vi "输出数据解析.vi"(0 "主板引用":refnum<vi>, 1 "从板引用":refnum<vi>, 2 "板选择":enum16{"主板", "从板"}(ring), 3 "二维码信息":refnum<vi>, 5 "错误代码":i32, 7 "命令序号":u8, 9 "输入数组":u8[](array[numeric]), 11 "命令":u8 format="%x", 12 "进度引用":refnum<vi>, 13 "从板个数":refnum<vi>, 14 "从板二维码信息":refnum<vi>) -> (4 "从板数":u8, 10 "序号":u8, 15 "状态":bool)   [LabVIEW 2013]
panel:
  in  "从板个数 2":dbl=1.0
  out "子字符串之前":string
  out "从板信息":T1
  out "主板数据 2":T2
  out "充电控制参数":bool
  out "二级故障1 2":bool
  out "一级故障1 6":bool
  out "一级故障1 5":bool
  out "二级故障1":bool
  out "一级故障5":bool
  out "一级故障1 4":bool
  out "一级故障1 3":bool
  out "一级故障1 2":bool
  out "一级故障1":bool
  in  "Ctl引用句柄":refnum<vi>
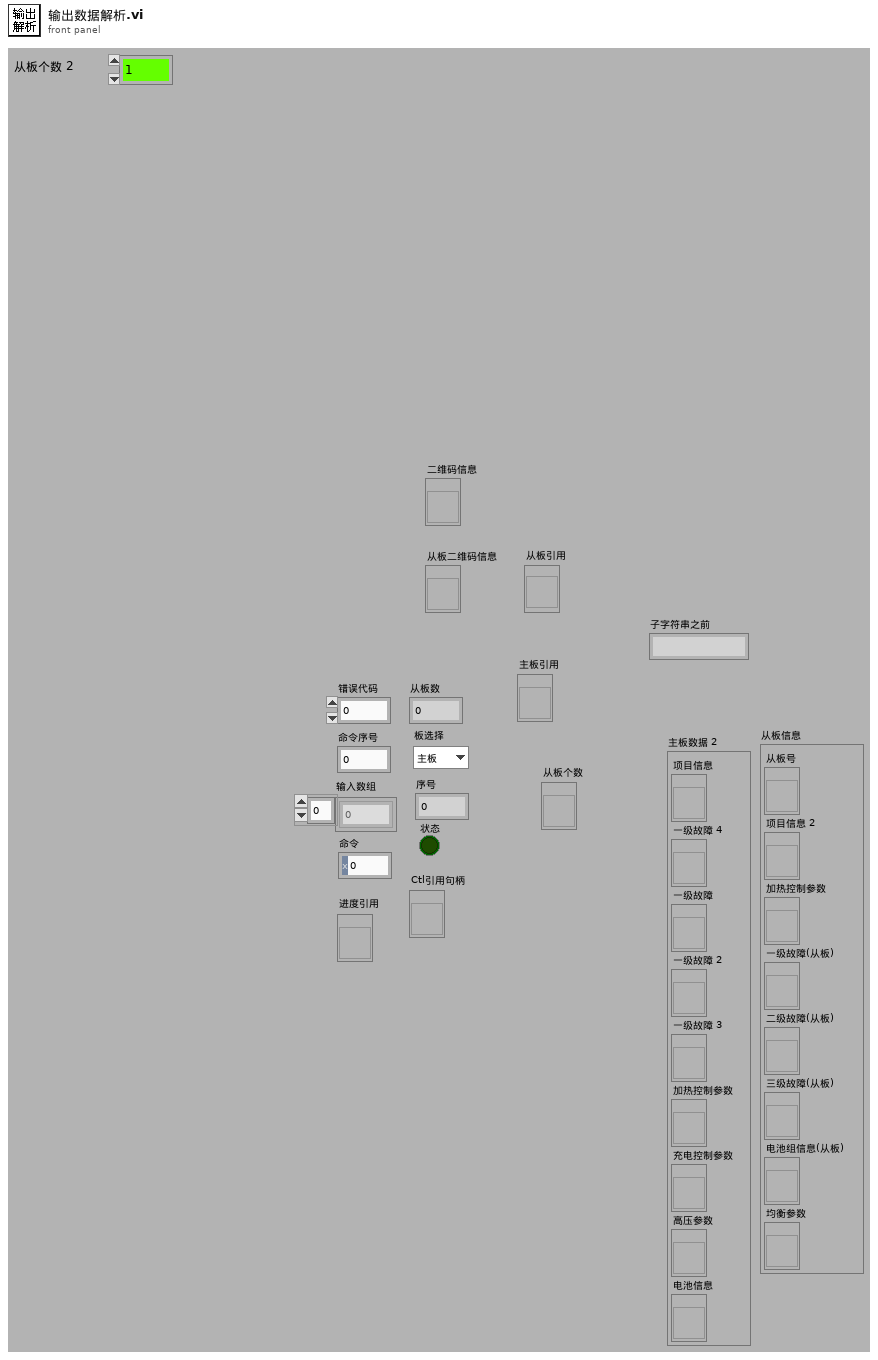
[diagram p1: front panel]
types:
  T1 = cluster{"从板号":refnum<vi>, "项目信息 2":refnum<vi>, "加热控制参数":refnum<vi>, "一级故障(从板)":refnum<vi>, "二级故障(从板)":refnum<vi>, "三级故障(从板)":refnum<vi>, "电池组信息(从板)":refnum<vi>, "均衡参数":refnum<vi>}
  T2 = cluster{"项目信息":refnum<vi>, "一级故障 4":refnum<vi>, "一级故障":refnum<vi>, "一级故障 2":refnum<vi>, "一级故障 3":refnum<vi>, "加热控制参数":refnum<vi>, "充电控制参数":refnum<vi>, "高压参数":refnum<vi>, "电池信息":refnum<vi>}
  T3 = cluster{"电池额定容量":dbl, "使用者":dbl, "电池实际容量":dbl, "车牌号":string, "配置文件版本":string, "SOH":dbl, "SOC":dbl, "产品编号":string, "系统时钟":string}
  T4 = cluster{"电池额定容量(A)":dbl, "使用者":dbl, "电池实际容量(A)":dbl, "车架(牌)号":string, "配置文件版本":string, "SOH(%)":dbl, "SOC(%)":dbl, "产品编号":string, "系统时钟":string}
  T5 = cluster{"总电压过高":dbl, "整组电压不均衡":dbl, "SOC过高":dbl, "单体电压过高":dbl, "总电压过低":dbl, "温度过高":dbl, "温度过低":dbl, "单组电压不均衡":dbl, "整组温度不均衡":dbl, "单组温度不均衡":dbl, "单体电压过低":dbl, "充电电流过高":dbl, "放电电流过高":dbl, "SOC过低":dbl, "内阻过大":dbl, "极柱温度过高":dbl, "SOH过低":dbl}
  T6 = cluster{"风机开启温度":dbl, "风机关闭温度":dbl, "加热开启温度":dbl, "加热关闭温度":dbl, "风机开启温差":dbl, "风机关闭温差":dbl, "加热关闭温差":dbl}
  T7 = cluster{"最大允许单体电压":dbl, "最大允许总电压":dbl, "最小允许单体电压":dbl, "最大允许充电电流":dbl, "最小允许充电电流":dbl, "最大允许充电温度":dbl, "最小允许充电温度":dbl, "电流步长":dbl}
  T8 = cluster{"充电能量阀值":dbl, "放电能量阀值":dbl, "电流增益":dbl, "平均电流":dbl, "电压增益":dbl, "平均电压":dbl}
  T9 = cluster{"电池串联":dbl, "电池并联":dbl, "累计放电总安时":dbl, "电池包额定容量":dbl, "电池包额定能量":dbl, "电池包额定总电压":dbl, "累计充电总安时":dbl, "电池充满次数":dbl, "电池放空次数":dbl, "电池充电次数":dbl, "电池生产日期":string, "电池厂家":string, "电池类型":string, "电池包组号":string, "电池包产权标识":string, "电池应用车型":string, "实际容量":dbl}
  T10 = cluster{"电压过高":dbl, "电压过低":dbl, "温度过高":dbl, "温度过低":dbl, "电压不均衡(V)":dbl, "温度不均衡":dbl, "SOC过低":dbl}
  T11 = cluster{"串联数":dbl, "并联数":dbl, "电池厂家":dbl, "电池类型":dbl, "额定能量":dbl, "额定容量":dbl, "实际容量":dbl, "额定总压":dbl, "产权标识":dbl, "应用车型":dbl, "电池包组号":dbl, "SOC":dbl, "充电总安时":dbl, "放电总这时":dbl, "放空次数":dbl, "充满次数":dbl, "充电次数":dbl, "车牌号":string, "生产日期":string, "最大允许单体电压":dbl, "最大允许总电压":dbl, "最大允许温度":dbl, "最小允许温度":dbl, "最大允许充电电流":dbl, "最小允许充电电流":dbl, "最小允许单体电压":dbl, "电流步长":dbl, "电池包序号":dbl}
  T12 = cluster{"充电结束电压(90%)":sgl, "充电结束电压(91%)":sgl, "充电结束电压(92%)":sgl, "充电结束电压(93%)":sgl, "充电结束电压(94%)":sgl, "均衡计算-电压高阀值1级":sgl, "均衡计算-电压高阀值2级":sgl, "均衡计算-电压低阀值1级":sgl, "均衡计算-电压低阀值2级":sgl, "均衡计算-最低电压阀值":sgl, "均衡停止-最低电压阀值":sgl, "均衡计算-电压极差阀值":sgl, "充电结束电压(95%)":sgl, "充电结束电压(96%)":sgl, "充电结束电压(97%)":sgl, "充电结束电压(98%)":sgl, "充电结束电压(99%)":sgl, "充电结束电压(100%)":sgl}
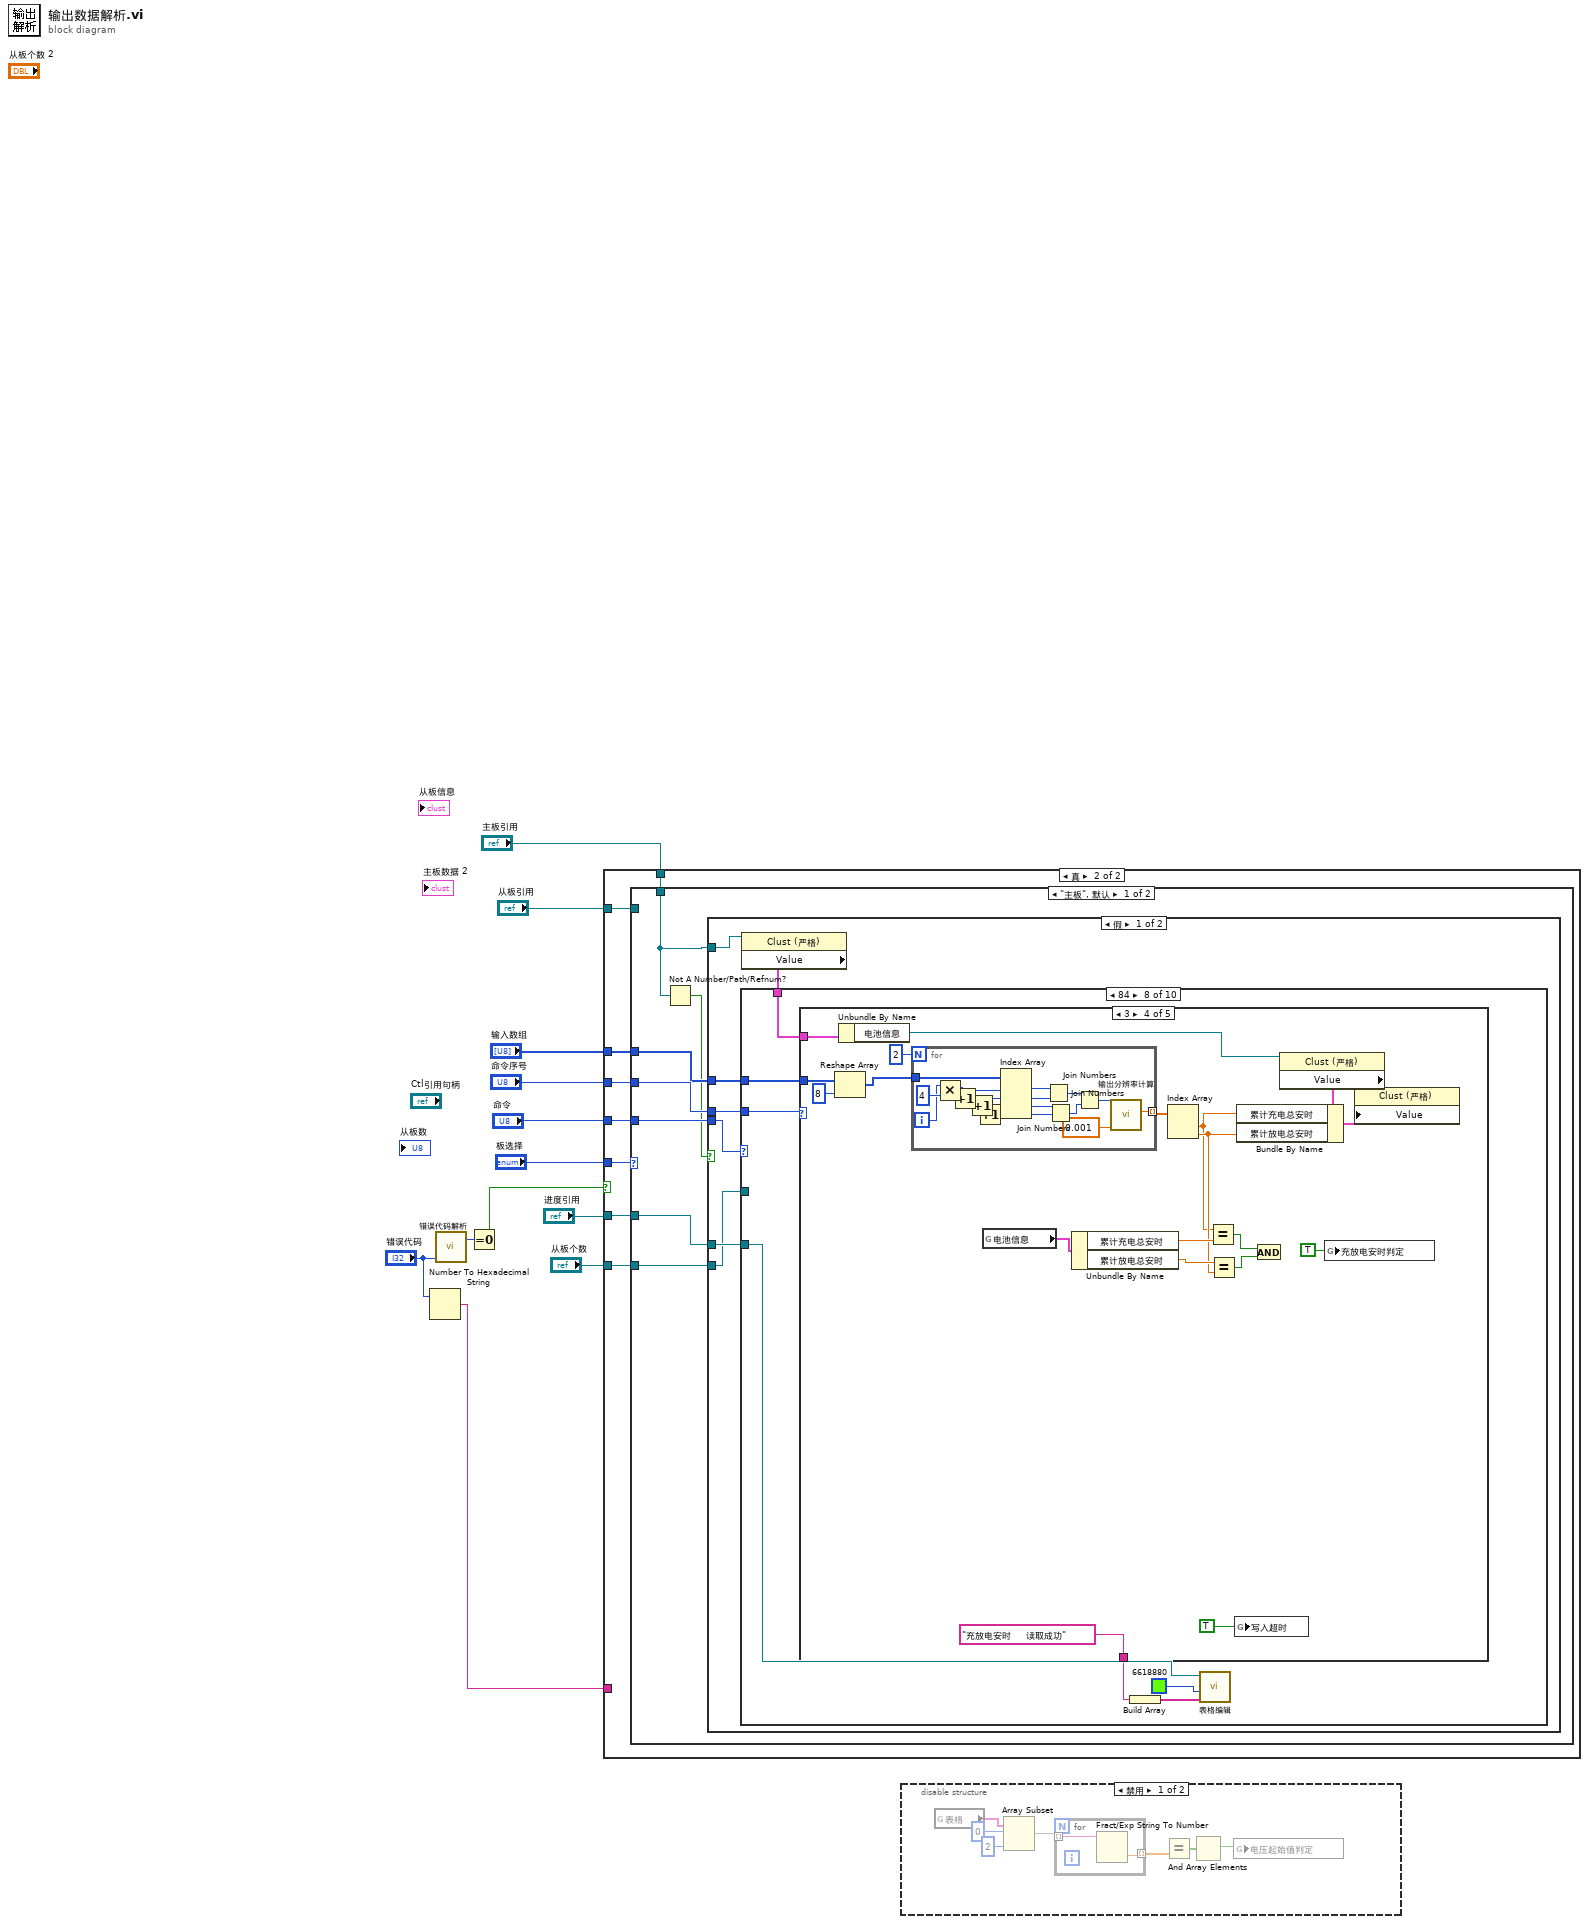
[diagram p0: block diagram]
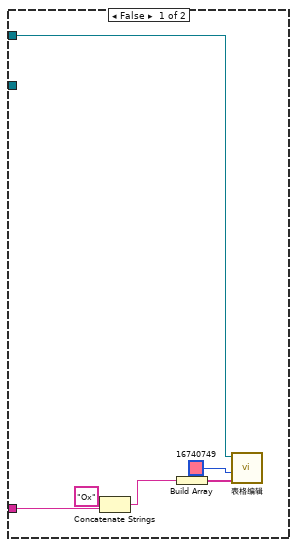
[diagram p3: hidden frame]
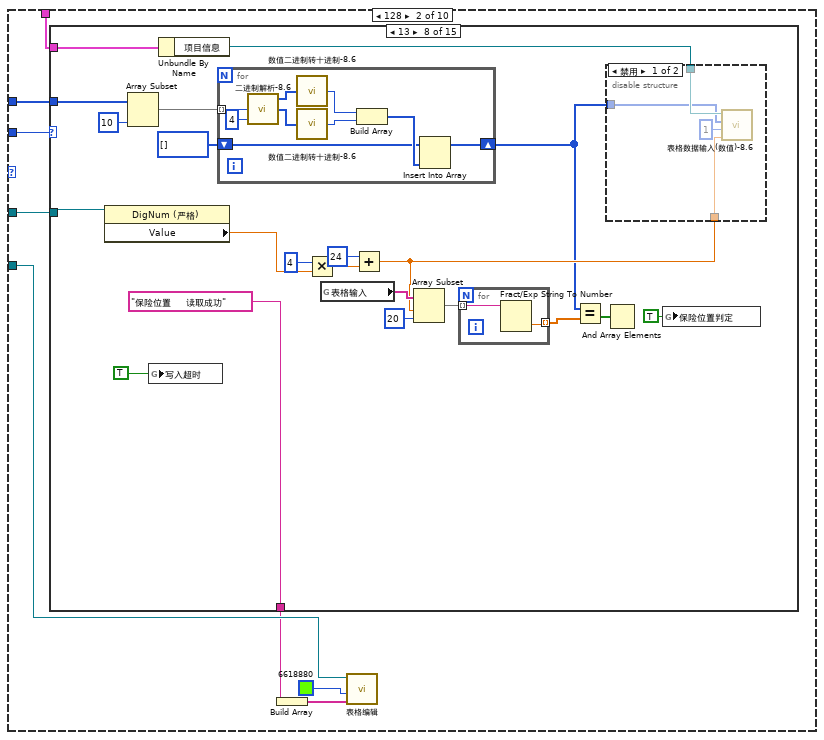
[diagram p5: hidden frame]
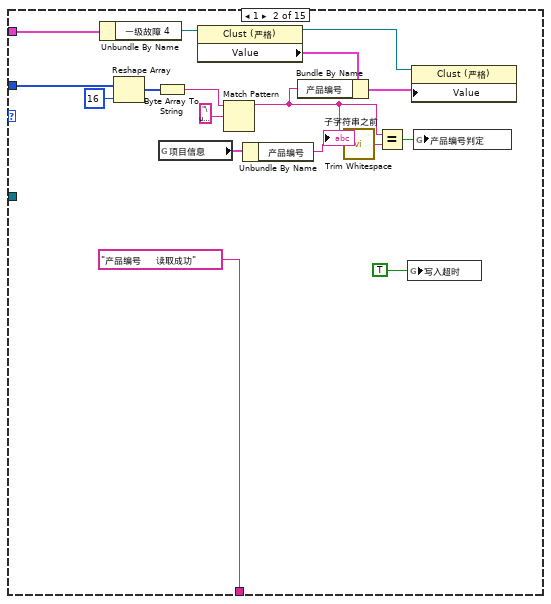
[diagram p7: hidden frame]
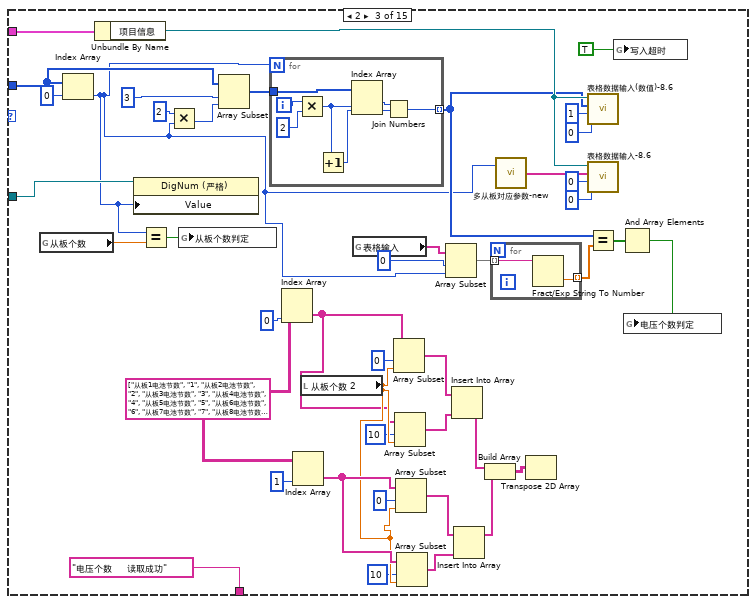
[diagram p8: hidden frame]
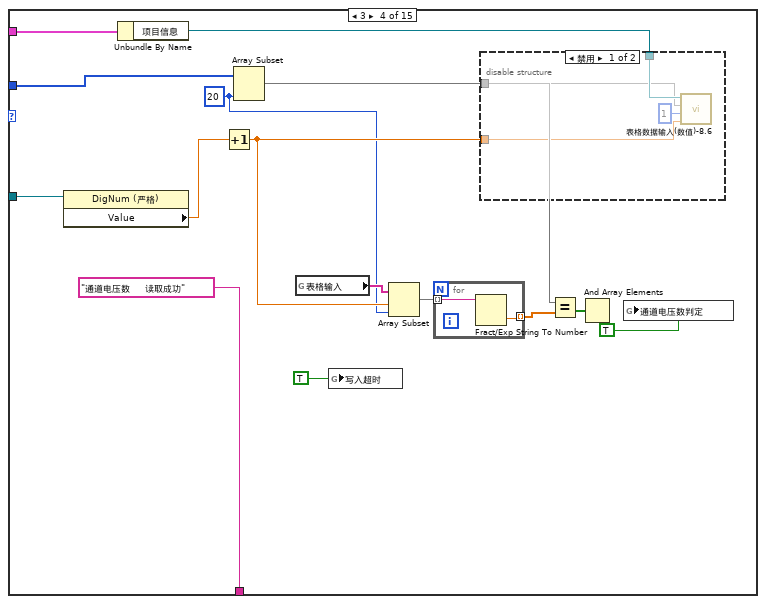
[diagram p9: hidden frame]
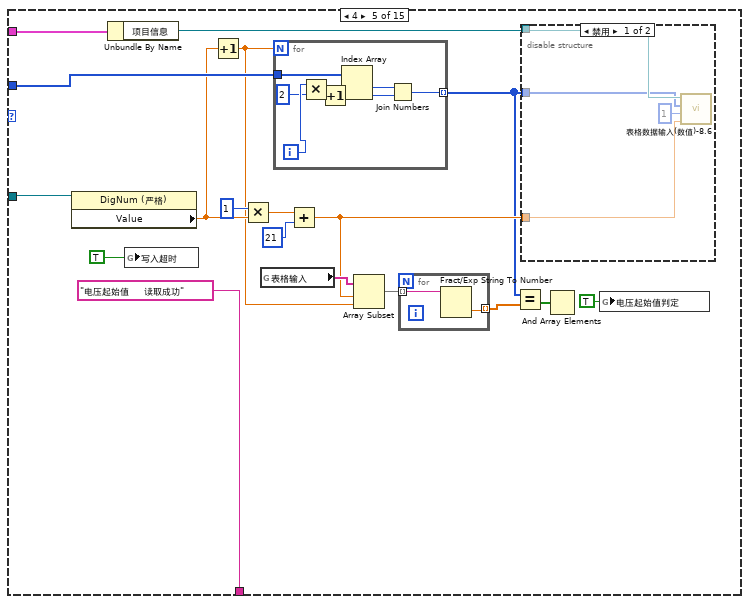
[diagram p11: hidden frame]
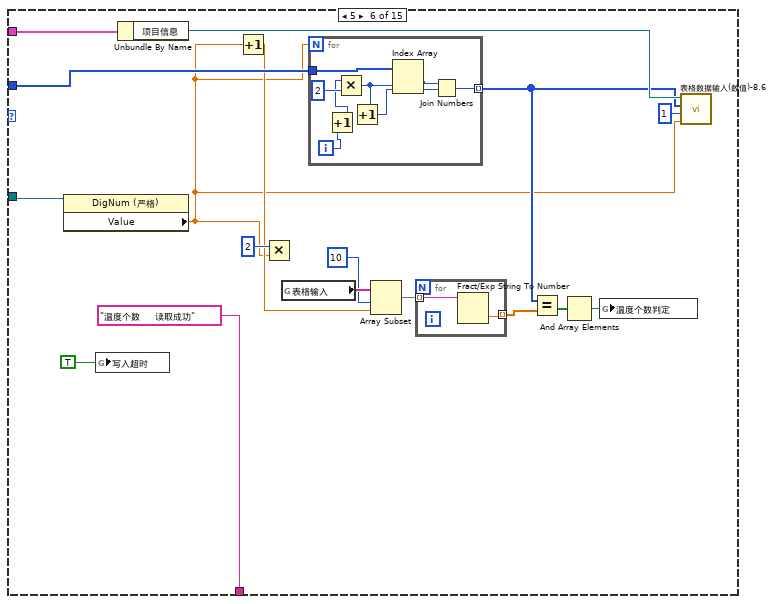
[diagram p13: hidden frame]
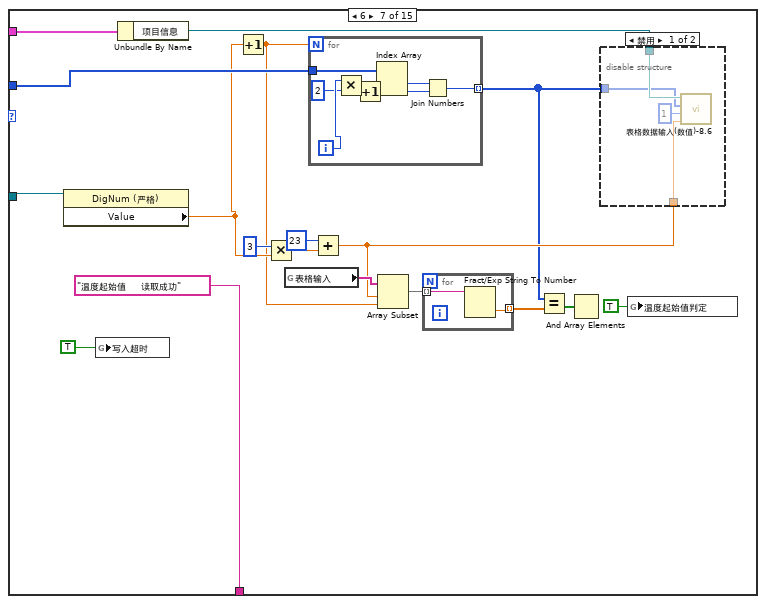
[diagram p14: hidden frame]
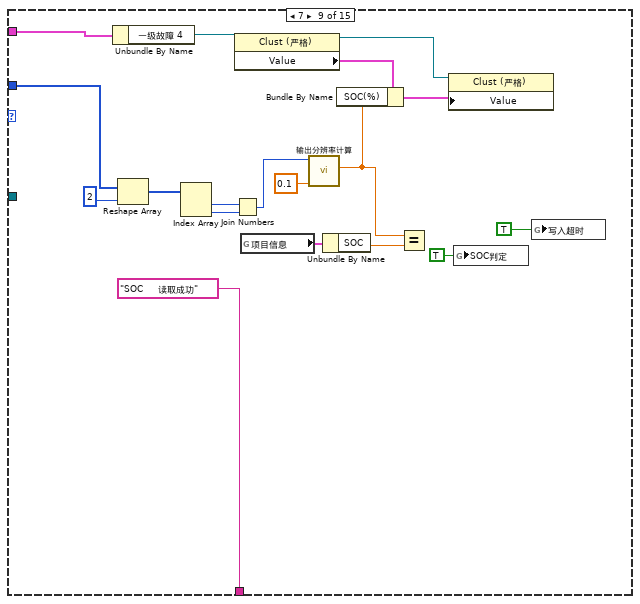
[diagram p17: hidden frame]
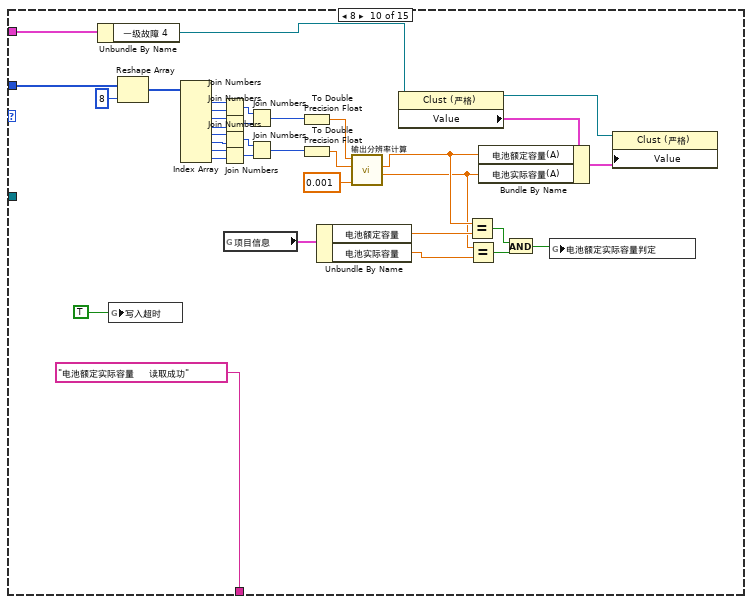
[diagram p18: hidden frame]
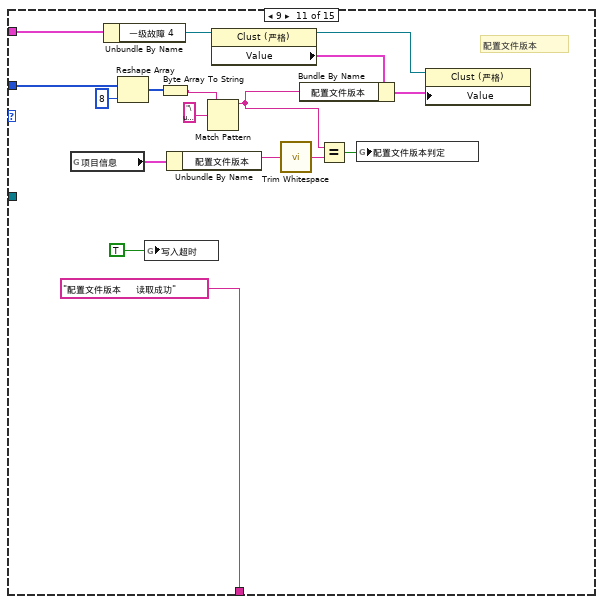
[diagram p19: hidden frame]
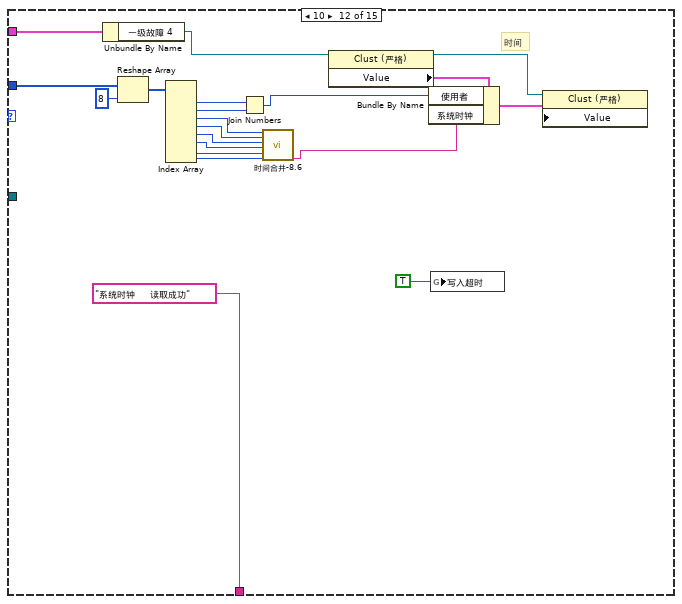
[diagram p20: hidden frame]
diagram:
  n1 = Number To Hexadecimal String(2:"错误代码") -> (0:w2:string)  [unwired: 1 out]
  n2 = call "错误代码解析.vi"("错误代码"="错误代码") -> ("错误代码"=w12:i32)  [unwired: 2 out]
  n3 = Equal To 0?(x=w12) -> (x = 0?=w11:bool)
  n4 = case shown="真" w11 {
    tunnel: "命令" -> [_ w26]
    tunnel: "命令序号" -> [_ w25]
    tunnel: "输入数组" -> [_ w24]
    tunnel: "板选择" -> [_ w23]
    tunnel: "主板引用" -> [_ w22]
    tunnel: "从板引用" -> [_ w21]
    tunnel: "进度引用" -> [w14 w20]
    tunnel: w2 -> [w17 _]
    tunnel: "从板个数" -> [_ w19]
    frame False {
      n5 = Concatenate Strings("Ox" ("字符串"), w17) -> (w16:string)
      n6 = Build Array(w16) -> (w15:string[])
      n7 = call "表格编辑.vi"("新元素/子数组"=w15, "活动单元格:单元格背景色"=u32 16740749, "MCListbox引用句柄"=w14) -> ()  [unwired: 9 out]
    }
    frame True {
      n8 = case shown="\"主板\", 默认" w23 {
        tunnel: w26 -> [w33 w1787]
        tunnel: w25 -> [w32 w1786]
        tunnel: w24 -> [w31 w1785]
        tunnel: w22 -> [w28 _]
        tunnel: w21 -> [_ w1783]
        tunnel: w20 -> [w30 w1784]
        tunnel: w19 -> [w27 _]
        frame "主板", Default {
          n9 = Not A Number/Path/Refnum?(number/path/refnum=w28) -> (NaN/Path/Refnum?=w29:bool)
          n10 = case shown="假" w29 {
            tunnel: w33 -> [w40 _]
            tunnel: w32 -> [w39 _]
            tunnel: w31 -> [w38 _]
            tunnel: w28 -> [w37 _]
            tunnel: w30 -> [w35 _]
            tunnel: w27 -> [w34 _]
            frame False {
              n11 = property class="Clust (严格)"(reference=w37) -> ("Value"=w36:T2)  [unwired: 1 in, 2 out]
              n12 = case shown="84" w40 {
                tunnel: w39 -> [_ w48 w413 w1115 w1300 w1346 w1388 w1560 _ _]
                tunnel: w38 -> [_ w47 w412 w1114 w1299 w1345 w1387 w1559 w1769 w1780]
                tunnel: w36 -> [_ w46 w411 w1113 w1298 w1344 _ w1558 _ _]
                tunnel: w35 -> [_ w44 w410 w1112 w1297 w1343 _ w1555 _ w1773]
                tunnel: w34 -> [_ w42 _ _ _ _ _ _ _ _]
                frame 0, Default {
                }
                frame 128 {
                  n13 = case shown="13" w48 {
                    tunnel: w47 -> [_ w65 w100 w133 w152 w184 w212 w243 w285 w320 w337 w357 w374 w391 w407]
                    tunnel: w46 -> [_ w62 w102 w132 w155 w186 w215 w250 w282 w317 w334 w351 w368 w385 w402]
                    tunnel: w42 -> [_ _ w97 w130 w151 w183 w211 w247 _ _ _ _ _ _ _]
                    tunnel: [_ "产品编号     读取成功" ("字符串") "电压个数     读取成功" ("字符串") "通道电压数     读取成功" ("字符串") "电压起始值     读取成功" ("字符串") "温度个数     读取成功" ("字符串") "温度起始值     读取成功" ("字符串") "保险位置     读取成功" ("字符串") "SOC     读取成功" ("字符串") "电池额定实际容量     读取成功" ("字符串") "配置文件版本     读取成功" ("字符串") "系统时钟     读取成功" ("字符串") "校正时钟     读取成功" ("字符串") "车牌号     读取成功" ("字符串") "SOH     读取成功" ("字符串")] -> w41
                    frame 0, Default {
                    }
                    frame 1 {
                      n14 = Unbundle By Name(w62) -> ("一级故障 4"=w61:refnum<vi>)
                      n15 = Reshape Array(w65, 16 ("维数大小")) -> (w64:u8[])
                      n16 = Byte Array To String(unsigned byte array=w64) -> (string=w50:string)
                      n17 = global read "读配置文件全局.vi" "项目信息"() -> (w56:T3)
                      n18 = property class="Clust (严格)"(reference=w61) -> (reference out=w59:refnum<vi>, "Value"=w60:T4)  [unwired: 1 in, 1 out]
                      n19 = Match Pattern(string=w50, regular expression="\u0000" ("trimmed string")) -> (before substring=w49:string)  [unwired: 1 in, 3 out]
                      "子字符串之前" <- w49
                      n20 = Unbundle By Name(w56) -> ("产品编号"=w54:string)
                      n21 = Bundle By Name(cluster=w60, "产品编号"=w49) -> (w55:T4)
                      n22 = call <vilib>:"Trim Whitespace.vi"("string"=w54) -> ("trimmed string"=w52:string)  [unwired: 1 in]
                      n23 = Equal?(x=w49, y=w52) -> (x = y?=w53:bool)
                      n24 = global write "EV05全局变量1.vi" "写入超时"(TRUE ("写入超时")) -> ()
                      n25 = property class="Clust (严格)"(reference=w59, "Value"=w55) -> ()  [unwired: 1 in, 2 out]
                      n26 = global write "读配置文件全局.vi" "产品编号判定"(w53) -> ()
                    }
                    frame 2 {
                      w74 = string[][] [["从板1电池节数", "1"], ["从板2电池节数", "2"], ["从板3电池节数", "3"], ["从板4电池节数", "4"], ["从板5电池节数", "5"], ["从板6电池节数", "6"], ["从板7电池节数", "7"], ["从板8电池节数", "8"], ["从板9电池节数", "9"], ["从板10电池节数", "10"], ["从板1温度个数", "1"], ["从板2温度个数", "2"], ["从板3温度个数", "3"], ["从板4温度个数", "4"], ["从板5温度个数", "5"], ["从板6温度个数", "6"], ["从板7温度个数", "7"], ["从板8温度个数", "8"], ["从板9温度个数", "9"], ["从板10温度个数", "10"]] ("项目信息")
                      n27 = global read "读配置文件全局.vi" "从板个数"() -> (w94:dbl)
                      n28 = Index Array(array=w100, index=0 ("索引")) -> (element=w67:u8)
                      n29 = Unbundle By Name(w102) -> ("项目信息"=w101:refnum<vi>)
                      n30 = property class="DigNum (严格)"(reference=w97, "Value"=w67) -> ()  [unwired: 1 in, 2 out]
                      n31 = Equal?(x=w67, y=w94) -> (x = y?=w93:bool)
                      n32 = Multiply(x=u8 2, y=w67) -> (x*y=w85:u8)
                      n33 = global write "读配置文件全局.vi" "从板个数判定"(w93) -> ()
                      n34 = Array Subset(array=w100, index=u8 3 ("y"), length=w85) -> (w99:u8[])
                      n35 = for {
                        N: w67 -> [_]
                        tunnel: w99 -> [w118]
                        tunnel: [w111] -> w88 mode=indexing
                        i -> [w117]
                        n36 = Multiply(x=w117, y=2) -> (x*y=w115:i32)
                        n37 = Increment(x=w115) -> (x+1=w114:i32)
                        n38 = Index Array(array=w118, index #1=w115, index #2=w114) -> (element #1=w112:u8, element #2=w113:u8)
                        n39 = Join Numbers(hi=w112, lo=w113) -> ((hi.lo)=w111:u16)
                      }
                      n40 = Index Array(array=w74, index (col)=0 ("索引 (行)")) -> (element=w71:string[])  [unwired: 1 in]
                      n41 = Index Array(array=w74, index (col)=1 ("禁用的索引 (列)")) -> (element=w81:string[])  [unwired: 1 in]
                      n42 = local read "从板个数 2"() -> (w79:dbl)
                      n43 = global read "读配置文件全局.vi" "表格输入"() -> (w92:string[])
                      n44 = Array Subset(array=w71, index=0 ("索引"), length=w79) -> (w72:string[])
                      n45 = Array Subset(array=w71, index=10 ("索引"), length=w79) -> (w73:string[])
                      n46 = Array Subset(array=w81, index=0 ("索引"), length=w79) -> (w75:string[])
                      n47 = Array Subset(array=w81, index=10 ("索引"), length=w79) -> (w80:string[])
                      n48 = Array Subset(array=w92, index=0 ("索引"), length=w67) -> (w90:string[])
                      n49 = Insert Into Array(array=w72, new element=w73) -> (w82:string[])  [unwired: 1 in]
                      n50 = Insert Into Array(array=w75, new element=w80) -> (w83:string[])  [unwired: 1 in]
                      n51 = Build Array(w82, w83) -> (w84:string[][])
                      n52 = for {
                        tunnel: w90 -> [w110] mode=indexing
                        tunnel: [w109] -> w89 mode=indexing
                        n53 = Fract/Exp String To Number(string=w110) -> (number=w109:dbl)  [unwired: 4 out]
                      }
                      n54 = call "多从板对应参数-new.vi"("从板个数"=w67) -> ("输出数组"=w105:string[])  [unwired: 1 in]
                      n55 = Transpose 2D Array(2D array=w84) -> ()  [unwired: 1 out]
                      n56 = call "表格数据输入(数值)-8.6.vi"("行数"=u32 0, "列数"=u32 1, "数值数组"=w88, "表格引用"=w101) -> ()  [unwired: 8 out]
                      n57 = call "表格数据输入-8.6.vi"("行数"=u32 0, "列数"=u32 0, "字符串数组"=w105, "表格引用"=w101) -> ()  [unwired: 8 out]
                      n58 = Equal?(x=w88, y=w89) -> (x = y?=w87:bool[])
                      n59 = global write "EV05全局变量1.vi" "写入超时"(TRUE ("写入超时")) -> ()
                      n60 = And Array Elements(Boolean array=w87) -> (logical AND=w86:bool)
                      n61 = global write "读配置文件全局.vi" "电压个数判定"(w86) -> ()
                    }
                    frame 3 {
                      w123 = 20 ("长度")
                      n62 = property class="DigNum (严格)"(reference=w130) -> ("Value"=w129:dbl)  [unwired: 1 in, 2 out]
                      n63 = Unbundle By Name(w132) -> ("项目信息"=w131:refnum<vi>)
                      n64 = Increment(x=w129) -> (x+1=w124:dbl)
                      n65 = Array Subset(array=w133, length=w123) -> (w121:u8[])  [unwired: 1 in]
                      n66 = global read "读配置文件全局.vi" "表格输入"() -> (w126:string[])
                      n67 = global write "EV05全局变量1.vi" "写入超时"(TRUE ("写入超时")) -> ()
                      n68 = Array Subset(array=w126, index=w124, length=w123) -> (w125:string[])
                      n69 = for {
                        tunnel: w125 -> [w139] mode=indexing
                        tunnel: [w138] -> w122 mode=indexing
                        n70 = Fract/Exp String To Number(string=w139) -> (number=w138:dbl)  [unwired: 4 out]
                      }
                      n71 = disable-structure shown="禁用" {
                        disable-tunnel: w131 -> [w136 _]
                        disable-tunnel: w124 -> [w135 _]
                        disable-tunnel: w121 -> [w134 _]
                        frame Disabled {
                          n72 = call "表格数据输入(数值)-8.6.vi"("行数"=w135, "列数"=u32 1, "数值数组"=w134, "表格引用"=w136) -> ()  [unwired: 8 out]
                        }
                        frame Enabled {
                        }
                      }
                      n73 = Equal?(x=w121, y=w122) -> (x = y?=w120:bool[])
                      n74 = And Array Elements(Boolean array=w120) -> ()  [unwired: 1 out]
                      n75 = global write "读配置文件全局.vi" "通道电压数判定"(TRUE ("通道电压数判定")) -> ()
                    }
                    frame 4 {
                      n76 = property class="DigNum (严格)"(reference=w151) -> ("Value"=w150:dbl)  [unwired: 1 in, 2 out]
                      n77 = Unbundle By Name(w155) -> ("项目信息"=w154:refnum<vi>)
                      n78 = global write "EV05全局变量1.vi" "写入超时"(TRUE ("写入超时")) -> ()
                      n79 = Increment(x=w150) -> (x+1=w142:dbl)
                      n80 = Multiply(x=u8 1, y=w150) -> (x*y=w156:dbl)
                      n81 = global read "读配置文件全局.vi" "表格输入"() -> (w147:string[])
                      n82 = for {
                        N: w142 -> [_]
                        tunnel: w152 -> [w171]
                        tunnel: [w164] -> w141 mode=indexing
                        i -> [w170]
                        n83 = Multiply(x=w170, y=2) -> (x*y=w168:i32)
                        n84 = Increment(x=w168) -> (x+1=w167:i32)
                        n85 = Index Array(array=w171, index #1=w168, index #2=w167) -> (element #1=w165:u8, element #2=w166:u8)
                        n86 = Join Numbers(hi=w165, lo=w166) -> ((hi.lo)=w164:u16)
                      }
                      n87 = Add(x=w156, y=u8 21) -> (x+y=w143:dbl)
                      n88 = Array Subset(array=w147, index=w143, length=w142) -> (w146:string[])
                      n89 = for {
                        tunnel: w146 -> [w163] mode=indexing
                        tunnel: [w162] -> w145 mode=indexing
                        n90 = Fract/Exp String To Number(string=w163) -> (number=w162:dbl)  [unwired: 4 out]
                      }
                      n91 = Equal?(x=w141, y=w145) -> (x = y?=w144:bool[])
                      n92 = disable-structure shown="禁用" {
                        disable-tunnel: w154 -> [w160 _]
                        disable-tunnel: w143 -> [w159 _]
                        disable-tunnel: w141 -> [w158 _]
                        frame Disabled {
                          n93 = call "表格数据输入(数值)-8.6.vi"("行数"=w159, "列数"=u32 1, "数值数组"=w158, "表格引用"=w160) -> ()  [unwired: 8 out]
                        }
                        frame Enabled {
                        }
                      }
                      n94 = And Array Elements(Boolean array=w144) -> ()  [unwired: 1 out]
                      n95 = global write "读配置文件全局.vi" "电压起始值判定"(TRUE ("电压起始值判定")) -> ()
                    }
                    frame 5 {
                      n96 = property class="DigNum (严格)"(reference=w183) -> ("Value"=w174:dbl)  [unwired: 1 in, 2 out]
                      n97 = global write "EV05全局变量1.vi" "写入超时"(TRUE ("写入超时")) -> ()
                      n98 = Unbundle By Name(w186) -> ("项目信息"=w185:refnum<vi>)
                      n99 = Increment(x=w174) -> (x+1=w176:dbl)
                      n100 = Multiply(x=u8 2, y=w174) -> ()  [unwired: 1 out]
                      n101 = global read "读配置文件全局.vi" "表格输入"() -> (w180:string[])
                      n102 = for {
                        N: w174 -> [_]
                        tunnel: w184 -> [w199]
                        tunnel: [w193] -> w175 mode=indexing
                        i -> [w192]
                        n103 = Increment(x=w192) -> (x+1=w191:i32)
                        n104 = Multiply(x=w191, y=2) -> (x*y=w197:i32)
                        n105 = Increment(x=w197) -> (x+1=w196:i32)
                        n106 = Index Array(array=w199, index #1=w197, index #2=w196) -> (element #1=w194:u8, element #2=w195:u8)
                        n107 = Join Numbers(hi=w194, lo=w195) -> ((hi.lo)=w193:u16)
                      }
                      n108 = Array Subset(array=w180, index=u8 10 ("x"), length=w176) -> (w179:string[])
                      n109 = for {
                        tunnel: w179 -> [w190] mode=indexing
                        tunnel: [w189] -> w178 mode=indexing
                        n110 = Fract/Exp String To Number(string=w190) -> (number=w189:dbl)  [unwired: 4 out]
                      }
                      n111 = Equal?(x=w175, y=w178) -> (x = y?=w177:bool[])
                      n112 = And Array Elements(Boolean array=w177) -> (logical AND=w172:bool)
                      n113 = global write "读配置文件全局.vi" "温度个数判定"(w172) -> ()
                      n114 = call "表格数据输入(数值)-8.6.vi"("行数"=w174, "列数"=u32 1, "数值数组"=w175, "表格引用"=w185) -> ()  [unwired: 8 out]
                    }
                    frame 6 {
                      n115 = property class="DigNum (严格)"(reference=w211) -> ("Value"=w210:dbl)  [unwired: 1 in, 2 out]
                      n116 = global write "EV05全局变量1.vi" "写入超时"(TRUE ("写入超时")) -> ()
                      n117 = Unbundle By Name(w215) -> ("项目信息"=w214:refnum<vi>)
                      n118 = Increment(x=w210) -> (x+1=w202:dbl)
                      n119 = Multiply(x=u8 3, y=w210) -> (x*y=w216:dbl)
                      n120 = global read "读配置文件全局.vi" "表格输入"() -> (w207:string[])
                      n121 = for {
                        N: w202 -> [_]
                        tunnel: w212 -> [w231]
                        tunnel: [w224] -> w201 mode=indexing
                        i -> [w230]
                        n122 = Multiply(x=w230, y=2) -> (x*y=w228:i32)
                        n123 = Increment(x=w228) -> (x+1=w227:i32)
                        n124 = Index Array(array=w231, index #1=w228, index #2=w227) -> (element #1=w225:u8, element #2=w226:u8)
                        n125 = Join Numbers(hi=w225, lo=w226) -> ((hi.lo)=w224:u16)
                      }
                      n126 = Add(x=u8 23, y=w216) -> (x+y=w203:dbl)
                      n127 = Array Subset(array=w207, index=w203, length=w202) -> (w206:string[])
                      n128 = for {
                        tunnel: w206 -> [w223] mode=indexing
                        tunnel: [w222] -> w205 mode=indexing
                        n129 = Fract/Exp String To Number(string=w223) -> (number=w222:dbl)  [unwired: 4 out]
                      }
                      n130 = Equal?(x=w201, y=w205) -> (x = y?=w204:bool[])
                      n131 = And Array Elements(Boolean array=w204) -> ()  [unwired: 1 out]
                      n132 = disable-structure shown="禁用" {
                        disable-tunnel: w214 -> [w220 _]
                        disable-tunnel: w203 -> [w219 _]
                        disable-tunnel: w201 -> [w218 _]
                        frame Disabled {
                          n133 = call "表格数据输入(数值)-8.6.vi"("行数"=w219, "列数"=u32 1, "数值数组"=w218, "表格引用"=w220) -> ()  [unwired: 8 out]
                        }
                        frame Enabled {
                        }
                      }
                      n134 = global write "读配置文件全局.vi" "温度起始值判定"(TRUE ("温度起始值判定")) -> ()
                    }
                    frame 13 {
                      n135 = property class="DigNum (严格)"(reference=w247) -> ("Value"=w246:dbl)  [unwired: 1 in, 2 out]
                      n136 = Array Subset(array=w243, length=10 ("长度")) -> (w235:u8[])  [unwired: 1 in]
                      n137 = global write "EV05全局变量1.vi" "写入超时"(TRUE ("写入超时")) -> ()
                      n138 = Unbundle By Name(w250) -> ("项目信息"=w249:refnum<vi>)
                      n139 = for {
                        tunnel: w235 -> [w265] mode=indexing
                        shift-right: [w258] -> w234
                        shift-left: i32[] [] -> [w257]
                        n140 = call "二进制解析-8.6.vi"("索引"=4, "数值"=w265) -> ("低位子数组"=w263:i32[], "高位子数组"=w262:i32[])  [unwired: 1 in, 1 out]
                        n141 = call "数值二进制转十进制-8.6.vi"("子数组"=w262) -> ("十进制数值"=w261:i32)  [unwired: 4 in]
                        n142 = call "数值二进制转十进制-8.6.vi"("子数组"=w263) -> ("十进制数值"=w260:i32)  [unwired: 4 in]
                        n143 = Build Array(w261, w260) -> (w259:i32[])
                        n144 = Insert Into Array(array=w257, new element=w259) -> (w258:i32[])  [unwired: 1 in]
                      }
                      n145 = Multiply(x=u8 4, y=w246) -> (x*y=w251:dbl)
                      n146 = global read "读配置文件全局.vi" "表格输入"() -> (w241:string[])
                      n147 = Add(x=u8 24, y=w251) -> (x+y=w237:dbl)
                      n148 = Array Subset(array=w241, index=w237, length=20 ("长度")) -> (w240:string[])
                      n149 = for {
                        tunnel: w240 -> [w267] mode=indexing
                        tunnel: [w266] -> w239 mode=indexing
                        n150 = Fract/Exp String To Number(string=w267) -> (number=w266:dbl)  [unwired: 4 out]
                      }
                      n151 = Equal?(x=w234, y=w239) -> (x = y?=w238:bool[])
                      n152 = disable-structure shown="禁用" {
                        disable-tunnel: w249 -> [w255 _]
                        disable-tunnel: w237 -> [w254 _]
                        disable-tunnel: w234 -> [w253 _]
                        frame Disabled {
                          n153 = call "表格数据输入(数值)-8.6.vi"("行数"=w254, "列数"=u32 1, "数值数组"=w253, "表格引用"=w255) -> ()  [unwired: 8 out]
                        }
                        frame Enabled {
                        }
                      }
                      n154 = And Array Elements(Boolean array=w238) -> ()  [unwired: 1 out]
                      n155 = global write "读配置文件全局.vi" "保险位置判定"(TRUE ("保险位置判定")) -> ()
                    }
                    frame 7 {
                      n156 = Unbundle By Name(w282) -> ("一级故障 4"=w278:refnum<vi>)
                      n157 = Reshape Array(w285, 2 ("维数大小")) -> (w283:u8[])
                      n158 = Index Array(array=w283) -> (element #1=w275:u8, element #2=w274:u8)  [unwired: 2 in]
                      n159 = Join Numbers(hi=w275, lo=w274) -> ((hi.lo)=w273:u16)
                      n160 = property class="Clust (严格)"(reference=w278) -> (reference out=w280:refnum<vi>, "Value"=w281:T4)  [unwired: 1 in, 1 out]
                      n161 = global read "读配置文件全局.vi" "项目信息"() -> (w271:T3)
                      n162 = call "输出分辨率计算.vi"("分辨率"=0.1, "数值 2"=w273) -> ("输出2"=w269:dbl)  [unwired: 4 in, 5 out]
                      n163 = Unbundle By Name(w271) -> ("SOC"=w270:dbl)
                      n164 = Bundle By Name(cluster=w281, "SOC(%)"=w269) -> (w279:T4)
                      n165 = Equal?(x=w269, y=w270) -> ()  [unwired: 1 out]
                      n166 = property class="Clust (严格)"(reference=w280, "Value"=w279) -> ()  [unwired: 1 in, 2 out]
                      n167 = global write "读配置文件全局.vi" "SOC判定"(TRUE ("SOC判定")) -> ()
                      n168 = global write "EV05全局变量1.vi" "写入超时"(TRUE ("写入超时")) -> ()
                    }
                    frame 8 {
                      n169 = Unbundle By Name(w317) -> ("一级故障 4"=w313:refnum<vi>)
                      n170 = global write "EV05全局变量1.vi" "写入超时"(TRUE ("写入超时")) -> ()
                      n171 = Reshape Array(w320, 8 ("维数大小")) -> (w318:u8[])
                      n172 = Index Array(array=w318) -> (element #1=w307:u8, element #2=w308:u8, element #3=w306:u8, element #4=w305:u8, element #5=w298:u8, element #6=w297:u8, element #7=w296:u8, element #8=w295:u8)  [unwired: 8 in]
                      n173 = Join Numbers(hi=w307, lo=w308) -> ((hi.lo)=w303:u16)
                      n174 = Join Numbers(hi=w306, lo=w305) -> ((hi.lo)=w304:u16)
                      n175 = Join Numbers(hi=w298, lo=w297) -> ((hi.lo)=w300:u16)
                      n176 = Join Numbers(hi=w296, lo=w295) -> ((hi.lo)=w299:u16)
                      n177 = global read "读配置文件全局.vi" "项目信息"() -> (w293:T3)
                      n178 = Join Numbers(hi=w303, lo=w304) -> ((hi.lo)=w302:u32)
                      n179 = Join Numbers(hi=w300, lo=w299) -> ((hi.lo)=w301:u32)
                      n180 = To Double Precision Float(number=w302) -> (double precision float=w309:dbl)
                      n181 = To Double Precision Float(number=w301) -> (double precision float=w294:dbl)
                      n182 = Unbundle By Name(w293) -> ("电池额定容量"=w291:dbl, "电池实际容量"=w289:dbl)
                      n183 = call "输出分辨率计算.vi"("分辨率"=0.001, "数值 3"=w294, "数值 2"=w309) -> ("输出3"=w290:dbl, "输出2"=w292:dbl)  [unwired: 3 in, 4 out]
                      n184 = property class="Clust (严格)"(reference=w313) -> (reference out=w315:refnum<vi>, "Value"=w316:T4)  [unwired: 1 in, 1 out]
                      n185 = Equal?(x=w292, y=w291) -> (x = y?=w287:bool)
                      n186 = Equal?(x=w290, y=w289) -> (x = y?=w288:bool)
                      n187 = Bundle By Name(cluster=w316, "电池额定容量(A)"=w292, "电池实际容量(A)"=w290) -> (w314:T4)
                      n188 = And(x=w287, y=w288) -> (x .and. y?=w286:bool)
                      n189 = global write "读配置文件全局.vi" "电池额定实际容量判定"(w286) -> ()
                      n190 = property class="Clust (严格)"(reference=w315, "Value"=w314) -> ()  [unwired: 1 in, 2 out]
                    }
                    frame 9 {
                      # "配置文件版本"
                      n191 = global read "读配置文件全局.vi" "项目信息"() -> (w327:T3)
                      n192 = Unbundle By Name(w334) -> ("一级故障 4"=w330:refnum<vi>)
                      n193 = Reshape Array(w337, 8 ("维数大小")) -> (w335:u8[])
                      n194 = global write "EV05全局变量1.vi" "写入超时"(TRUE ("写入超时")) -> ()
                      n195 = Byte Array To String(unsigned byte array=w335) -> (string=w322:string)
                      n196 = Unbundle By Name(w327) -> ("配置文件版本"=w326:string)
                      n197 = Match Pattern(string=w322, regular expression="\u0000" ("trimmed string")) -> (before substring=w321:string)  [unwired: 1 in, 3 out]
                      n198 = property class="Clust (严格)"(reference=w330) -> (reference out=w332:refnum<vi>, "Value"=w333:T4)  [unwired: 1 in, 1 out]
                      n199 = call <vilib>:"Trim Whitespace.vi"("string"=w326) -> ("trimmed string"=w325:string)  [unwired: 1 in]
                      n200 = Bundle By Name(cluster=w333, "配置文件版本"=w321) -> (w331:T4)
                      n201 = Equal?(x=w321, y=w325) -> (x = y?=w324:bool)
                      n202 = global write "读配置文件全局.vi" "配置文件版本判定"(w324) -> ()
                      n203 = property class="Clust (严格)"(reference=w332, "Value"=w331) -> ()  [unwired: 1 in, 2 out]
                    }
                    frame 10 {
                      # "时间"
                      n204 = Unbundle By Name(w351) -> ("一级故障 4"=w350:refnum<vi>)
                      n205 = Reshape Array(w357, 8 ("维数大小")) -> (w355:u8[])
                      n206 = Index Array(array=w355) -> (element #1=w341:u8, element #2=w342:u8, element #3=w343:u8, element #4=w344:u8, element #5=w345:u8, element #6=w346:u8, element #7=w347:u8, element #8=w348:u8)  [unwired: 8 in]
                      n207 = Join Numbers(hi=w341, lo=w342) -> ((hi.lo)=w340:u16)
                      n208 = call "时间合并-8.6.vi"("年"=w343, "月"=w344, "日"=w345, "时"=w346, "分"=w347, "秒"=w348) -> ("时间"=w349:string)  [unwired: 13 out]
                      n209 = property class="Clust (严格)"(reference=w350) -> (reference out=w353:refnum<vi>, "Value"=w354:T4)  [unwired: 1 in, 1 out]
                      n210 = Bundle By Name(cluster=w354, "使用者"=w340, "系统时钟"=w349) -> (w352:T4)
                      n211 = global write "EV05全局变量1.vi" "写入超时"(TRUE ("写入超时")) -> ()
                      n212 = property class="Clust (严格)"(reference=w353, "Value"=w352) -> ()  [unwired: 1 in, 2 out]
                    }
                    frame 14 {
                      n213 = Unbundle By Name(w368) -> ("一级故障 4"=w367:refnum<vi>)
                      n214 = Reshape Array(w374, 6 ("维数大小")) -> (w372:u8[])
                      n215 = Index Array(array=w372) -> (element #1=w363:u8, element #2=w362:u8, element #3=w361:u8, element #4=w360:u8, element #5=w359:u8, element #6=w358:u8)  [unwired: 6 in]
                      n216 = call "时间合并-8.6.vi"("年"=w363, "月"=w362, "日"=w361, "时"=w360, "分"=w359, "秒"=w358) -> ("时间"=w366:string)  [unwired: 13 out]
                      n217 = property class="Clust (严格)"(reference=w367) -> (reference out=w370:refnum<vi>, "Value"=w371:T4)  [unwired: 1 in, 1 out]
                      n218 = Bundle By Name(cluster=w371, "系统时钟"=w366) -> (w369:T4)
                      n219 = global write "EV05全局变量1.vi" "写入超时"(TRUE ("写入超时")) -> ()
                      n220 = property class="Clust (严格)"(reference=w370, "Value"=w369) -> ()  [unwired: 1 in, 2 out]
                    }
                    frame 11 {
                      # "车牌号"
                      n221 = Unbundle By Name(w385) -> ("一级故障 4"=w384:refnum<vi>)
                      n222 = Reshape Array(w391, 8 ("维数大小")) -> (w389:u8[])
                      n223 = global read "读配置文件全局.vi" "项目信息"() -> (w381:T3)
                      n224 = Byte Array To String(unsigned byte array=w389) -> (string=w377:string)
                      n225 = property class="Clust (严格)"(reference=w384) -> (reference out=w387:refnum<vi>, "Value"=w388:T4)  [unwired: 1 in, 1 out]
                      n226 = Unbundle By Name(w381) -> ("车牌号"=w380:string)
                      n227 = Match Pattern(string=w377, regular expression="\u0000" ("trimmed string")) -> (before substring=w376:string)  [unwired: 1 in, 3 out]
                      n228 = call <vilib>:"Trim Whitespace.vi"("string"=w380) -> ("trimmed string"=w379:string)  [unwired: 1 in]
                      n229 = Bundle By Name(cluster=w388, "车架(牌)号"=w376) -> (w386:T4)
                      n230 = Equal?(x=w376, y=w379) -> ()  [unwired: 1 out]
                      n231 = global write "读配置文件全局.vi" "车牌号判定"(TRUE ("车牌号判定")) -> ()
                      n232 = global write "EV05全局变量1.vi" "写入超时"(TRUE ("写入超时")) -> ()
                      n233 = property class="Clust (严格)"(reference=w387, "Value"=w386) -> ()  [unwired: 1 in, 2 out]
                    }
                    frame 12 {
                      # "SOH"
                      n234 = Unbundle By Name(w402) -> ("一级故障 4"=w401:refnum<vi>)
                      n235 = Reshape Array(w407, 2 ("维数大小")) -> (w408:u8[])
                      n236 = Index Array(array=w408) -> (element #1=w399:u8, element #2=w400:u8)  [unwired: 2 in]
                      n237 = Join Numbers(hi=w399, lo=w400) -> ((hi.lo)=w398:u16)
                      n238 = property class="Clust (严格)"(reference=w401) -> (reference out=w404:refnum<vi>, "Value"=w405:T4)  [unwired: 1 in, 1 out]
                      n239 = global read "读配置文件全局.vi" "项目信息"() -> (w395:T3)
                      n240 = Unbundle By Name(w395) -> ("SOH"=w393:dbl)
                      n241 = call "输出分辨率计算.vi"("分辨率"=0.1, "数值 2"=w398) -> ("输出2"=w394:dbl)  [unwired: 4 in, 5 out]
                      n242 = Equal?(x=w394, y=w393) -> ()  [unwired: 1 out]
                      n243 = Bundle By Name(cluster=w405, "SOH(%)"=w394) -> (w403:T4)
                      n244 = global write "读配置文件全局.vi" "SOH判定"(TRUE ("SOH判定")) -> ()
                      n245 = property class="Clust (严格)"(reference=w404, "Value"=w403) -> ()  [unwired: 1 in, 2 out]
                      n246 = global write "EV05全局变量1.vi" "写入超时"(TRUE ("写入超时")) -> ()
                    }
                  }
                  n247 = Build Array(w41) -> (w45:string[])
                  n248 = call "表格编辑.vi"("新元素/子数组"=w45, "活动单元格:单元格背景色"=u32 6618880, "MCListbox引用句柄"=w44) -> ()  [unwired: 9 out]
                }
                frame 129 {
                  n249 = case shown="0, 默认" w413 {
                    tunnel: w412 -> [_ w424 w658 w890]
                    tunnel: w411 -> [_ w420 w654 w886]
                    tunnel: w410 -> [_ w414 w650 w880]
                    frame 0, Default {
                    }
                    frame 1 {
                      n250 = Unbundle By Name(w420) -> ("一级故障"=w419:refnum<vi>)
                      n251 = Reshape Array(w424, 28 ("维数大小")) -> (w421:u8[])
                      n252 = for {
                        N: 4 -> [_]
                        tunnel: w421 -> [w446]
                        tunnel: w419 -> [w429]
                        i -> [w443]
                        n253 = case shown="0, 默认" w443 {
                          tunnel: [0 7 15 24] -> w442
                          tunnel: [1 8 16 25] -> w441
                          tunnel: [2 9 17 26] -> w440
                          tunnel: [3 10 18 27] -> w439
                          tunnel: [4 11 19 _] -> w438
                          tunnel: [5 12 20 27] -> w437
                          tunnel: [6 13 21 _] -> w436
                          tunnel: [w447 w455 22 _] -> w428
                          tunnel: [w447 w455 23 _] -> w427
                          frame 0, Default {
                            w447 = 0
                          }
                          frame 1 {
                            w455 = 14
                          }
                          frame 2 {
                          }
                          frame 3 {
                          }
                        }
                        n254 = global write "EV05全局变量1.vi" "写入超时"(TRUE ("写入超时")) -> ()
                        n255 = Index Array(array=w446, index #1=w442, index #2=w441, index #3=w440, index #4=w439, index #5=w438, index #6=w437, index #7=w436, index #8=w428, index #9=w427) -> (element #1=w445:u8, element #2=w444:u8, element #3=w435:u8, element #4=w434:u8, element #5=w433:u8, element #6=w432:u8, element #7=w431:u8, element #8=w430:u8, element #9=w426:u8)
                        n256 = case shown="0, 默认" w443 {
                          tunnel: w445 -> [w519 w563 w610 w636]
                          tunnel: w444 -> [w516 w562 w609 w642]
                          tunnel: w435 -> [w515 w560 w608 w639]
                          tunnel: w434 -> [w514 w559 w607 w638]
                          tunnel: w433 -> [w510 w558 w573 _]
                          tunnel: w432 -> [w509 w557 w600 _]
                          tunnel: w431 -> [w487 w556 w599 _]
                          tunnel: w430 -> [_ w555 w598 _]
                          tunnel: w429 -> [w505 w549 w603 w643]
                          tunnel: w426 -> [_ _ w597 _]
                          frame 0, Default {
                            n257 = global read "读配置文件全局.vi" "一级故障"() -> (w504:sgl[])
                            n258 = Join Numbers(hi=w519, lo=w516) -> ((hi.lo)=w518:u16)
                            n259 = Join Numbers(hi=w515, lo=w514) -> ((hi.lo)=w513:u16)
                            n260 = call "输出分辨率计算.vi"("偏移量"=sgl -40.0, "分辨率"=1.0, "数值 3"=w509, "数值 2"=w510) -> ("输出3"=w496:dbl, "输出2"=w498:dbl)  [unwired: 2 in, 4 out]
                            n261 = call "输出分辨率计算.vi"("分辨率"=0.1, "数值 3"=w513, "数值 2"=w518) -> ("输出3"=w500:dbl, "输出2"=w502:dbl)  [unwired: 3 in, 4 out]
                            n262 = Index Array(array=w504, index #5=6 ("索引")) -> (element #1=w501:sgl, element #2=w499:sgl, element #3=w497:sgl, element #4=w495:sgl, element #5=w494:sgl)  [unwired: 4 in]
                            n263 = To Single Precision Float(number=w502) -> (single precision float=w478:sgl)
                            n264 = To Single Precision Float(number=w501) -> (single precision float=w479:sgl)
                            n265 = To Single Precision Float(number=w500) -> (single precision float=w480:sgl)
                            n266 = To Single Precision Float(number=w499) -> (single precision float=w481:sgl)
                            n267 = To Single Precision Float(number=w498) -> (single precision float=w482:sgl)
                            n268 = To Single Precision Float(number=w497) -> (single precision float=w483:sgl)
                            n269 = To Single Precision Float(number=w496) -> (single precision float=w484:sgl)
                            n270 = To Single Precision Float(number=w495) -> (single precision float=w485:sgl)
                            n271 = To Single Precision Float(number=w487) -> (single precision float=w477:sgl)
                            n272 = To Single Precision Float(number=w494) -> (single precision float=w486:sgl)
                            n273 = property class="Clust (严格)"(reference=w505) -> (reference out=w507:refnum<vi>, "Value"=w508:T5)  [unwired: 1 in, 1 out]
                            n274 = Bundle By Name(cluster=w508, "总电压过高"=w502, "总电压过低"=w500, "温度过高"=w498, "温度过低"=w496, "整组温度不均衡"=w487) -> (w506:T5)
                            n275 = Equal?(x=w478, y=w479) -> (x = y?=w493:bool)
                            n276 = Equal?(x=w480, y=w481) -> (x = y?=w492:bool)
                            n277 = Equal?(x=w482, y=w483) -> (x = y?=w491:bool)
                            n278 = Equal?(x=w484, y=w485) -> (x = y?=w490:bool)
                            n279 = Equal?(x=w477, y=w486) -> (x = y?=w489:bool)
                            n280 = Compound Arithmetic op=AND(w493, w492, w491, w490, w489) -> (→"一级故障1":bool)
                            n281 = property class="Clust (严格)"(reference=w507, "Value"=w506) -> ()  [unwired: 1 in, 2 out]
                          }
                          frame 1 {
                            n282 = Join Numbers(hi=w563, lo=w562) -> ((hi.lo)=w548:u16)
                            n283 = Join Numbers(hi=w560, lo=w559) -> ((hi.lo)=w547:u16)
                            n284 = Join Numbers(hi=w558, lo=w557) -> ((hi.lo)=w554:u16)
                            n285 = Join Numbers(hi=w556, lo=w555) -> ((hi.lo)=w553:u16)
                            n286 = global read "读配置文件全局.vi" "一级故障"() -> (w545:sgl[])
                            n287 = call "输出分辨率计算.vi"("分辨率"=0.001, "数值 3"=w553, "数值 2"=w554) -> ("输出3"=w529:dbl, "输出2"=w530:dbl)  [unwired: 3 in, 4 out]
                            n288 = call "输出分辨率计算.vi"("分辨率"=0.001, "数值 3"=w547, "数值 2"=w548) -> ("输出3"=w531:dbl, "输出2"=w532:dbl)  [unwired: 3 in, 4 out]
                            n289 = Index Array(array=w545, index #1=4 ("索引"), index #2=5 ("索引"), index #3=8 ("索引"), index #4=9 ("索引")) -> (element #1=w544:sgl, element #2=w543:sgl, element #3=w542:sgl, element #4=w541:sgl)
                            n290 = property class="Clust (严格)"(reference=w549) -> (reference out=w551:refnum<vi>, "Value"=w552:T5)  [unwired: 1 in, 1 out]
                            n291 = Bundle By Name(cluster=w552, "单组电压不均衡"=w532, "整组电压不均衡"=w531, "单体电压过高"=w530, "单体电压过低"=w529) -> (w550:T5)
                            n292 = To Single Precision Float(number=w530) -> (single precision float=w524:sgl)
                            n293 = To Single Precision Float(number=w529) -> (single precision float=w526:sgl)
                            n294 = To Single Precision Float(number=w542) -> (single precision float=w525:sgl)
                            n295 = To Single Precision Float(number=w541) -> (single precision float=w527:sgl)
                            n296 = To Single Precision Float(number=w543) -> (single precision float=w523:sgl)
                            n297 = To Single Precision Float(number=w531) -> (single precision float=w522:sgl)
                            n298 = To Single Precision Float(number=w532) -> (single precision float=w520:sgl)
                            n299 = To Single Precision Float(number=w544) -> (single precision float=w521:sgl)
                            n300 = property class="Clust (严格)"(reference=w551, "Value"=w550) -> ()  [unwired: 1 in, 2 out]
                            n301 = Equal?(x=w520, y=w521) -> (x = y?=w540:bool)
                            n302 = Equal?(x=w522, y=w523) -> (x = y?=w539:bool)
                            n303 = Equal?(x=w524, y=w525) -> (x = y?=w538:bool)
                            n304 = Equal?(x=w526, y=w527) -> (x = y?=w537:bool)
                            n305 = Compound Arithmetic op=AND(w540, w539, w538, w537) -> (→"一级故障1 2":bool)
                          }
                          frame 2 {
                            n306 = Join Numbers(hi=w610, lo=w609) -> ((hi.lo)=w602:u16)
                            n307 = Join Numbers(hi=w608, lo=w607) -> ((hi.lo)=w601:u16)
                            n308 = global read "读配置文件全局.vi" "一级故障"() -> (w594:sgl[])
                            n309 = Join Numbers(hi=w600, lo=w599) -> ((hi.lo)=w596:u16)
                            n310 = Join Numbers(hi=w598, lo=w597) -> ((hi.lo)=w595:u16)
                            n311 = Index Array(array=w594, index #1=10 ("索引"), index #2=11 ("索引"), index #3=7 ("索引"), index #4=12 ("索引"), index #5=13 ("索引")) -> (element #1=w593:sgl, element #2=w592:sgl, element #3=w591:sgl, element #4=w590:sgl, element #5=w577:sgl)
                            n312 = call "输出分辨率计算.vi"("偏移量"=sgl 0.0, "数值1"=w602, "分辨率"=0.1, "数值 4"=w595, "数值 3"=w596, "数值 2"=w601) -> ("输出4"=w576:dbl, "输出3"=w578:dbl, "输出2"=w579:dbl, "输出1"=w580:dbl)  [unwired: 2 out]
                            n313 = To Single Precision Float(number=w577) -> (single precision float=w572:sgl)
                            n314 = To Single Precision Float(number=w590) -> (single precision float=w570:sgl)
                            n315 = To Single Precision Float(number=w576) -> (single precision float=w571:sgl)
                            n316 = To Single Precision Float(number=w578) -> (single precision float=w569:sgl)
                            n317 = To Single Precision Float(number=w591) -> (single precision float=w568:sgl)
                            n318 = To Single Precision Float(number=w592) -> (single precision float=w567:sgl)
                            n319 = To Single Precision Float(number=w593) -> (single precision float=w565:sgl)
                            n320 = To Single Precision Float(number=w579) -> (single precision float=w566:sgl)
                            n321 = To Single Precision Float(number=w580) -> (single precision float=w564:sgl)
                            n322 = property class="Clust (严格)"(reference=w603) -> (reference out=w605:refnum<vi>, "Value"=w606:T5)  [unwired: 1 in, 1 out]
                            n323 = Bundle By Name(cluster=w606, "充电电流过高"=w580, "放电电流过高"=w579, "单组温度不均衡"=w573, "SOC过高"=w578, "SOC过低"=w576) -> (w604:T5)
                            n324 = Equal?(x=w564, y=w565) -> (x = y?=w589:bool)
                            n325 = Equal?(x=w566, y=w567) -> (x = y?=w588:bool)
                            n326 = Equal?(x=w573, y=w568) -> (x = y?=w587:bool)
                            n327 = Equal?(x=w569, y=w570) -> (x = y?=w586:bool)
                            n328 = Equal?(x=w572, y=w571) -> (x = y?=w575:bool)
                            n329 = property class="Clust (严格)"(reference=w605, "Value"=w604) -> ()  [unwired: 1 in, 2 out]
                            n330 = Compound Arithmetic op=AND(w589, w588, w587, w586, w575) -> (→"一级故障5":bool)
                          }
                          frame 3 {
                            n331 = Join Numbers(hi=w639, lo=w638) -> ((hi.lo)=w637:u16)
                            n332 = global read "读配置文件全局.vi" "一级故障"() -> (w635:sgl[])
                            n333 = local read "一级故障1 2"() -> (w621:bool)
                            n334 = local read "一级故障1"() -> (w622:bool)
                            n335 = local read "一级故障5"() -> (w620:bool)
                            n336 = Index Array(array=w635, index #1=14 ("索引"), index #2=15 ("索引"), index #3=16 ("索引")) -> (element #1=w631:sgl, element #2=w630:sgl, element #3=w629:sgl)
                            n337 = call "输出分辨率计算.vi"("偏移量"=sgl -40.0, "分辨率"=1.0, "数值 3"=w642) -> ("输出3"=w627:dbl)  [unwired: 3 in, 5 out]
                            n338 = call "输出分辨率计算.vi"("数值1"=w636, "分辨率"=0.1, "数值 2"=w637) -> ("输出2"=w626:dbl, "输出1"=w628:dbl)  [unwired: 3 in, 4 out]
                            n339 = To Single Precision Float(number=w626) -> (single precision float=w618:sgl)
                            n340 = To Single Precision Float(number=w629) -> (single precision float=w617:sgl)
                            n341 = To Single Precision Float(number=w627) -> (single precision float=w616:sgl)
                            n342 = To Single Precision Float(number=w630) -> (single precision float=w615:sgl)
                            n343 = To Single Precision Float(number=w628) -> (single precision float=w614:sgl)
                            n344 = To Single Precision Float(number=w631) -> (single precision float=w613:sgl)
                            n345 = property class="Clust (严格)"(reference=w643) -> (reference out=w645:refnum<vi>, "Value"=w646:T5)  [unwired: 1 in, 1 out]
                            n346 = Equal?(x=w613, y=w614) -> (x = y?=w625:bool)
                            n347 = Equal?(x=w615, y=w616) -> (x = y?=w624:bool)
                            n348 = Equal?(x=w617, y=w618) -> (x = y?=w623:bool)
                            n349 = Bundle By Name(cluster=w646, "内阻过大"=w628, "极柱温度过高"=w627, "SOH过低"=w626) -> (w644:T5)
                            n350 = Compound Arithmetic op=AND(w625, w624, w623, w622, w621, w620) -> (w619:bool)
                            n351 = property class="Clust (严格)"(reference=w645, "Value"=w644) -> ()  [unwired: 1 in, 2 out]
                            n352 = global write "读配置文件全局.vi" "一级故障判定"(w619) -> ()
                          }
                        }
                      }
                      n353 = Build Array("一级故障阀值     读取成功" ("字符串")) -> (w417:string[])
                      n354 = call "表格编辑.vi"("新元素/子数组"=w417, "活动单元格:单元格背景色"=u32 6618880, "MCListbox引用句柄"=w414) -> ()  [unwired: 9 out]
                      n355 = global write "EV05全局变量1.vi" "写入超时"(TRUE ("写入超时")) -> ()
                    }
                    frame 2 {
                      n356 = Unbundle By Name(w654) -> ("一级故障 2"=w653:refnum<vi>)
                      n357 = Reshape Array(w658, 28 ("维数大小")) -> (w655:u8[])
                      n358 = for {
                        N: 4 -> [_]
                        tunnel: w655 -> [w680]
                        tunnel: w653 -> [w662]
                        i -> [w677]
                        n359 = case shown="2" w677 {
                          tunnel: [0 7 15 24] -> w676
                          tunnel: [1 8 16 25] -> w675
                          tunnel: [2 9 17 26] -> w674
                          tunnel: [3 10 18 27] -> w673
                          tunnel: [4 11 19 _] -> w672
                          tunnel: [5 12 20 _] -> w671
                          tunnel: [6 13 21 _] -> w670
                          tunnel: [0 14 22 _] -> w669
                          tunnel: [_ _ 23 _] -> w661
                          frame 0, Default {
                          }
                          frame 1 {
                          }
                          frame 2 {
                          }
                          frame 3 {
                          }
                        }
                        n360 = global write "EV05全局变量1.vi" "写入超时"(TRUE ("写入超时")) -> ()
                        n361 = Index Array(array=w680, index #1=w676, index #2=w675, index #3=w674, index #4=w673, index #5=w672, index #6=w671, index #7=w670, index #8=w669, index #9=w661) -> (element #1=w679:u8, element #2=w678:u8, element #3=w668:u8, element #4=w667:u8, element #5=w666:u8, element #6=w665:u8, element #7=w664:u8, element #8=w663:u8, element #9=w660:u8)
                        n362 = case shown="2" w677 {
                          tunnel: w679 -> [w751 w795 w842 w868]
                          tunnel: w678 -> [w748 w794 w841 w874]
                          tunnel: w668 -> [w747 w792 w840 w870]
                          tunnel: w667 -> [w746 w791 w839 w871]
                          tunnel: w666 -> [w742 w790 w805 _]
                          tunnel: w665 -> [w741 w789 w832 _]
                          tunnel: w664 -> [w720 w788 w831 _]
                          tunnel: w663 -> [_ w787 w830 _]
                          tunnel: w662 -> [w737 w781 w835 w875]
                          tunnel: w660 -> [_ _ w829 _]
                          frame 0, Default {
                            n363 = global read "读配置文件全局.vi" "二级故障"() -> (w736:sgl[])
                            n364 = Join Numbers(hi=w751, lo=w748) -> ((hi.lo)=w750:u16)
                            n365 = Join Numbers(hi=w747, lo=w746) -> ((hi.lo)=w745:u16)
                            n366 = call "输出分辨率计算.vi"("偏移量"=sgl -40.0, "分辨率"=1.0, "数值 3"=w741, "数值 2"=w742) -> ("输出3"=w721:dbl, "输出2"=w722:dbl)  [unwired: 2 in, 4 out]
                            n367 = call "输出分辨率计算.vi"("分辨率"=0.1, "数值 3"=w745, "数值 2"=w750) -> ("输出3"=w723:dbl, "输出2"=w724:dbl)  [unwired: 3 in, 4 out]
                            n368 = Index Array(array=w736, index #5=6 ("索引")) -> (element #1=w734:sgl, element #2=w733:sgl, element #3=w732:sgl, element #4=w731:sgl, element #5=w711:sgl)  [unwired: 4 in]
                            n369 = To Single Precision Float(number=w720) -> (single precision float=w710:sgl)
                            n370 = To Single Precision Float(number=w731) -> (single precision float=w719:sgl)
                            n371 = To Single Precision Float(number=w732) -> (single precision float=w717:sgl)
                            n372 = To Single Precision Float(number=w722) -> (single precision float=w716:sgl)
                            n373 = To Single Precision Float(number=w734) -> (single precision float=w713:sgl)
                            n374 = To Single Precision Float(number=w721) -> (single precision float=w718:sgl)
                            n375 = To Single Precision Float(number=w723) -> (single precision float=w714:sgl)
                            n376 = To Single Precision Float(number=w733) -> (single precision float=w715:sgl)
                            n377 = To Single Precision Float(number=w724) -> (single precision float=w712:sgl)
                            n378 = property class="Clust (严格)"(reference=w737) -> (reference out=w739:refnum<vi>, "Value"=w740:T5)  [unwired: 1 in, 1 out]
                            n379 = Bundle By Name(cluster=w740, "总电压过高"=w724, "总电压过低"=w723, "温度过高"=w722, "温度过低"=w721, "整组温度不均衡"=w720) -> (w738:T5)
                            n380 = Equal?(x=w712, y=w713) -> (x = y?=w730:bool)
                            n381 = Equal?(x=w714, y=w715) -> (x = y?=w729:bool)
                            n382 = Equal?(x=w716, y=w717) -> (x = y?=w728:bool)
                            n383 = Equal?(x=w718, y=w719) -> (x = y?=w727:bool)
                            n384 = Equal?(x=w710, y=w711) -> (x = y?=w726:bool)
                            n385 = property class="Clust (严格)"(reference=w739, "Value"=w738) -> ()  [unwired: 1 in, 2 out]
                            n386 = Compound Arithmetic op=AND(w730, w729, w728, w727, w726) -> (→"一级故障1 3":bool)
                          }
                          frame 1 {
                            n387 = global read "读配置文件全局.vi" "二级故障"() -> (w777:sgl[])
                            n388 = Join Numbers(hi=w795, lo=w794) -> ((hi.lo)=w780:u16)
                            n389 = Join Numbers(hi=w792, lo=w791) -> ((hi.lo)=w779:u16)
                            n390 = Join Numbers(hi=w790, lo=w789) -> ((hi.lo)=w786:u16)
                            n391 = Join Numbers(hi=w788, lo=w787) -> ((hi.lo)=w785:u16)
                            n392 = call "输出分辨率计算.vi"("分辨率"=0.001, "数值 3"=w785, "数值 2"=w786) -> ("输出3"=w762:dbl, "输出2"=w765:dbl)  [unwired: 3 in, 4 out]
                            n393 = call "输出分辨率计算.vi"("分辨率"=0.001, "数值 3"=w779, "数值 2"=w780) -> ("输出3"=w766:dbl, "输出2"=w767:dbl)  [unwired: 3 in, 4 out]
                            n394 = Index Array(array=w777, index #1=4 ("索引"), index #2=5 ("索引"), index #3=8 ("索引"), index #4=9 ("索引")) -> (element #1=w776:sgl, element #2=w775:sgl, element #3=w758:sgl, element #4=w761:sgl)
                            n395 = To Single Precision Float(number=w776) -> (single precision float=w754:sgl)
                            n396 = To Single Precision Float(number=w775) -> (single precision float=w755:sgl)
                            n397 = To Single Precision Float(number=w761) -> (single precision float=w759:sgl)
                            n398 = To Single Precision Float(number=w762) -> (single precision float=w760:sgl)
                            n399 = To Single Precision Float(number=w758) -> (single precision float=w756:sgl)
                            n400 = To Single Precision Float(number=w765) -> (single precision float=w757:sgl)
                            n401 = To Single Precision Float(number=w766) -> (single precision float=w753:sgl)
                            n402 = To Single Precision Float(number=w767) -> (single precision float=w752:sgl)
                            n403 = property class="Clust (严格)"(reference=w781) -> (reference out=w783:refnum<vi>, "Value"=w784:T5)  [unwired: 1 in, 1 out]
                            n404 = Bundle By Name(cluster=w784, "单组电压不均衡"=w767, "整组电压不均衡"=w766, "单体电压过高"=w765, "单体电压过低"=w762) -> (w782:T5)
                            n405 = Equal?(x=w752, y=w754) -> (x = y?=w774:bool)
                            n406 = Equal?(x=w753, y=w755) -> (x = y?=w773:bool)
                            n407 = Equal?(x=w757, y=w756) -> (x = y?=w764:bool)
                            n408 = Equal?(x=w760, y=w759) -> (x = y?=w763:bool)
                            n409 = property class="Clust (严格)"(reference=w783, "Value"=w782) -> ()  [unwired: 1 in, 2 out]
                            n410 = Compound Arithmetic op=AND(w774, w773, w764, w763) -> (→"一级故障1 4":bool)
                          }
                          frame 2 {
                            n411 = global read "读配置文件全局.vi" "二级故障"() -> (w826:sgl[])
                            n412 = Join Numbers(hi=w842, lo=w841) -> ((hi.lo)=w834:u16)
                            n413 = Join Numbers(hi=w840, lo=w839) -> ((hi.lo)=w833:u16)
                            n414 = Join Numbers(hi=w832, lo=w831) -> ((hi.lo)=w827:u16)
                            n415 = Join Numbers(hi=w830, lo=w829) -> ((hi.lo)=w828:u16)
                            n416 = Index Array(array=w826, index #1=10 ("索引"), index #2=11 ("索引"), index #3=7 ("索引"), index #4=12 ("索引"), index #5=13 ("索引")) -> (element #1=w825:sgl, element #2=w824:sgl, element #3=w823:sgl, element #4=w822:sgl, element #5=w812:sgl)
                            n417 = call "输出分辨率计算.vi"("偏移量"=sgl 0.0, "数值1"=w834, "分辨率"=0.1, "数值 4"=w828, "数值 3"=w827, "数值 2"=w833) -> ("输出4"=w808:dbl, "输出3"=w809:dbl, "输出2"=w810:dbl, "输出1"=w811:dbl)  [unwired: 2 out]
                            n418 = To Single Precision Float(number=w808) -> (single precision float=w804:sgl)
                            n419 = To Single Precision Float(number=w812) -> (single precision float=w803:sgl)
                            n420 = To Single Precision Float(number=w811) -> (single precision float=w796:sgl)
                            n421 = To Single Precision Float(number=w809) -> (single precision float=w801:sgl)
                            n422 = To Single Precision Float(number=w822) -> (single precision float=w802:sgl)
                            n423 = To Single Precision Float(number=w825) -> (single precision float=w797:sgl)
                            n424 = To Single Precision Float(number=w810) -> (single precision float=w798:sgl)
                            n425 = To Single Precision Float(number=w824) -> (single precision float=w799:sgl)
                            n426 = To Single Precision Float(number=w823) -> (single precision float=w800:sgl)
                            n427 = property class="Clust (严格)"(reference=w835) -> (reference out=w837:refnum<vi>, "Value"=w838:T5)  [unwired: 1 in, 1 out]
                            n428 = Bundle By Name(cluster=w838, "充电电流过高"=w811, "放电电流过高"=w810, "单组温度不均衡"=w805, "SOC过高"=w809, "SOC过低"=w808) -> (w836:T5)
                            n429 = Equal?(x=w796, y=w797) -> (x = y?=w821:bool)
                            n430 = Equal?(x=w798, y=w799) -> (x = y?=w820:bool)
                            n431 = Equal?(x=w805, y=w800) -> (x = y?=w819:bool)
                            n432 = Equal?(x=w801, y=w802) -> (x = y?=w818:bool)
                            n433 = Equal?(x=w803, y=w804) -> (x = y?=w807:bool)
                            n434 = property class="Clust (严格)"(reference=w837, "Value"=w836) -> ()  [unwired: 1 in, 2 out]
                            n435 = Compound Arithmetic op=AND(w821, w820, w819, w818, w807) -> (→"二级故障1":bool)
                          }
                          frame 3 {
                            n436 = Join Numbers(hi=w870, lo=w871) -> ((hi.lo)=w869:u16)
                            n437 = global read "读配置文件全局.vi" "二级故障"() -> (w867:sgl[])
                            n438 = local read "一级故障1 3"() -> (w854:bool)
                            n439 = local read "一级故障1 4"() -> (w853:bool)
                            n440 = local read "二级故障1"() -> (w852:bool)
                            n441 = call "输出分辨率计算.vi"("数值1"=w868, "分辨率"=0.1, "数值 2"=w869) -> ("输出2"=w855:dbl, "输出1"=w857:dbl)  [unwired: 3 in, 4 out]
                            n442 = Index Array(array=w867, index #1=14 ("索引"), index #2=15 ("索引"), index #3=16 ("索引")) -> (element #1=w863:sgl, element #2=w862:sgl, element #3=w861:sgl)
                            n443 = call "输出分辨率计算.vi"("偏移量"=sgl -40.0, "分辨率"=1.0, "数值 3"=w874) -> ("输出3"=w856:dbl)  [unwired: 3 in, 5 out]
                            n444 = To Single Precision Float(number=w861) -> (single precision float=w849:sgl)
                            n445 = To Single Precision Float(number=w856) -> (single precision float=w848:sgl)
                            n446 = To Single Precision Float(number=w862) -> (single precision float=w847:sgl)
                            n447 = To Single Precision Float(number=w855) -> (single precision float=w850:sgl)
                            n448 = To Single Precision Float(number=w863) -> (single precision float=w845:sgl)
                            n449 = To Single Precision Float(number=w857) -> (single precision float=w846:sgl)
                            n450 = Equal?(x=w845, y=w846) -> (x = y?=w860:bool)
                            n451 = Equal?(x=w847, y=w848) -> (x = y?=w859:bool)
                            n452 = Equal?(x=w849, y=w850) -> (x = y?=w858:bool)
                            n453 = property class="Clust (严格)"(reference=w875) -> (reference out=w877:refnum<vi>, "Value"=w878:T5)  [unwired: 1 in, 1 out]
                            n454 = Bundle By Name(cluster=w878, "内阻过大"=w857, "极柱温度过高"=w856, "SOH过低"=w855) -> (w876:T5)
                            n455 = Compound Arithmetic op=AND(w860, w859, w858, w854, w853, w852) -> (w851:bool)
                            n456 = property class="Clust (严格)"(reference=w877, "Value"=w876) -> ()  [unwired: 1 in, 2 out]
                            n457 = global write "读配置文件全局.vi" "二级故障判定"(w851) -> ()
                          }
                        }
                      }
                      n458 = Build Array("二级故障阀值     读取成功" ("字符串")) -> (w652:string[])
                      n459 = call "表格编辑.vi"("新元素/子数组"=w652, "活动单元格:单元格背景色"=u32 6618880, "MCListbox引用句柄"=w650) -> ()  [unwired: 9 out]
                      n460 = global write "EV05全局变量1.vi" "写入超时"(TRUE ("写入超时")) -> ()
                    }
                    frame 3 {
                      n461 = Unbundle By Name(w886) -> ("一级故障 3"=w885:refnum<vi>)
                      n462 = Reshape Array(w890, 28 ("维数大小")) -> (w887:u8[])
                      n463 = for {
                        N: 4 -> [_]
                        tunnel: w887 -> [w911]
                        tunnel: w885 -> [w893]
                        i -> [w908]
                        n464 = case shown="0, 默认" w908 {
                          tunnel: [0 7 15 24] -> w907
                          tunnel: [1 8 16 25] -> w906
                          tunnel: [2 9 17 26] -> w905
                          tunnel: [3 10 18 27] -> w904
                          tunnel: [4 11 19 _] -> w903
                          tunnel: [5 12 20 _] -> w902
                          tunnel: [6 13 21 _] -> w901
                          tunnel: [0 14 22 _] -> w900
                          tunnel: [_ _ 23 _] -> w892
                          frame 0, Default {
                          }
                          frame 1 {
                          }
                          frame 2 {
                          }
                          frame 3 {
                          }
                        }
                        n465 = Index Array(array=w911, index #1=w907, index #2=w906, index #3=w905, index #4=w904, index #5=w903, index #6=w902, index #7=w901, index #8=w900, index #9=w892) -> (element #1=w910:u8, element #2=w909:u8, element #3=w899:u8, element #4=w898:u8, element #5=w897:u8, element #6=w896:u8, element #7=w895:u8, element #8=w894:u8, element #9=w891:u8)
                        n466 = case shown="0, 默认" w908 {
                          tunnel: w910 -> [w983 w1027 w1074 w1100]
                          tunnel: w909 -> [w980 w1026 w1073 w1106]
                          tunnel: w899 -> [w979 w1024 w1072 w1103]
                          tunnel: w898 -> [w978 w1023 w1071 w1102]
                          tunnel: w897 -> [w974 w1022 w1037 _]
                          tunnel: w896 -> [w973 w1021 w1062 _]
                          tunnel: w895 -> [w951 w1020 w1061 _]
                          tunnel: w894 -> [_ w1019 w1064 _]
                          tunnel: w893 -> [w969 w1013 w1067 w1107]
                          tunnel: w891 -> [_ _ w1063 _]
                          frame 0, Default {
                            n467 = global read "读配置文件全局.vi" "三级故障"() -> (w968:sgl[])
                            n468 = Join Numbers(hi=w983, lo=w980) -> ((hi.lo)=w982:u16)
                            n469 = Join Numbers(hi=w979, lo=w978) -> ((hi.lo)=w977:u16)
                            n470 = call "输出分辨率计算.vi"("偏移量"=sgl -40.0, "分辨率"=1.0, "数值 3"=w973, "数值 2"=w974) -> ("输出3"=w953:dbl, "输出2"=w954:dbl)  [unwired: 2 in, 4 out]
                            n471 = call "输出分辨率计算.vi"("分辨率"=0.1, "数值 3"=w977, "数值 2"=w982) -> ("输出3"=w955:dbl, "输出2"=w956:dbl)  [unwired: 3 in, 4 out]
                            n472 = Index Array(array=w968, index #5=6 ("索引")) -> (element #1=w966:sgl, element #2=w965:sgl, element #3=w964:sgl, element #4=w963:sgl, element #5=w952:sgl)  [unwired: 4 in]
                            n473 = To Single Precision Float(number=w953) -> (single precision float=w948:sgl)
                            n474 = To Single Precision Float(number=w963) -> (single precision float=w949:sgl)
                            n475 = To Single Precision Float(number=w956) -> (single precision float=w942:sgl)
                            n476 = To Single Precision Float(number=w964) -> (single precision float=w947:sgl)
                            n477 = To Single Precision Float(number=w951) -> (single precision float=w941:sgl)
                            n478 = To Single Precision Float(number=w965) -> (single precision float=w945:sgl)
                            n479 = To Single Precision Float(number=w954) -> (single precision float=w946:sgl)
                            n480 = To Single Precision Float(number=w952) -> (single precision float=w950:sgl)
                            n481 = To Single Precision Float(number=w966) -> (single precision float=w943:sgl)
                            n482 = To Single Precision Float(number=w955) -> (single precision float=w944:sgl)
                            n483 = property class="Clust (严格)"(reference=w969) -> (reference out=w971:refnum<vi>, "Value"=w972:T5)  [unwired: 1 in, 1 out]
                            n484 = Bundle By Name(cluster=w972, "总电压过高"=w956, "总电压过低"=w955, "温度过高"=w954, "温度过低"=w953, "整组温度不均衡"=w951) -> (w970:T5)
                            n485 = Equal?(x=w942, y=w943) -> (x = y?=w962:bool)
                            n486 = Equal?(x=w944, y=w945) -> (x = y?=w961:bool)
                            n487 = Equal?(x=w946, y=w947) -> (x = y?=w960:bool)
                            n488 = Equal?(x=w948, y=w949) -> (x = y?=w959:bool)
                            n489 = Equal?(x=w941, y=w950) -> (x = y?=w958:bool)
                            n490 = property class="Clust (严格)"(reference=w971, "Value"=w970) -> ()  [unwired: 1 in, 2 out]
                            n491 = Compound Arithmetic op=AND(w962, w961, w960, w959, w958) -> (→"一级故障1 5":bool)
                          }
                          frame 1 {
                            n492 = global read "读配置文件全局.vi" "三级故障"() -> (w1009:sgl[])
                            n493 = Join Numbers(hi=w1027, lo=w1026) -> ((hi.lo)=w1012:u16)
                            n494 = Join Numbers(hi=w1024, lo=w1023) -> ((hi.lo)=w1011:u16)
                            n495 = Join Numbers(hi=w1022, lo=w1021) -> ((hi.lo)=w1018:u16)
                            n496 = Join Numbers(hi=w1020, lo=w1019) -> ((hi.lo)=w1017:u16)
                            n497 = call "输出分辨率计算.vi"("分辨率"=0.001, "数值 3"=w1017, "数值 2"=w1018) -> ("输出3"=w992:dbl, "输出2"=w993:dbl)  [unwired: 3 in, 4 out]
                            n498 = call "输出分辨率计算.vi"("分辨率"=0.001, "数值 3"=w1011, "数值 2"=w1012) -> ("输出3"=w994:dbl, "输出2"=w995:dbl)  [unwired: 3 in, 4 out]
                            n499 = Index Array(array=w1009, index #1=4 ("索引"), index #2=5 ("索引"), index #3=8 ("索引"), index #4=9 ("索引")) -> (element #1=w1008:sgl, element #2=w1007:sgl, element #3=w1006:sgl, element #4=w1005:sgl)
                            n500 = To Single Precision Float(number=w1006) -> (single precision float=w986:sgl)
                            n501 = To Single Precision Float(number=w993) -> (single precision float=w987:sgl)
                            n502 = To Single Precision Float(number=w1005) -> (single precision float=w984:sgl)
                            n503 = property class="Clust (严格)"(reference=w1013) -> (reference out=w1015:refnum<vi>, "Value"=w1016:T5)  [unwired: 1 in, 1 out]
                            n504 = Bundle By Name(cluster=w1016, "单组电压不均衡"=w995, "整组电压不均衡"=w994, "单体电压过高"=w993, "单体电压过低"=w992) -> (w1014:T5)
                            n505 = To Single Precision Float(number=w992) -> (single precision float=w985:sgl)
                            n506 = To Single Precision Float(number=w1007) -> (single precision float=w988:sgl)
                            n507 = To Single Precision Float(number=w995) -> (single precision float=w991:sgl)
                            n508 = To Single Precision Float(number=w1008) -> (single precision float=w990:sgl)
                            n509 = To Single Precision Float(number=w994) -> (single precision float=w989:sgl)
                            n510 = Equal?(x=w991, y=w990) -> (x = y?=w1004:bool)
                            n511 = Equal?(x=w989, y=w988) -> (x = y?=w1003:bool)
                            n512 = Equal?(x=w987, y=w986) -> (x = y?=w1002:bool)
                            n513 = Equal?(x=w985, y=w984) -> (x = y?=w1001:bool)
                            n514 = property class="Clust (严格)"(reference=w1015, "Value"=w1014) -> ()  [unwired: 1 in, 2 out]
                            n515 = Compound Arithmetic op=AND(w1004, w1003, w1002, w1001) -> (→"一级故障1 6":bool)
                          }
                          frame 2 {
                            n516 = Join Numbers(hi=w1074, lo=w1073) -> ((hi.lo)=w1066:u16)
                            n517 = Join Numbers(hi=w1072, lo=w1071) -> ((hi.lo)=w1065:u16)
                            n518 = Join Numbers(hi=w1062, lo=w1061) -> ((hi.lo)=w1060:u16)
                            n519 = Join Numbers(hi=w1064, lo=w1063) -> ((hi.lo)=w1059:u16)
                            n520 = global read "读配置文件全局.vi" "三级故障"() -> (w1058:sgl[])
                            n521 = Index Array(array=w1058, index #1=10 ("索引"), index #2=11 ("索引"), index #3=7 ("索引"), index #4=12 ("索引"), index #5=13 ("索引")) -> (element #1=w1057:sgl, element #2=w1056:sgl, element #3=w1055:sgl, element #4=w1054:sgl, element #5=w1044:sgl)
                            n522 = call "输出分辨率计算.vi"("偏移量"=sgl 0.0, "数值1"=w1066, "分辨率"=0.1, "数值 4"=w1059, "数值 3"=w1060, "数值 2"=w1065) -> ("输出4"=w1038:dbl, "输出3"=w1039:dbl, "输出2"=w1040:dbl, "输出1"=w1041:dbl)  [unwired: 2 out]
                            n523 = To Single Precision Float(number=w1054) -> (single precision float=w1034:sgl)
                            n524 = To Single Precision Float(number=w1044) -> (single precision float=w1036:sgl)
                            n525 = To Single Precision Float(number=w1055) -> (single precision float=w1032:sgl)
                            n526 = To Single Precision Float(number=w1056) -> (single precision float=w1031:sgl)
                            n527 = To Single Precision Float(number=w1039) -> (single precision float=w1033:sgl)
                            n528 = To Single Precision Float(number=w1038) -> (single precision float=w1035:sgl)
                            n529 = To Single Precision Float(number=w1040) -> (single precision float=w1030:sgl)
                            n530 = To Single Precision Float(number=w1057) -> (single precision float=w1029:sgl)
                            n531 = To Single Precision Float(number=w1041) -> (single precision float=w1028:sgl)
                            n532 = Equal?(x=w1028, y=w1029) -> (x = y?=w1053:bool)
                            n533 = Equal?(x=w1030, y=w1031) -> (x = y?=w1052:bool)
                            n534 = Equal?(x=w1037, y=w1032) -> (x = y?=w1051:bool)
                            n535 = Equal?(x=w1033, y=w1034) -> (x = y?=w1050:bool)
                            n536 = Equal?(x=w1036, y=w1035) -> (x = y?=w1043:bool)
                            n537 = property class="Clust (严格)"(reference=w1067) -> (reference out=w1069:refnum<vi>, "Value"=w1070:T5)  [unwired: 1 in, 1 out]
                            n538 = Bundle By Name(cluster=w1070, "充电电流过高"=w1041, "放电电流过高"=w1040, "单组温度不均衡"=w1037, "SOC过高"=w1039, "SOC过低"=w1038) -> (w1068:T5)
                            n539 = Compound Arithmetic op=AND(w1053, w1052, w1051, w1050, w1043) -> (→"二级故障1 2":bool)
                            n540 = property class="Clust (严格)"(reference=w1069, "Value"=w1068) -> ()  [unwired: 1 in, 2 out]
                          }
                          frame 3 {
                            n541 = global read "读配置文件全局.vi" "三级故障"() -> (w1099:sgl[])
                            n542 = local read "二级故障1 2"() -> (w1083:bool)
                            n543 = local read "一级故障1 5"() -> (w1085:bool)
                            n544 = local read "一级故障1 6"() -> (w1084:bool)
                            n545 = Join Numbers(hi=w1103, lo=w1102) -> ((hi.lo)=w1101:u16)
                            n546 = Index Array(array=w1099, index #1=14 ("索引"), index #2=15 ("索引"), index #3=16 ("索引")) -> (element #1=w1095:sgl, element #2=w1094:sgl, element #3=w1088:sgl)
                            n547 = call "输出分辨率计算.vi"("偏移量"=sgl -40.0, "分辨率"=1.0, "数值 3"=w1106) -> ("输出3"=w1089:dbl)  [unwired: 3 in, 5 out]
                            n548 = call "输出分辨率计算.vi"("数值1"=w1100, "分辨率"=0.1, "数值 2"=w1101) -> ("输出2"=w1087:dbl, "输出1"=w1090:dbl)  [unwired: 3 in, 4 out]
                            n549 = To Single Precision Float(number=w1094) -> (single precision float=w1080:sgl)
                            n550 = To Single Precision Float(number=w1089) -> (single precision float=w1079:sgl)
                            n551 = To Single Precision Float(number=w1088) -> (single precision float=w1078:sgl)
                            n552 = To Single Precision Float(number=w1087) -> (single precision float=w1077:sgl)
                            n553 = To Single Precision Float(number=w1090) -> (single precision float=w1081:sgl)
                            n554 = To Single Precision Float(number=w1095) -> (single precision float=w1082:sgl)
                            n555 = Equal?(x=w1082, y=w1081) -> (x = y?=w1093:bool)
                            n556 = Equal?(x=w1080, y=w1079) -> (x = y?=w1092:bool)
                            n557 = Equal?(x=w1078, y=w1077) -> (x = y?=w1091:bool)
                            n558 = property class="Clust (严格)"(reference=w1107) -> (reference out=w1109:refnum<vi>, "Value"=w1110:T5)  [unwired: 1 in, 1 out]
                            n559 = Bundle By Name(cluster=w1110, "内阻过大"=w1090, "极柱温度过高"=w1089, "SOH过低"=w1087) -> (w1108:T5)
                            n560 = Compound Arithmetic op=AND(w1093, w1092, w1091, w1085, w1084, w1083) -> (w1086:bool)
                            n561 = property class="Clust (严格)"(reference=w1109, "Value"=w1108) -> ()  [unwired: 1 in, 2 out]
                            n562 = global write "读配置文件全局.vi" "三级故障判定"(w1086) -> ()
                          }
                        }
                      }
                      n563 = Build Array("三级故障阀值     读取成功" ("字符串")) -> (w881:string[])
                      n564 = call "表格编辑.vi"("新元素/子数组"=w881, "活动单元格:单元格背景色"=u32 6618880, "MCListbox引用句柄"=w880) -> ()  [unwired: 9 out]
                      n565 = global write "EV05全局变量1.vi" "写入超时"(TRUE ("写入超时")) -> ()
                    }
                  }
                }
                frame 130 {
                  n566 = case shown="1" w1115 {
                    tunnel: w1114 -> [_ w1157 w1168]
                    tunnel: w1113 -> [_ w1152 w1164]
                    tunnel: w1112 -> [_ w1142 w1160]
                    frame 0, Default {
                    }
                    frame 1 {
                      n567 = Unbundle By Name(w1152) -> ("加热控制参数"=w1151:refnum<vi>)
                      n568 = global read "读配置文件全局.vi" "加热控制参数"() -> (w1140:dbl[])
                      n569 = Reshape Array(w1157, 7 ("维数大小")) -> (w1148:u8[])
                      n570 = Index Array(array=w1148) -> (element #1=w1147:u8, element #2=w1146:u8, element #3=w1120:u8, element #4=w1119:u8, element #5=w1122:u8, element #6=w1121:u8, element #7=w1116:u8)  [unwired: 7 in]
                      n571 = Index Array(array=w1140) -> (element #1=w1139:dbl, element #2=w1138:dbl, element #3=w1137:dbl, element #4=w1136:dbl, element #5=w1130:dbl, element #6=w1135:dbl, element #7=w1118:dbl)  [unwired: 7 in]
                      n572 = call "输出分辨率计算.vi"("偏移量"=sgl -40.0, "数值1"=w1147, "分辨率"=1.0, "数值 4"=w1121, "数值 3"=w1122, "数值 2"=w1146) -> ("输出4"=w1131:dbl, "输出3"=w1132:dbl, "输出2"=w1133:dbl, "输出1"=w1134:dbl)  [unwired: 2 out]
                      n573 = Equal?(x=w1116, y=w1118) -> (x = y?=w1117:bool)
                      n574 = Equal?(x=w1139, y=w1134) -> (x = y?=w1129:bool)
                      n575 = Equal?(x=w1138, y=w1133) -> (x = y?=w1128:bool)
                      n576 = Equal?(x=w1137, y=w1132) -> (x = y?=w1127:bool)
                      n577 = Equal?(x=w1136, y=w1131) -> (x = y?=w1126:bool)
                      n578 = Equal?(x=w1130, y=w1120) -> (x = y?=w1125:bool)
                      n579 = Equal?(x=w1135, y=w1119) -> (x = y?=w1124:bool)
                      n580 = Build Array("加热控制参数     读取成功" ("字符串")) -> (w1145:string[])
                      n581 = Compound Arithmetic op=AND(w1129, w1128, w1127, w1126, w1125, w1124, w1117) -> (w1123:bool)
                      n582 = global write "读配置文件全局.vi" "加热控制参数判定"(w1123) -> ()
                      n583 = call "表格编辑.vi"("新元素/子数组"=w1145, "活动单元格:单元格背景色"=u32 6618880, "MCListbox引用句柄"=w1142) -> ()  [unwired: 9 out]
                      n584 = property class="Clust (严格)"(reference=w1151) -> (reference out=w1154:refnum<vi>, "Value"=w1155:T6)  [unwired: 1 in, 1 out]
                      n585 = Bundle By Name(cluster=w1155, "风机开启温度"=w1134, "风机关闭温度"=w1133, "加热开启温度"=w1132, "加热关闭温度"=w1131, "风机开启温差"=w1120, "风机关闭温差"=w1119, "加热关闭温差"=w1116) -> (w1153:T6)
                      n586 = global write "EV05全局变量1.vi" "写入超时"(TRUE ("写入超时")) -> ()
                      n587 = property class="Clust (严格)"(reference=w1154, "Value"=w1153) -> ()  [unwired: 1 in, 2 out]
                    }
                    frame 2 {
                      n588 = Unbundle By Name(w1164) -> ("充电控制参数"=w1163:refnum<vi>)
                      n589 = Reshape Array(w1168, 14 ("维数大小")) -> (w1165:u8[])
                      n590 = for {
                        N: 2 -> [_]
                        tunnel: w1165 -> [w1185]
                        tunnel: w1163 -> [w1169]
                        i -> [w1177]
                        n591 = case shown="0, 默认" w1177 {
                          tunnel: [0 7 14] -> w1184
                          tunnel: [1 8 15] -> w1183
                          tunnel: [2 9 16] -> w1182
                          tunnel: [3 10 10] -> w1181
                          tunnel: [4 11 11] -> w1180
                          tunnel: [5 12 12] -> w1179
                          tunnel: [6 13 13] -> w1178
                          frame 0, Default {
                          }
                          frame 1 {
                          }
                          frame 2 {
                          }
                        }
                        n592 = Index Array(array=w1185, index #1=w1184, index #2=w1183, index #3=w1182, index #4=w1181, index #5=w1180, index #6=w1179, index #7=w1178) -> (element #1=w1175:u8, element #2=w1176:u8, element #3=w1174:u8, element #4=w1173:u8, element #5=w1172:u8, element #6=w1171:u8, element #7=w1170:u8)
                        n593 = case shown="1" w1177 {
                          tunnel: w1176 -> [w1229 w1275]
                          tunnel: w1175 -> [w1228 w1274]
                          tunnel: w1174 -> [w1227 w1273]
                          tunnel: w1173 -> [w1226 w1272]
                          tunnel: w1172 -> [w1225 w1271]
                          tunnel: w1171 -> [w1224 w1270]
                          tunnel: w1170 -> [w1216 w1264]
                          tunnel: w1169 -> [w1210 w1258]
                          frame 0, Default {
                            n594 = Join Numbers(hi=w1225, lo=w1224) -> ((hi.lo)=w1221:u16)
                            n595 = Join Numbers(hi=w1228, lo=w1229) -> ((hi.lo)=w1223:u16)
                            n596 = Join Numbers(hi=w1227, lo=w1226) -> ((hi.lo)=w1222:u16)
                            n597 = global read "读配置文件全局.vi" "充电控制参数"() -> (w1209:dbl[])
                            n598 = call "输出分辨率计算.vi"("分辨率"=0.1, "数值 2"=w1222) -> ("输出2"=w1201:dbl)  [unwired: 4 in, 5 out]
                            n599 = call "输出分辨率计算.vi"("偏移量"=sgl 0.0, "分辨率"=0.1, "数值 2"=w1221) -> ("输出2"=w1200:dbl)  [unwired: 3 in, 5 out]
                            n600 = call "输出分辨率计算.vi"("分辨率"=0.001, "数值 2"=w1223) -> ("输出2"=w1202:dbl)  [unwired: 4 in, 5 out]
                            n601 = call "输出分辨率计算.vi"("偏移量"=sgl -40.0, "分辨率"=1.0, "数值 2"=w1216) -> ("输出2"=w1199:dbl)  [unwired: 3 in, 5 out]
                            n602 = Index Array(array=w1209, index #3=3 ("索引"), index #4=6 ("索引")) -> (element #1=w1206:dbl, element #2=w1205:dbl, element #3=w1204:dbl, element #4=w1203:dbl)  [unwired: 2 in]
                            n603 = To Single Precision Float(number=w1202) -> (single precision float=w1192:sgl)
                            n604 = To Single Precision Float(number=w1206) -> (single precision float=w1193:sgl)
                            n605 = To Single Precision Float(number=w1203) -> (single precision float=w1187:sgl)
                            n606 = To Single Precision Float(number=w1199) -> (single precision float=w1186:sgl)
                            n607 = To Single Precision Float(number=w1201) -> (single precision float=w1190:sgl)
                            n608 = To Single Precision Float(number=w1200) -> (single precision float=w1188:sgl)
                            n609 = To Single Precision Float(number=w1204) -> (single precision float=w1189:sgl)
                            n610 = To Single Precision Float(number=w1205) -> (single precision float=w1191:sgl)
                            n611 = property class="Clust (严格)"(reference=w1210) -> (reference out=w1212:refnum<vi>, "Value"=w1213:T7)  [unwired: 1 in, 1 out]
                            n612 = Bundle By Name(cluster=w1213, "最大允许单体电压"=w1202, "最大允许总电压"=w1201, "最大允许充电电流"=w1200, "最小允许充电温度"=w1199) -> (w1211:T7)
                            n613 = Equal?(x=w1193, y=w1192) -> (x = y?=w1198:bool)
                            n614 = Equal?(x=w1191, y=w1190) -> (x = y?=w1197:bool)
                            n615 = Equal?(x=w1189, y=w1188) -> (x = y?=w1196:bool)
                            n616 = Equal?(x=w1187, y=w1186) -> (x = y?=w1195:bool)
                            n617 = Compound Arithmetic op=AND(w1198, w1197, w1196, w1195) -> (→"充电控制参数":bool)
                            n618 = property class="Clust (严格)"(reference=w1212, "Value"=w1211) -> ()  [unwired: 1 in, 2 out]
                          }
                          frame 1 {
                            n619 = Join Numbers(hi=w1271, lo=w1270) -> ((hi.lo)=w1268:u16)
                            n620 = Join Numbers(hi=w1274, lo=w1275) -> ((hi.lo)=w1269:u16)
                            n621 = Join Numbers(hi=w1273, lo=w1272) -> ((hi.lo)=w1237:u16)
                            n622 = global read "读配置文件全局.vi" "充电控制参数"() -> (w1257:dbl[])
                            n623 = call "输出分辨率计算.vi"("偏移量"=sgl 0.0, "分辨率"=0.1, "数值 3"=w1237, "数值 2"=w1269) -> ("输出3"=w1236:dbl, "输出2"=w1249:dbl)  [unwired: 2 in, 4 out]
                            n624 = call "输出分辨率计算.vi"("分辨率"=0.001, "数值 2"=w1268) -> ("输出2"=w1242:dbl)  [unwired: 4 in, 5 out]
                            n625 = call "输出分辨率计算.vi"("偏移量"=sgl -40.0, "分辨率"=1.0, "数值 2"=w1264) -> ("输出2"=w1248:dbl)  [unwired: 3 in, 5 out]
                            n626 = Index Array(array=w1257, index #1=4 ("索引"), index #2=7 ("索引"), index #3=2 ("索引"), index #4=5 ("索引")) -> (element #1=w1256:dbl, element #2=w1255:dbl, element #3=w1241:dbl, element #4=w1254:dbl)
                            n627 = local read "充电控制参数"() -> (w1247:bool)
                            n628 = To Single Precision Float(number=w1254) -> (single precision float=w1231:sgl)
                            n629 = To Single Precision Float(number=w1248) -> (single precision float=w1230:sgl)
                            n630 = To Single Precision Float(number=w1255) -> (single precision float=w1233:sgl)
                            n631 = property class="Clust (严格)"(reference=w1258) -> (reference out=w1260:refnum<vi>, "Value"=w1261:T7)  [unwired: 1 in, 1 out]
                            n632 = Bundle By Name(cluster=w1261, "最小允许充电电流"=w1249, "电流步长"=w1236, "最小允许单体电压"=w1242, "最大允许充电温度"=w1248) -> (w1259:T7)
                            n633 = To Single Precision Float(number=w1236) -> (single precision float=w1232:sgl)
                            n634 = To Single Precision Float(number=w1249) -> (single precision float=w1234:sgl)
                            n635 = To Single Precision Float(number=w1242) -> (single precision float=w1239:sgl)
                            n636 = To Single Precision Float(number=w1256) -> (single precision float=w1235:sgl)
                            n637 = To Single Precision Float(number=w1241) -> (single precision float=w1238:sgl)
                            n638 = Equal?(x=w1231, y=w1230) -> (x = y?=w1244:bool)
                            n639 = Equal?(x=w1235, y=w1234) -> (x = y?=w1246:bool)
                            n640 = Equal?(x=w1233, y=w1232) -> (x = y?=w1245:bool)
                            n641 = Equal?(x=w1239, y=w1238) -> (x = y?=w1240:bool)
                            n642 = property class="Clust (严格)"(reference=w1260, "Value"=w1259) -> ()  [unwired: 1 in, 2 out]
                            n643 = Compound Arithmetic op=AND(w1246, w1245, w1240, w1244, w1247) -> (w1243:bool)
                            n644 = global write "读配置文件全局.vi" "充电控制参数判定"(w1243) -> ()
                          }
                        }
                      }
                      n645 = Build Array("充电控制参数     读取成功" ("字符串")) -> (w1162:string[])
                      n646 = call "表格编辑.vi"("新元素/子数组"=w1162, "活动单元格:单元格背景色"=u32 6618880, "MCListbox引用句柄"=w1160) -> ()  [unwired: 9 out]
                      n647 = global write "EV05全局变量1.vi" "写入超时"(TRUE ("写入超时")) -> ()
                    }
                  }
                }
                frame 98 {
                  n648 = case shown="6" w1300 {
                    tunnel: w1299 -> [_ w1321 w1342]
                    tunnel: w1298 -> [_ w1316 w1337]
                    tunnel: w1297 -> [_ w1309 w1330]
                    frame 0, Default {
                    }
                    frame 5 {
                      n649 = Reshape Array(w1321, 4 ("维数大小")) -> (w1313:u8[])
                      n650 = Unbundle By Name(w1316) -> ("高压参数"=w1315:refnum<vi>)
                      n651 = Index Array(array=w1313) -> (element #1=w1306:u8, element #2=w1307:u8, element #3=w1303:u8, element #4=w1304:u8)  [unwired: 4 in]
                      n652 = Join Numbers(hi=w1303, lo=w1304) -> ((hi.lo)=w1302:u16)
                      n653 = Join Numbers(hi=w1306, lo=w1307) -> ((hi.lo)=w1305:u16)
                      n654 = call "输出分辨率计算.vi"("分辨率"=0.1, "数值 2"=w1302) -> ("输出2"=w1301:dbl)  [unwired: 4 in, 5 out]
                      n655 = Build Array("电流增益     读取成功" ("字符串")) -> (w1312:string[])
                      n656 = call "表格编辑.vi"("新元素/子数组"=w1312, "活动单元格:单元格背景色"=u32 6618880, "MCListbox引用句柄"=w1309) -> ()  [unwired: 9 out]
                      n657 = property class="Clust (严格)"(reference=w1315) -> (reference out=w1318:refnum<vi>, "Value"=w1319:T8)  [unwired: 1 in, 1 out]
                      n658 = Bundle By Name(cluster=w1319, "电流增益"=w1305, "平均电流"=w1301) -> (w1317:T8)
                      n659 = global write "EV05全局变量1.vi" "写入超时"(TRUE ("写入超时")) -> ()
                      n660 = property class="Clust (严格)"(reference=w1318, "Value"=w1317) -> ()  [unwired: 1 in, 2 out]
                    }
                    frame 6 {
                      n661 = Reshape Array(w1342, 4 ("维数大小")) -> (w1334:u8[])
                      n662 = Unbundle By Name(w1337) -> ("高压参数"=w1336:refnum<vi>)
                      n663 = Index Array(array=w1334) -> (element #1=w1327:u8, element #2=w1328:u8, element #3=w1324:u8, element #4=w1325:u8)  [unwired: 4 in]
                      n664 = Join Numbers(hi=w1324, lo=w1325) -> ((hi.lo)=w1323:u16)
                      n665 = Join Numbers(hi=w1327, lo=w1328) -> ((hi.lo)=w1326:u16)
                      n666 = call "输出分辨率计算.vi"("分辨率"=0.1, "数值 2"=w1323) -> ("输出2"=w1322:dbl)  [unwired: 4 in, 5 out]
                      n667 = Build Array("电压增益     读取成功" ("字符串")) -> (w1333:string[])
                      n668 = call "表格编辑.vi"("新元素/子数组"=w1333, "活动单元格:单元格背景色"=u32 6618880, "MCListbox引用句柄"=w1330) -> ()  [unwired: 9 out]
                      n669 = property class="Clust (严格)"(reference=w1336) -> (reference out=w1339:refnum<vi>, "Value"=w1340:T8)  [unwired: 1 in, 1 out]
                      n670 = Bundle By Name(cluster=w1340, "电压增益"=w1326, "平均电压"=w1322) -> (w1338:T8)
                      n671 = global write "EV05全局变量1.vi" "写入超时"(TRUE ("写入超时")) -> ()
                      n672 = property class="Clust (严格)"(reference=w1339, "Value"=w1338) -> ()  [unwired: 1 in, 2 out]
                    }
                  }
                }
                frame 99 {
                  n673 = case shown="5" w1346 {
                    tunnel: w1345 -> [_ w1366 w1386]
                    tunnel: w1344 -> [_ w1361 w1381]
                    tunnel: w1343 -> [_ w1355 w1375]
                    frame 0, Default {
                    }
                    frame 4 {
                      n674 = Reshape Array(w1366, 4 ("维数大小")) -> (w1359:u8[])
                      n675 = Unbundle By Name(w1361) -> ("高压参数"=w1360:refnum<vi>)
                      n676 = Index Array(array=w1359) -> (element #1=w1352:u8, element #2=w1353:u8, element #3=w1350:u8, element #4=w1351:u8)  [unwired: 4 in]
                      n677 = Join Numbers(hi=w1350, lo=w1351) -> ((hi.lo)=w1348:u16)
                      n678 = Join Numbers(hi=w1352, lo=w1353) -> ((hi.lo)=w1349:u16)
                      n679 = Join Numbers(hi=w1349, lo=w1348) -> ((hi.lo)=w1347:u32)
                      n680 = Build Array("充电能量阀值     读取成功" ("字符串")) -> (w1358:string[])
                      n681 = call "表格编辑.vi"("新元素/子数组"=w1358, "活动单元格:单元格背景色"=u32 6618880, "MCListbox引用句柄"=w1355) -> ()  [unwired: 9 out]
                      n682 = property class="Clust (严格)"(reference=w1360) -> (reference out=w1363:refnum<vi>, "Value"=w1364:T8)  [unwired: 1 in, 1 out]
                      n683 = Bundle By Name(cluster=w1364, "充电能量阀值"=w1347) -> (w1362:T8)
                      n684 = global write "EV05全局变量1.vi" "写入超时"(TRUE ("写入超时")) -> ()
                      n685 = property class="Clust (严格)"(reference=w1363, "Value"=w1362) -> ()  [unwired: 1 in, 2 out]
                    }
                    frame 5 {
                      n686 = Reshape Array(w1386, 4 ("维数大小")) -> (w1379:u8[])
                      n687 = Unbundle By Name(w1381) -> ("高压参数"=w1380:refnum<vi>)
                      n688 = Index Array(array=w1379) -> (element #1=w1372:u8, element #2=w1373:u8, element #3=w1370:u8, element #4=w1371:u8)  [unwired: 4 in]
                      n689 = Join Numbers(hi=w1370, lo=w1371) -> ((hi.lo)=w1368:u16)
                      n690 = Join Numbers(hi=w1372, lo=w1373) -> ((hi.lo)=w1369:u16)
                      n691 = Join Numbers(hi=w1369, lo=w1368) -> ((hi.lo)=w1367:u32)
                      n692 = Build Array("放电能量阀值     读取成功" ("字符串")) -> (w1378:string[])
                      n693 = call "表格编辑.vi"("新元素/子数组"=w1378, "活动单元格:单元格背景色"=u32 6618880, "MCListbox引用句柄"=w1375) -> ()  [unwired: 9 out]
                      n694 = property class="Clust (严格)"(reference=w1380) -> (reference out=w1383:refnum<vi>, "Value"=w1384:T8)  [unwired: 1 in, 1 out]
                      n695 = Bundle By Name(cluster=w1384, "放电能量阀值"=w1367) -> (w1382:T8)
                      n696 = global write "EV05全局变量1.vi" "写入超时"(TRUE ("写入超时")) -> ()
                      n697 = property class="Clust (严格)"(reference=w1383, "Value"=w1382) -> ()  [unwired: 1 in, 2 out]
                    }
                  }
                }
                frame 131 {
                  n698 = disable-structure shown="禁用" {
                    disable-tunnel: w1388 -> [w1391 _]
                    disable-tunnel: w1387 -> [w1390 _]
                    disable-tunnel: _ -> [w1389 _]
                    frame Disabled {
                      n699 = case shown="2" w1391 {
                        tunnel: w1390 -> [_ w1404 w1448 w1490 w1527]
                        tunnel: w1389 -> [_ w1403 w1447 w1489 w1526]
                        tunnel: _ -> [_ w1399 w1443 w1485 w1522]
                        frame 0, Default {
                        }
                        frame 1 {
                          n700 = Reshape Array(w1404, 14 ("维数大小")) -> (w1393:u8[])
                          n701 = for {
                            N: 7 ("维数大小") -> [_]
                            tunnel: w1403 -> [w1435]
                            tunnel: [w1435] -> w1396 mode=indexing
                          }
                          n702 = for {
                            N: 7 -> [_]
                            tunnel: w1393 -> [w1413]
                            tunnel: [w1405] -> w1392 mode=indexing
                            i -> [w1409]
                            n703 = Multiply(x=w1409, y=2) -> (x*y=w1411:i32)
                            n704 = Increment(x=w1411) -> (x+1=w1410:i32)
                            n705 = Index Array(array=w1413, index #1=w1411, index #2=w1410) -> (element #1=w1408:u8, element #2=w1407:u8)
                            n706 = Join Numbers(hi=w1408, lo=w1407) -> ((hi.lo)=w1406:u16)
                            n707 = case shown="6" w1409 {
                              tunnel: w1406 -> [w1416 w1419 w1422 w1425 w1428 w1431 w1434]
                              tunnel: [w1414 w1417 w1420 w1423 w1426 w1429 w1432] -> w1405
                              frame 0, Default {
                                n708 = call "输出分辨率计算.vi"("分辨率"=0.001, "数值 2"=w1416) -> ("输出2"=w1414:dbl)  [unwired: 4 in, 5 out]
                              }
                              frame 1 {
                                n709 = call "输出分辨率计算.vi"("分辨率"=0.001, "数值 2"=w1419) -> ("输出2"=w1417:dbl)  [unwired: 4 in, 5 out]
                              }
                              frame 2 {
                                n710 = call "输出分辨率计算.vi"("分辨率"=1.0, "数值 2"=w1422) -> ("输出2"=w1420:dbl)  [unwired: 4 in, 5 out]
                              }
                              frame 3 {
                                n711 = call "输出分辨率计算.vi"("分辨率"=0.001, "数值 2"=w1425) -> ("输出2"=w1423:dbl)  [unwired: 4 in, 5 out]
                              }
                              frame 4 {
                                n712 = call "输出分辨率计算.vi"("分辨率"=0.001, "数值 2"=w1428) -> ("输出2"=w1426:dbl)  [unwired: 4 in, 5 out]
                              }
                              frame 5 {
                                n713 = call "输出分辨率计算.vi"("分辨率"=0.1, "数值 2"=w1431) -> ("输出2"=w1429:dbl)  [unwired: 4 in, 5 out]
                              }
                              frame 6 {
                                n714 = call "输出分辨率计算.vi"("分辨率"=0.1, "数值 2"=w1434) -> ("输出2"=w1432:dbl)  [unwired: 4 in, 5 out]
                              }
                            }
                          }
                          n715 = call "表格数据输入(数值)-8.6.vi"("行数"=u32 1, "列数"=u32 17, "数值数组"=w1392, "表格引用"=w1399) -> ()  [unwired: 8 out]
                          n716 = call "表格颜色-8.6.vi"("颜色类型"=w1396, "列数"=17, "行数"=1, "表格引用"=w1399) -> ()  [unwired: 1 in, 7 out]
                        }
                        frame 3 {
                          n717 = Reshape Array(w1448, 12 ("维数大小")) -> (w1437:u8[])
                          n718 = for {
                            N: 6 ("维数大小") -> [_]
                            tunnel: w1447 -> [w1477]
                            tunnel: [w1477] -> w1440 mode=indexing
                          }
                          n719 = for {
                            N: 6 -> [_]
                            tunnel: w1437 -> [w1457]
                            tunnel: [w1449] -> w1436 mode=indexing
                            i -> [w1453]
                            n720 = Multiply(x=w1453, y=2) -> (x*y=w1455:i32)
                            n721 = Increment(x=w1455) -> (x+1=w1454:i32)
                            n722 = Index Array(array=w1457, index #1=w1455, index #2=w1454) -> (element #1=w1452:u8, element #2=w1451:u8)
                            n723 = Join Numbers(hi=w1452, lo=w1451) -> ((hi.lo)=w1450:u16)
                            n724 = case shown="4, 5" w1453 {
                              tunnel: w1450 -> [w1461 w1465 w1469 w1473 w1476]
                              tunnel: [w1459 w1463 w1467 w1471 w1474] -> w1449
                              frame 0, Default {
                                n725 = call "输出分辨率计算.vi"("偏移量"=sgl -300.0, "分辨率"=0.01, "数值 2"=w1461) -> ("输出2"=w1459:dbl)  [unwired: 3 in, 5 out]
                              }
                              frame 1 {
                                n726 = call "输出分辨率计算.vi"("偏移量"=sgl -300.0, "分辨率"=0.01, "数值 2"=w1465) -> ("输出2"=w1463:dbl)  [unwired: 3 in, 5 out]
                              }
                              frame 2 {
                                n727 = call "输出分辨率计算.vi"("偏移量"=sgl -3000.0, "分辨率"=0.1, "数值 2"=w1469) -> ("输出2"=w1467:dbl)  [unwired: 3 in, 5 out]
                              }
                              frame 3 {
                                n728 = call "输出分辨率计算.vi"("偏移量"=sgl -3000.0, "分辨率"=0.1, "数值 2"=w1473) -> ("输出2"=w1471:dbl)  [unwired: 3 in, 5 out]
                              }
                              frame 4, 5 {
                                n729 = call "输出分辨率计算.vi"("分辨率"=1.0, "数值 2"=w1476) -> ("输出2"=w1474:dbl)  [unwired: 4 in, 5 out]
                              }
                            }
                          }
                          n730 = call "表格数据输入(数值)-8.6.vi"("行数"=u32 17, "列数"=u32 17, "数值数组"=w1436, "表格引用"=w1443) -> ()  [unwired: 8 out]
                          n731 = call "表格颜色-8.6.vi"("颜色类型"=w1440, "列数"=17, "行数"=17, "表格引用"=w1443) -> ()  [unwired: 1 in, 7 out]
                        }
                        frame 4 {
                          n732 = Reshape Array(w1490, 12 ("维数大小")) -> (w1479:u8[])
                          n733 = for {
                            N: 3 ("维数大小") -> [_]
                            tunnel: w1489 -> [w1515]
                            tunnel: [w1515] -> w1482 mode=indexing
                          }
                          n734 = for {
                            N: 3 -> [_]
                            tunnel: w1479 -> [w1505]
                            tunnel: [w1499] -> w1478 mode=indexing
                            i -> [w1502]
                            n735 = Multiply(x=w1502, y=4) -> (x*y=w1503:i32)
                            n736 = Increment(x=w1503) -> (x+1=w1498:i32)
                            n737 = Increment(x=w1498) -> (x+1=w1497:i32)
                            n738 = Increment(x=w1497) -> (x+1=w1496:i32)
                            n739 = Index Array(array=w1505, index #1=w1503, index #2=w1498, index #3=w1497, index #4=w1496) -> (element #1=w1501:u8, element #2=w1500:u8, element #3=w1495:u8, element #4=w1494:u8)
                            n740 = Join Numbers(hi=w1501, lo=w1500) -> ((hi.lo)=w1492:u16)
                            n741 = Join Numbers(hi=w1495, lo=w1494) -> ((hi.lo)=w1493:u16)
                            n742 = Join Numbers(hi=w1492, lo=w1493) -> ((hi.lo)=w1491:u32)
                            n743 = case shown="0, 默认" w1502 {
                              tunnel: w1491 -> [w1508 w1511 w1514]
                              tunnel: [w1506 w1509 w1512] -> w1499
                              frame 0, Default {
                                n744 = call "输出分辨率计算.vi"("分辨率"=0.001, "数值 2"=w1508) -> ("输出2"=w1506:dbl)  [unwired: 4 in, 5 out]
                              }
                              frame 1 {
                                n745 = call "输出分辨率计算.vi"("分辨率"=0.001, "数值 2"=w1511) -> ("输出2"=w1509:dbl)  [unwired: 4 in, 5 out]
                              }
                              frame 2 {
                                n746 = call "输出分辨率计算.vi"("分辨率"=0.1, "数值 2"=w1514) -> ("输出2"=w1512:dbl)  [unwired: 4 in, 5 out]
                              }
                            }
                          }
                          n747 = call "表格数据输入(数值)-8.6.vi"("行数"=u32 23, "列数"=u32 17, "数值数组"=w1478, "表格引用"=w1485) -> ()  [unwired: 8 out]
                          n748 = call "表格颜色-8.6.vi"("颜色类型"=w1482, "列数"=17, "行数"=23, "表格引用"=w1485) -> ()  [unwired: 1 in, 7 out]
                        }
                        frame 2 {
                          n749 = Reshape Array(w1527, 9 ("维数大小")) -> (w1517:u8[])
                          n750 = for {
                            N: 9 ("维数大小") -> [_]
                            tunnel: w1526 -> [w1553]
                            tunnel: [w1553] -> w1519 mode=indexing
                          }
                          n751 = for {
                            tunnel: w1517 -> [w1528] mode=indexing
                            tunnel: [w1529] -> w1516 mode=indexing
                            i -> [w1530]
                            n752 = case shown="5..8" w1530 {
                              tunnel: w1528 -> [w1534 w1538 w1541 w1545 w1549 w1552]
                              tunnel: [w1532 w1536 w1539 w1543 w1547 w1550] -> w1529
                              frame 0, Default {
                                n753 = call "输出分辨率计算.vi"("偏移量"=sgl -40.0, "分辨率"=1.0, "数值 2"=w1534) -> ("输出2"=w1532:dbl)  [unwired: 3 in, 5 out]
                              }
                              frame 1 {
                                n754 = call "输出分辨率计算.vi"("偏移量"=sgl -40.0, "分辨率"=1.0, "数值 2"=w1538) -> ("输出2"=w1536:dbl)  [unwired: 3 in, 5 out]
                              }
                              frame 2 {
                                n755 = call "输出分辨率计算.vi"("分辨率"=1.0, "数值 2"=w1541) -> ("输出2"=w1539:dbl)  [unwired: 4 in, 5 out]
                              }
                              frame 3 {
                                n756 = call "输出分辨率计算.vi"("偏移量"=sgl -40.0, "分辨率"=1.0, "数值 2"=w1545) -> ("输出2"=w1543:dbl)  [unwired: 3 in, 5 out]
                              }
                              frame 4 {
                                n757 = call "输出分辨率计算.vi"("偏移量"=sgl -40.0, "分辨率"=1.0, "数值 2"=w1549) -> ("输出2"=w1547:dbl)  [unwired: 3 in, 5 out]
                              }
                              frame 5..8 {
                                n758 = call "输出分辨率计算.vi"("分辨率"=1.0, "数值 2"=w1552) -> ("输出2"=w1550:dbl)  [unwired: 4 in, 5 out]
                              }
                            }
                          }
                          n759 = call "表格数据输入(数值)-8.6.vi"("行数"=u32 8, "列数"=u32 17, "数值数组"=w1516, "表格引用"=w1522) -> ()  [unwired: 8 out]
                          n760 = call "表格颜色-8.6.vi"("颜色类型"=w1519, "列数"=17, "行数"=8, "表格引用"=w1522) -> ()  [unwired: 1 in, 7 out]
                        }
                      }
                    }
                    frame Enabled {
                    }
                  }
                }
                frame 132 {
                  n761 = case shown="3" w1560 {
                    tunnel: w1559 -> [_ w1652 w1702 w1722 w1765]
                    tunnel: w1558 -> [_ w1649 w1696 w1715 w1753]
                    tunnel: [_ "电池信息1     读取成功" ("字符串") "电池包组号     读取成功" ("字符串") "充放电安时     读取成功" ("字符串") "电池充放电次数     读取成功" ("字符串")] -> w1554
                    frame 0, Default {
                    }
                    frame 1 {
                      w1632 = ":" ("字符串")
                      w1639 = "-" ("字符串")
                      n762 = Reshape Array(w1652, 30 ("维数大小")) -> (w1650:u8[])
                      n763 = Unbundle By Name(w1649) -> ("电池信息"=w1648:refnum<vi>)
                      n764 = global read "读配置文件全局.vi" "电池信息"() -> (w1601:T9)
                      n765 = Index Array(array=w1650) -> (element #1=w1645:u8, element #2=w1646:u8, element #3=w1597:u8, element #4=w1564:u8, element #5=w1563:u8, element #6=w1627:u8, element #7=w1626:u8, element #8=w1625:u8, element #9=w1624:u8, element #10=w1623:u8, element #11=w1622:u8, element #12=w1616:u8, element #13=w1615:u8, element #14=w1614:u8, element #15=w1613:u8, element #16=w1610:u8, element #17=w1609:u8, element #21=w1607:u8, element #22=w1606:u8, element #23=w1605:u8, element #24=w1604:u8, element #25=w1603:u8, element #26=w1602:u8)  [unwired: 26 in, 3 out]
                      n766 = Join Numbers(hi=w1623, lo=w1622) -> ((hi.lo)=w1621:u16)
                      n767 = Join Numbers(hi=w1645, lo=w1646) -> ((hi.lo)=w1599:u16)
                      n768 = Join Numbers(hi=w1614, lo=w1613) -> ((hi.lo)=w1617:u16)
                      n769 = Join Numbers(hi=w1610, lo=w1609) -> ((hi.lo)=w1608:u16)
                      n770 = Join Numbers(hi=w1625, lo=w1624) -> ((hi.lo)=w1620:u16)
                      n771 = Join Numbers(hi=w1627, lo=w1626) -> ((hi.lo)=w1582:u16)
                      n772 = Join Numbers(hi=w1616, lo=w1615) -> ((hi.lo)=w1612:u16)
                      n773 = Unbundle By Name(w1601) -> ("电池串联"=w1600:dbl, "电池并联"=w1598:dbl, "电池厂家"=w1576:string, "电池类型"=w1574:string, "电池包额定能量"=w1596:dbl, "电池包额定容量"=w1594:dbl, "实际容量"=w1593:dbl, "电池包额定总电压"=w1592:dbl)
                      n774 = Join Numbers(hi=w1620, lo=w1621) -> ((hi.lo)=w1619:u32)
                      n775 = Join Numbers(hi=w1612, lo=w1617) -> ((hi.lo)=w1618:u32)
                      n776 = To Double Precision Float(number=w1619) -> (double precision float=w1581:dbl)
                      n777 = To Double Precision Float(number=w1618) -> (double precision float=w1580:dbl)
                      n778 = Number To Decimal String(number=w1564) -> (decimal integer string=w1562:string)  [unwired: 1 in]
                      n779 = Number To Decimal String(number=w1563) -> (decimal integer string=w1561:string)  [unwired: 1 in]
                      n780 = call "输出分辨率计算.vi"("数值1"=w1582, "分辨率"=0.1, "数值 4"=w1608) -> ("输出4"=w1591:dbl, "输出1"=w1595:dbl)  [unwired: 3 in, 4 out]
                      n781 = case shown="1" w1563 {
                        tunnel: [_ "磷酸铁锂" "锰酸锂" "三元材料" "铅酸" "镍氢" "钴酸锂" "聚合物锂离子" "钛酸锂" "其他电池"] -> w1573
                        frame 0, Default {
                        }
                        frame 1 {
                        }
                        frame 2 {
                        }
                        frame 3 {
                        }
                        frame 4 {
                        }
                        frame 5 {
                        }
                        frame 6 {
                        }
                        frame 7 {
                        }
                        frame 8 {
                        }
                        frame 9 {
                        }
                      }
                      n782 = case shown="1" w1564 {
                        tunnel: [_ "普莱德" "盟固利"] -> w1575
                        frame 0, Default {
                        }
                        frame 1 {
                        }
                        frame 2 {
                        }
                      }
                      n783 = Number To Decimal String(number=w1607) -> (decimal integer string=w1640:string)  [unwired: 1 in]
                      n784 = Number To Decimal String(number=w1606) -> (decimal integer string=w1638:string)  [unwired: 1 in]
                      n785 = Number To Decimal String(number=w1604) -> (decimal integer string=w1633:string)  [unwired: 1 in]
                      n786 = Number To Decimal String(number=w1605) -> (decimal integer string=w1637:string)  [unwired: 1 in]
                      n787 = Number To Decimal String(number=w1603) -> (decimal integer string=w1634:string)  [unwired: 1 in]
                      n788 = Number To Decimal String(number=w1602) -> (decimal integer string=w1635:string)  [unwired: 1 in]
                      n789 = call "输出分辨率计算.vi"("分辨率"=0.001, "数值 3"=w1580, "数值 2"=w1581) -> ("输出3"=w1577:dbl, "输出2"=w1578:dbl)  [unwired: 3 in, 4 out]
                      n790 = To Single Precision Float(number=w1593) -> (single precision float=w1570:sgl)
                      n791 = To Single Precision Float(number=w1592) -> (single precision float=w1569:sgl)
                      n792 = To Single Precision Float(number=w1596) -> (single precision float=w1572:sgl)
                      n793 = To Single Precision Float(number=w1594) -> (single precision float=w1571:sgl)
                      n794 = Concatenate Strings("20" ("字符串"), w1640, w1639, w1638, w1639, w1637) -> (w1631:string)
                      n795 = Concatenate Strings(w1633, w1632, w1634, w1632, w1635) -> (w1630:string)
                      n796 = call <vilib>:"Space Constant.vi"() -> ("String"=w1629:string)
                      n797 = To Single Precision Float(number=w1591) -> (single precision float=w1565:sgl)
                      n798 = To Single Precision Float(number=w1577) -> (single precision float=w1566:sgl)
                      n799 = Concatenate Strings(w1631, w1629, w1630) -> (w1628:string)
                      n800 = To Single Precision Float(number=w1595) -> (single precision float=w1568:sgl)
                      n801 = To Single Precision Float(number=w1578) -> (single precision float=w1567:sgl)
                      n802 = stacked-sequence {
                        seq-local: [w1653 _] -> [_ w1664]
                        seq-local: [w1654 _] -> [_ w1661]
                        tunnel: [_ w1660] -> _
                        tunnel: [_ w1659] -> w1590
                        tunnel: w1576 -> [w1658 w1668]
                        tunnel: w1575 -> [w1657 _]
                        tunnel: w1574 -> [w1656 w1667]
                        tunnel: w1573 -> [w1655 _]
                        tunnel: w1562 -> [_ w1666]
                        tunnel: w1561 -> [_ w1665]
                        frame #0 {
                          n803 = Equal?(x=w1657, y=w1658) -> (x = y?=w1654:bool)
                          n804 = Equal?(x=w1655, y=w1656) -> (x = y?=w1653:bool)
                        }
                        frame #1 {
                          n805 = Equal?(x=w1665, y=w1667) -> (x = y?=w1663:bool)
                          n806 = Equal?(x=w1666, y=w1668) -> (x = y?=w1662:bool)
                          n807 = Or(x=w1661, y=w1662) -> (x .or. y?=w1660:bool)
                          n808 = Or(x=w1663, y=w1664) -> (x .or. y?=w1659:bool)
                        }
                      }
                      n809 = Equal?(x=w1600, y=w1599) -> (x = y?=w1589:bool)
                      n810 = Equal?(x=w1598, y=w1597) -> (x = y?=w1588:bool)
                      n811 = property class="Clust (严格)"(reference=w1648) -> (reference out=w1643:refnum<vi>, "Value"=w1644:T9)  [unwired: 1 in, 1 out]
                      n812 = Bundle By Name(cluster=w1644, "电池串联"=w1599, "电池并联"=w1597, "电池厂家"=w1575, "电池类型"=w1573, "电池包额定能量"=w1595, "电池包额定容量"=w1578, "实际容量"=w1577, "电池包额定总电压"=w1591, "电池生产日期"=w1628) -> (w1642:T9)
                      n813 = Equal?(x=w1572, y=w1568) -> (x = y?=w1587:bool)
                      n814 = Equal?(x=w1567, y=w1571) -> (x = y?=w1586:bool)
                      n815 = Equal?(x=w1570, y=w1566) -> (x = y?=w1585:bool)
                      n816 = Equal?(x=w1569, y=w1565) -> (x = y?=w1584:bool)
                      n817 = property class="Clust (严格)"(reference=w1643, "Value"=w1642) -> ()  [unwired: 1 in, 2 out]
                      n818 = global write "EV05全局变量1.vi" "写入超时"(TRUE ("写入超时")) -> ()
                      n819 = Compound Arithmetic op=AND(w1590, w1589, w1588, w1587, w1586, w1585, w1584) -> (w1583:bool)
                      n820 = global write "读配置文件全局.vi" "电池信息1判定"(w1583) -> ()
                    }
                    frame 2 {
                      n821 = Reshape Array(w1702, 4 ("维数大小")) -> (w1700:u8[])
                      n822 = Unbundle By Name(w1696) -> ("电池信息"=w1695:refnum<vi>)
                      n823 = global read "读配置文件全局.vi" "电池信息"() -> (w1688:T9)
                      n824 = Index Array(array=w1700) -> (element #1=w1693:u8, element #2=w1694:u8, element #3=w1691:u8, element #4=w1692:u8)  [unwired: 4 in]
                      n825 = Join Numbers(hi=w1693, lo=w1694) -> ((hi.lo)=w1686:u16)
                      n826 = Join Numbers(hi=w1691, lo=w1692) -> ((hi.lo)=w1685:u16)
                      n827 = Unbundle By Name(w1688) -> ("电池包组号"=w1682:string)
                      n828 = Join Numbers(hi=w1686, lo=w1685) -> ((hi.lo)=w1684:u32)
                      n829 = Number To Decimal String(number=w1684) -> (decimal integer string=w1683:string)  [unwired: 1 in]
                      n830 = Match Pattern(string=w1682, regular expression="-" ("正则表达式")) -> (before substring=w1681:string)  [unwired: 1 in, 3 out]
                      n831 = Equal?(x=w1683, y=w1681) -> (x = y?=w1687:bool)
                      n832 = global write "读配置文件全局.vi" "电池包组号判定"(w1687) -> ()
                      n833 = property class="Clust (严格)"(reference=w1695) -> (reference out=w1698:refnum<vi>, "Value"=w1699:T9)  [unwired: 1 in, 1 out]
                      n834 = Bundle By Name(cluster=w1699, "电池包组号"=w1683) -> (w1697:T9)
                      n835 = global write "EV05全局变量1.vi" "写入超时"(TRUE ("写入超时")) -> ()
                      n836 = property class="Clust (严格)"(reference=w1698, "Value"=w1697) -> ()  [unwired: 1 in, 2 out]
                    }
                    frame 3 {
                      n837 = Reshape Array(w1722, 8 ("维数大小")) -> (w1720:u8[])
                      n838 = Unbundle By Name(w1715) -> ("电池信息"=w1714:refnum<vi>)
                      n839 = for {
                        N: 2 -> [_]
                        tunnel: w1720 -> [w1738]
                        tunnel: [w1723] -> w1713 mode=indexing
                        i -> [w1735]
                        n840 = Multiply(x=w1735, y=4) -> (x*y=w1736:i32)
                        n841 = Increment(x=w1736) -> (x+1=w1732:i32)
                        n842 = Increment(x=w1732) -> (x+1=w1731:i32)
                        n843 = Increment(x=w1731) -> (x+1=w1730:i32)
                        n844 = Index Array(array=w1738, index #1=w1736, index #2=w1732, index #3=w1731, index #4=w1730) -> (element #1=w1734:u8, element #2=w1733:u8, element #3=w1729:u8, element #4=w1728:u8)
                        n845 = Join Numbers(hi=w1734, lo=w1733) -> ((hi.lo)=w1726:u16)
                        n846 = Join Numbers(hi=w1729, lo=w1728) -> ((hi.lo)=w1727:u16)
                        n847 = Join Numbers(hi=w1726, lo=w1727) -> ((hi.lo)=w1724:u32)
                        n848 = call "输出分辨率计算.vi"("分辨率"=0.001, "数值 2"=w1724) -> ("输出2"=w1723:dbl)  [unwired: 4 in, 5 out]
                      }
                      n849 = global read "读配置文件全局.vi" "电池信息"() -> (w1710:T9)
                      n850 = Unbundle By Name(w1710) -> ("累计充电总安时"=w1709:dbl, "累计放电总安时"=w1708:dbl)
                      n851 = Index Array(array=w1713) -> (element #1=w1706:dbl, element #2=w1707:dbl)  [unwired: 2 in]
                      n852 = Equal?(x=w1706, y=w1709) -> (x = y?=w1704:bool)
                      n853 = Equal?(x=w1708, y=w1707) -> (x = y?=w1705:bool)
                      n854 = global write "EV05全局变量1.vi" "写入超时"(TRUE ("写入超时")) -> ()
                      n855 = And(x=w1704, y=w1705) -> ()  [unwired: 1 out]
                      n856 = property class="Clust (严格)"(reference=w1714) -> (reference out=w1717:refnum<vi>, "Value"=w1718:T9)  [unwired: 1 in, 1 out]
                      n857 = Bundle By Name(cluster=w1718, "累计充电总安时"=w1706, "累计放电总安时"=w1707) -> (w1716:T9)
                      n858 = global write "读配置文件全局.vi" "充放电安时判定"(TRUE ("充放电安时判定")) -> ()
                      n859 = property class="Clust (严格)"(reference=w1717, "Value"=w1716) -> ()  [unwired: 1 in, 2 out]
                    }
                    frame 4 {
                      n860 = global read "读配置文件全局.vi" "电池信息"() -> (w1749:T9)
                      n861 = Reshape Array(w1765, 6 ("维数大小")) -> (w1763:u8[])
                      n862 = Unbundle By Name(w1753) -> ("电池信息"=w1752:refnum<vi>)
                      n863 = Index Array(array=w1763) -> (element #1=w1761:u8, element #2=w1762:u8, element #3=w1760:u8, element #4=w1759:u8, element #5=w1758:u8, element #6=w1757:u8)  [unwired: 6 in]
                      n864 = Unbundle By Name(w1749) -> ("电池放空次数"=w1748:dbl, "电池充满次数"=w1747:dbl, "电池充电次数"=w1744:dbl)
                      n865 = Join Numbers(hi=w1761, lo=w1762) -> ((hi.lo)=w1746:u16)
                      n866 = Join Numbers(hi=w1760, lo=w1759) -> ((hi.lo)=w1745:u16)
                      n867 = Join Numbers(hi=w1758, lo=w1757) -> ((hi.lo)=w1743:u16)
                      n868 = Equal?(x=w1746, y=w1748) -> (x = y?=w1742:bool)
                      n869 = Equal?(x=w1747, y=w1745) -> (x = y?=w1741:bool)
                      n870 = Equal?(x=w1744, y=w1743) -> (x = y?=w1740:bool)
                      n871 = property class="Clust (严格)"(reference=w1752) -> (reference out=w1755:refnum<vi>, "Value"=w1756:T9)  [unwired: 1 in, 1 out]
                      n872 = Bundle By Name(cluster=w1756, "电池放空次数"=w1746, "电池充满次数"=w1745, "电池充电次数"=w1743) -> (w1754:T9)
                      n873 = Compound Arithmetic op=AND(w1742, w1741, w1740) -> ()  [unwired: 1 out]
                      n874 = global write "读配置文件全局.vi" "电池充放电次数判定"(TRUE ("电池充放电次数判定")) -> ()
                      n875 = property class="Clust (严格)"(reference=w1755, "Value"=w1754) -> ()  [unwired: 1 in, 2 out]
                      n876 = global write "EV05全局变量1.vi" "写入超时"(TRUE ("写入超时")) -> ()
                    }
                  }
                  n877 = Build Array(w1554) -> (w1557:string[])
                  n878 = call "表格编辑.vi"("新元素/子数组"=w1557, "活动单元格:单元格背景色"=u32 6618880, "MCListbox引用句柄"=w1555) -> ()  [unwired: 9 out]
                }
                frame 192 {
                  n879 = Index Array(array=w1769) -> (element #1=→"序号":u8, element #2=w1767:u8)  [unwired: 2 in]
                  n880 = Not Equal To 0?(x=w1767) -> (x != 0?=→"状态":bool)
                }
                frame 140 {
                  n881 = Array Subset(array=w1780, length=30 ("长度")) -> (w1778:u8[])  [unwired: 1 in]
                  n882 = Byte Array To String(unsigned byte array=w1778) -> (string=w1772:string)
                  n883 = Concatenate Strings("BNET" ("字符串"), w1772) -> (w1771:string)
                  n884 = property class="Str"(reference="二维码信息", "Text.Text"=w1771) -> ()  [unwired: 1 in, 2 out]
                  n885 = global write "EV05全局变量1.vi" "写入超时"(TRUE ("写入超时")) -> ()
                  n886 = Build Array("二维码     读取成功" ("字符串")) -> (w1776:string[])
                  n887 = call "表格编辑.vi"("新元素/子数组"=w1776, "活动单元格:单元格背景色"=u32 6618880, "MCListbox引用句柄"=w1773) -> ()  [unwired: 9 out]
                }
              }
            }
            frame True {
            }
          }
        }
        frame "从板" {
          n888 = Not A Number/Path/Refnum?(number/path/refnum=w1783) -> (NaN/Path/Refnum?=w1782:bool)
          n889 = case shown="假" w1782 {
            tunnel: w1787 -> [w1793 _]
            tunnel: w1786 -> [w1792 _]
            tunnel: w1785 -> [w1791 _]
            tunnel: w1783 -> [w1789 _]
            tunnel: w1784 -> [w1788 _]
            frame False {
              n890 = property class="Clust (严格)"(reference=w1789) -> ("Value"=w1790:T1)  [unwired: 1 in, 2 out]
              n891 = case shown="A" w1793 {
                tunnel: w1792 -> [_ w1800 w1947 w2154 _ w2369]
                tunnel: w1790 -> [_ w1799 w1945 w2152 _ w2367]
                tunnel: w1791 -> [_ w1798 w1946 w2153 w2352 w2368]
                tunnel: w1788 -> [_ w1795 w1944 w2149 w2351 w2364]
                frame 153, Default {
                }
                frame 0 {
                  n892 = case shown="4" w1800 {
                    tunnel: w1799 -> [_ w1820 w1839 w1859 w1892 w1932 w1941]
                    tunnel: w1798 -> [_ w1818 w1836 w1856 w1889 w1934 w1943]
                    tunnel: [_ "电压起始值     读取成功" ("字符串") "通道电压节数     读取成功" ("字符串") "保险位置     读取成功" ("字符串") "温度起始值     读取成功" ("字符串") "加热控制参数     读取成功" ("字符串") "从板号     读取成功" ("字符串")] -> w1794
                    frame 0, Default {
                    }
                    frame 1 {
                      n893 = Unbundle By Name(w1820) -> ("项目信息 2"=w1819:refnum<vi>)
                      n894 = global read "读配置文件全局2.vi" "表格"() -> (w1808:string[])
                      n895 = Array Subset(array=w1818, length=4 ("长度")) -> (w1816:u8[])  [unwired: 1 in]
                      n896 = Array Subset(array=w1808, index=0 ("索引"), length=1 ("长度")) -> (w1805:string[])
                      n897 = Index Array(array=w1816) -> (element #1=w1814:u8, element #2=w1815:u8, element #3=w1813:u8, element #4=w1812:u8)  [unwired: 4 in]
                      n898 = for {
                        tunnel: w1805 -> [w1824] mode=indexing
                        tunnel: [w1823] -> w1804 mode=indexing
                        n899 = Fract/Exp String To Number(string=w1824) -> (number=w1823:dbl)  [unwired: 4 out]
                      }
                      n900 = Join Numbers(hi=w1814, lo=w1815) -> ((hi.lo)=w1811:u16)
                      n901 = Join Numbers(hi=w1813, lo=w1812) -> ()  [unwired: 1 out]
                      n902 = Build Array(w1811) -> (w1803:u16[])
                      n903 = Equal?(x=w1803, y=w1804) -> (x = y?=w1802:bool[])
                      n904 = And Array Elements(Boolean array=w1802) -> (logical AND=w1801:bool)
                      n905 = global write "读配置文件全局2.vi" "电压起始值判定"(w1801) -> ()
                      n906 = global write "EV05全局变量1.vi" "写入超时"(TRUE ("写入超时")) -> ()
                      n907 = call "表格数据输入(数值)-8.6.vi"("行数"=u32 0, "列数"=u32 1, "数值数组"=w1803, "表格引用"=w1819) -> ()  [unwired: 8 out]
                    }
                    frame 2 {
                      n908 = Unbundle By Name(w1839) -> ("项目信息 2"=w1838:refnum<vi>)
                      n909 = Array Subset(array=w1836, length=5 ("长度")) -> (w1825:u8[])  [unwired: 1 in]
                      n910 = global read "读配置文件全局2.vi" "表格"() -> (w1832:string[])
                      n911 = Array Subset(array=w1832, index=22 ("索引"), length=5 ("长度")) -> (w1829:string[])
                      n912 = for {
                        tunnel: w1829 -> [w1842] mode=indexing
                        tunnel: [w1841] -> w1828 mode=indexing
                        n913 = Fract/Exp String To Number(string=w1842) -> (number=w1841:dbl)  [unwired: 4 out]
                      }
                      n914 = Equal?(x=w1825, y=w1828) -> (x = y?=w1827:bool[])
                      n915 = And Array Elements(Boolean array=w1827) -> (logical AND=w1826:bool)
                      n916 = global write "EV05全局变量1.vi" "写入超时"(TRUE ("写入超时")) -> ()
                      n917 = global write "读配置文件全局2.vi" "通道电压判定"(w1826) -> ()
                      n918 = call "表格数据输入(数值)-8.6.vi"("行数"=u32 22, "列数"=u32 1, "数值数组"=w1825, "表格引用"=w1838) -> ()  [unwired: 8 out]
                    }
                    frame 3 {
                      n919 = Unbundle By Name(w1859) -> ("项目信息 2"=w1858:refnum<vi>)
                      n920 = Array Subset(array=w1856, length=10 ("长度")) -> (w1845:u8[])  [unwired: 1 in]
                      n921 = for {
                        tunnel: w1845 -> [w1869] mode=indexing
                        shift-right: [w1862] -> w1843
                        shift-left: i32[] [] -> [w1861]
                        n922 = call "二进制解析-8.6.vi"("索引"=4, "数值"=w1869) -> ("低位子数组"=w1867:i32[], "高位子数组"=w1866:i32[])  [unwired: 1 in, 1 out]
                        n923 = call "数值二进制转十进制-8.6.vi"("子数组"=w1866) -> ("十进制数值"=w1865:i32)  [unwired: 4 in]
                        n924 = call "数值二进制转十进制-8.6.vi"("子数组"=w1867) -> ("十进制数值"=w1864:i32)  [unwired: 4 in]
                        n925 = Build Array(w1865, w1864) -> (w1863:i32[])
                        n926 = Insert Into Array(array=w1861, new element=w1863) -> (w1862:i32[])  [unwired: 1 in]
                      }
                      n927 = global read "读配置文件全局2.vi" "表格"() -> (w1852:string[])
                      n928 = Array Subset(array=w1852, index=2 ("索引"), length=20 ("长度")) -> (w1849:string[])
                      n929 = for {
                        tunnel: w1849 -> [w1871] mode=indexing
                        tunnel: [w1870] -> w1848 mode=indexing
                        n930 = Fract/Exp String To Number(string=w1871) -> (number=w1870:dbl)  [unwired: 4 out]
                      }
                      n931 = global write "EV05全局变量1.vi" "写入超时"(TRUE ("写入超时")) -> ()
                      n932 = Equal?(x=w1843, y=w1848) -> (x = y?=w1847:bool[])
                      n933 = And Array Elements(Boolean array=w1847) -> (logical AND=w1846:bool)
                      n934 = global write "读配置文件全局2.vi" "保险位置判定"(w1846) -> ()
                      n935 = call "表格数据输入(数值)-8.6.vi"("行数"=u32 2, "列数"=u32 1, "数值数组"=w1843, "表格引用"=w1858) -> ()  [unwired: 8 out]
                    }
                    frame 4 {
                      n936 = Unbundle By Name(w1892) -> ("项目信息 2"=w1891:refnum<vi>)
                      n937 = Array Subset(array=w1889, length=4 ("长度")) -> (w1887:u8[])  [unwired: 1 in]
                      n938 = global read "读配置文件全局2.vi" "表格"() -> (w1879:string[])
                      n939 = Index Array(array=w1887) -> (element #1=w1885:u8, element #2=w1886:u8, element #3=w1883:u8, element #4=w1884:u8)  [unwired: 4 in]
                      n940 = Join Numbers(hi=w1883, lo=w1884) -> ()  [unwired: 1 out]
                      n941 = Join Numbers(hi=w1885, lo=w1886) -> ((hi.lo)=w1882:u16)
                      n942 = Array Subset(array=w1879, index=1 ("索引"), length=1 ("长度")) -> (w1876:string[])
                      n943 = Build Array(w1882) -> (w1872:u16[])
                      n944 = for {
                        tunnel: w1876 -> [w1895] mode=indexing
                        tunnel: [w1894] -> w1875 mode=indexing
                        n945 = Fract/Exp String To Number(string=w1895) -> (number=w1894:dbl)  [unwired: 4 out]
                      }
                      n946 = Equal?(x=w1872, y=w1875) -> (x = y?=w1874:bool[])
                      n947 = global write "EV05全局变量1.vi" "写入超时"(TRUE ("写入超时")) -> ()
                      n948 = And Array Elements(Boolean array=w1874) -> (logical AND=w1873:bool)
                      n949 = global write "读配置文件全局2.vi" "温度起始值判定"(w1873) -> ()
                      n950 = call "表格数据输入(数值)-8.6.vi"("行数"=u32 1, "列数"=u32 1, "数值数组"=w1872, "表格引用"=w1891) -> ()  [unwired: 8 out]
                    }
                    frame 5 {
                      n951 = global read "读配置文件全局2.vi" "加热控制参数"() -> (w1920:dbl[])
                      n952 = Unbundle By Name(w1932) -> ("加热控制参数"=w1928:refnum<vi>)
                      n953 = Array Subset(array=w1934, length=7 ("索引")) -> (w1927:u8[])  [unwired: 1 in]
                      n954 = Index Array(array=w1927) -> (element #1=w1926:u8, element #2=w1925:u8, element #3=w1900:u8, element #4=w1899:u8, element #5=w1902:u8, element #6=w1901:u8, element #7=w1897:u8)  [unwired: 7 in]
                      n955 = Index Array(array=w1920) -> (element #1=w1919:dbl, element #2=w1917:dbl, element #3=w1916:dbl, element #4=w1915:dbl, element #5=w1914:dbl, element #6=w1913:dbl, element #7=w1898:dbl)  [unwired: 7 in]
                      n956 = call "输出分辨率计算.vi"("偏移量"=sgl -40.0, "数值1"=w1926, "分辨率"=1.0, "数值 4"=w1901, "数值 3"=w1902, "数值 2"=w1925) -> ("输出4"=w1910:dbl, "输出3"=w1911:dbl, "输出2"=w1912:dbl, "输出1"=w1918:dbl)  [unwired: 2 out]
                      n957 = property class="Clust (严格)"(reference=w1928) -> (reference out=w1930:refnum<vi>, "Value"=w1931:T6)  [unwired: 1 in, 1 out]
                      n958 = Equal?(x=w1914, y=w1900) -> (x = y?=w1905:bool)
                      n959 = Equal?(x=w1913, y=w1899) -> (x = y?=w1904:bool)
                      n960 = Equal?(x=w1919, y=w1918) -> (x = y?=w1909:bool)
                      n961 = Equal?(x=w1917, y=w1912) -> (x = y?=w1908:bool)
                      n962 = Equal?(x=w1916, y=w1911) -> (x = y?=w1907:bool)
                      n963 = Equal?(x=w1915, y=w1910) -> (x = y?=w1906:bool)
                      n964 = Equal?(x=w1898, y=w1897) -> (x = y?=w1896:bool)
                      n965 = Bundle By Name(cluster=w1931, "风机开启温度"=w1918, "风机关闭温度"=w1912, "加热开启温度"=w1911, "加热关闭温度"=w1910, "风机开启温差"=w1900, "风机关闭温差"=w1899, "加热关闭温差"=w1897) -> (w1929:T6)
                      n966 = Compound Arithmetic op=AND(w1909, w1908, w1907, w1906, w1905, w1904, w1896) -> (w1903:bool)
                      n967 = global write "读配置文件全局2.vi" "加热控制参数判定"(w1903) -> ()
                      n968 = property class="Clust (严格)"(reference=w1930, "Value"=w1929) -> ()  [unwired: 1 in, 2 out]
                      n969 = global write "EV05全局变量1.vi" "写入超时"(TRUE ("写入超时")) -> ()
                    }
                    frame 6 {
                      n970 = Index Array(array=w1943, index=0 ("索引")) -> (element=w1936:u8)
                      n971 = Unbundle By Name(w1941) -> ("从板号"=w1940:refnum<vi>)
                      n972 = global read "读配置文件全局2.vi" "从板板号"() -> (w1937:dbl)
                      n973 = Equal?(x=w1936, y=w1937) -> (x = y?=w1935:bool)
                      n974 = property class="DigNum (严格)"(reference=w1940, "Value"=w1936) -> ()  [unwired: 1 in, 2 out]
                      n975 = global write "读配置文件全局2.vi" "从板号判定"(w1935) -> ()
                      n976 = global write "EV05全局变量1.vi" "写入超时"(TRUE ("写入超时")) -> ()
                    }
                  }
                  n977 = Build Array(w1794) -> (w1797:string[])
                  n978 = call "表格编辑.vi"("新元素/子数组"=w1797, "活动单元格:单元格背景色"=u32 6618880, "MCListbox引用句柄"=w1795) -> ()  [unwired: 9 out]
                }
                frame 2 {
                  n979 = case shown="1" w1947 {
                    tunnel: w1946 -> [_ w2013 w2081 w2147]
                    tunnel: w1945 -> [_ w1993 w2061 w2127]
                    tunnel: w1944 -> [_ w1988 w2056 w2122]
                    frame 0, Default {
                    }
                    frame 1 {
                      n980 = Unbundle By Name(w1993) -> ("一级故障(从板)"=w1992:refnum<vi>)
                      n981 = global read "读配置文件全局2.vi" "一级故障阀值"() -> (w1983:dbl[])
                      n982 = Index Array(array=w2013, index #1=0 ("长度")) -> (element #1=w2010:u8, element #2=w2011:u8, element #3=w2009:u8, element #4=w2008:u8, element #5=w2007:u8, element #6=w2006:u8, element #7=w2002:u8, element #8=w2001:u8, element #9=w1970:u8, element #10=w1986:u8, element #11=w1987:u8)  [unwired: 10 in]
                      n983 = Join Numbers(hi=w2010, lo=w2011) -> ((hi.lo)=w2005:u16)
                      n984 = Join Numbers(hi=w2009, lo=w2008) -> ((hi.lo)=w2004:u16)
                      n985 = Join Numbers(hi=w2007, lo=w2006) -> ((hi.lo)=w1998:u16)
                      n986 = Join Numbers(hi=w1986, lo=w1987) -> ((hi.lo)=w1985:u16)
                      n987 = call "输出分辨率计算.vi"("分辨率"=0.1, "数值 2"=w1985) -> ("输出2"=w1969:dbl)  [unwired: 4 in, 5 out]
                      n988 = Index Array(array=w1983) -> (element #1=w1982:dbl, element #2=w1981:dbl, element #3=w1980:dbl, element #4=w1979:dbl, element #5=w1978:dbl, element #6=w1977:dbl, element #7=w1976:dbl)  [unwired: 7 in]
                      n989 = call "输出分辨率计算.vi"("分辨率"=0.001, "数值 4"=w1998, "数值 3"=w2004, "数值 2"=w2005) -> ("输出4"=w1971:dbl, "输出3"=w1974:dbl, "输出2"=w1975:dbl)  [unwired: 2 in, 3 out]
                      n990 = call "输出分辨率计算.vi"("偏移量"=sgl -40.0, "分辨率"=1.0, "数值 3"=w2001, "数值 2"=w2002) -> ("输出3"=w1972:dbl, "输出2"=w1973:dbl)  [unwired: 2 in, 4 out]
                      n991 = To Single Precision Float(number=w1978) -> (single precision float=w1952:sgl)
                      n992 = To Single Precision Float(number=w1977) -> (single precision float=w1950:sgl)
                      n993 = To Single Precision Float(number=w1976) -> (single precision float=w1949:sgl)
                      n994 = To Single Precision Float(number=w1969) -> (single precision float=w1948:sgl)
                      n995 = To Single Precision Float(number=w1971) -> (single precision float=w1951:sgl)
                      n996 = To Single Precision Float(number=w1979) -> (single precision float=w1954:sgl)
                      n997 = To Single Precision Float(number=w1972) -> (single precision float=w1953:sgl)
                      n998 = To Single Precision Float(number=w1980) -> (single precision float=w1956:sgl)
                      n999 = To Single Precision Float(number=w1973) -> (single precision float=w1955:sgl)
                      n1000 = To Single Precision Float(number=w1982) -> (single precision float=w1960:sgl)
                      n1001 = To Single Precision Float(number=w1981) -> (single precision float=w1958:sgl)
                      n1002 = To Single Precision Float(number=w1974) -> (single precision float=w1957:sgl)
                      n1003 = To Single Precision Float(number=w1975) -> (single precision float=w1959:sgl)
                      n1004 = Build Array("一级故障阀值     读取成功" ("字符串")) -> (w1991:string[])
                      n1005 = property class="Clust (严格)"(reference=w1992) -> (reference out=w1995:refnum<vi>, "Value"=w1996:T10)  [unwired: 1 in, 1 out]
                      n1006 = Equal?(x=w1960, y=w1959) -> (x = y?=w1968:bool)
                      n1007 = Equal?(x=w1958, y=w1957) -> (x = y?=w1967:bool)
                      n1008 = Equal?(x=w1956, y=w1955) -> (x = y?=w1966:bool)
                      n1009 = Equal?(x=w1954, y=w1953) -> (x = y?=w1965:bool)
                      n1010 = Equal?(x=w1952, y=w1951) -> (x = y?=w1964:bool)
                      n1011 = Equal?(x=w1950, y=w1970) -> (x = y?=w1963:bool)
                      n1012 = Equal?(x=w1949, y=w1948) -> (x = y?=w1962:bool)
                      n1013 = Bundle By Name(cluster=w1996, "电压过高"=w1975, "电压过低"=w1974, "温度过高"=w1973, "温度过低"=w1972, "电压不均衡(V)"=w1971, "温度不均衡"=w1970, "SOC过低"=w1969) -> (w1994:T10)
                      n1014 = call "表格编辑.vi"("新元素/子数组"=w1991, "活动单元格:单元格背景色"=u32 6618880, "MCListbox引用句柄"=w1988) -> ()  [unwired: 9 out]
                      n1015 = Compound Arithmetic op=AND(w1968, w1967, w1966, w1965, w1964, w1963, w1962) -> (w1961:bool)
                      n1016 = property class="Clust (严格)"(reference=w1995, "Value"=w1994) -> ()  [unwired: 1 in, 2 out]
                      n1017 = global write "读配置文件全局2.vi" "一级故障判定"(w1961) -> ()
                      n1018 = global write "EV05全局变量1.vi" "写入超时"(TRUE ("写入超时")) -> ()
                    }
                    frame 2 {
                      n1019 = Unbundle By Name(w2061) -> ("二级故障(从板)"=w2060:refnum<vi>)
                      n1020 = Index Array(array=w2081, index #1=0 ("长度")) -> (element #1=w2078:u8, element #2=w2079:u8, element #3=w2077:u8, element #4=w2076:u8, element #5=w2075:u8, element #6=w2074:u8, element #7=w2070:u8, element #8=w2069:u8, element #9=w2030:u8, element #10=w2055:u8, element #11=w2054:u8)  [unwired: 10 in]
                      n1021 = global read "读配置文件全局2.vi" "二级故障阀值"() -> (w2051:dbl[])
                      n1022 = Join Numbers(hi=w2078, lo=w2079) -> ((hi.lo)=w2073:u16)
                      n1023 = Join Numbers(hi=w2077, lo=w2076) -> ((hi.lo)=w2072:u16)
                      n1024 = Join Numbers(hi=w2075, lo=w2074) -> ((hi.lo)=w2066:u16)
                      n1025 = Join Numbers(hi=w2055, lo=w2054) -> ((hi.lo)=w2053:u16)
                      n1026 = call "输出分辨率计算.vi"("分辨率"=0.1, "数值 2"=w2053) -> ("输出2"=w2029:dbl)  [unwired: 4 in, 5 out]
                      n1027 = Index Array(array=w2051) -> (element #1=w2050:dbl, element #2=w2049:dbl, element #3=w2048:dbl, element #4=w2047:dbl, element #5=w2046:dbl, element #6=w2045:dbl, element #7=w2044:dbl)  [unwired: 7 in]
                      n1028 = call "输出分辨率计算.vi"("分辨率"=0.001, "数值 4"=w2066, "数值 3"=w2072, "数值 2"=w2073) -> ("输出4"=w2031:dbl, "输出3"=w2034:dbl, "输出2"=w2035:dbl)  [unwired: 2 in, 3 out]
                      n1029 = call "输出分辨率计算.vi"("偏移量"=sgl -40.0, "分辨率"=1.0, "数值 3"=w2069, "数值 2"=w2070) -> ("输出3"=w2032:dbl, "输出2"=w2033:dbl)  [unwired: 2 in, 4 out]
                      n1030 = To Single Precision Float(number=w2034) -> (single precision float=w2027:sgl)
                      n1031 = To Single Precision Float(number=w2049) -> (single precision float=w2028:sgl)
                      n1032 = Build Array("二级故障阀值     读取成功" ("字符串")) -> (w2059:string[])
                      n1033 = To Single Precision Float(number=w2031) -> (single precision float=w2017:sgl)
                      n1034 = To Single Precision Float(number=w2044) -> (single precision float=w2015:sgl)
                      n1035 = To Single Precision Float(number=w2047) -> (single precision float=w2020:sgl)
                      n1036 = To Single Precision Float(number=w2046) -> (single precision float=w2018:sgl)
                      n1037 = To Single Precision Float(number=w2045) -> (single precision float=w2016:sgl)
                      n1038 = To Single Precision Float(number=w2033) -> (single precision float=w2021:sgl)
                      n1039 = To Single Precision Float(number=w2032) -> (single precision float=w2019:sgl)
                      n1040 = To Single Precision Float(number=w2029) -> (single precision float=w2014:sgl)
                      n1041 = To Single Precision Float(number=w2028) -> (single precision float=w2024:sgl)
                      n1042 = To Single Precision Float(number=w2027) -> (single precision float=w2023:sgl)
                      n1043 = To Single Precision Float(number=w2035) -> (single precision float=w2025:sgl)
                      n1044 = To Single Precision Float(number=w2048) -> (single precision float=w2022:sgl)
                      n1045 = To Single Precision Float(number=w2050) -> (single precision float=w2026:sgl)
                      n1046 = call "表格编辑.vi"("新元素/子数组"=w2059, "活动单元格:单元格背景色"=u32 6618880, "MCListbox引用句柄"=w2056) -> ()  [unwired: 9 out]
                      n1047 = property class="Clust (严格)"(reference=w2060) -> (reference out=w2063:refnum<vi>, "Value"=w2064:T10)  [unwired: 1 in, 1 out]
                      n1048 = Equal?(x=w2026, y=w2025) -> (x = y?=w2043:bool)
                      n1049 = Equal?(x=w2024, y=w2023) -> (x = y?=w2042:bool)
                      n1050 = Equal?(x=w2022, y=w2021) -> (x = y?=w2041:bool)
                      n1051 = Equal?(x=w2020, y=w2019) -> (x = y?=w2040:bool)
                      n1052 = Equal?(x=w2018, y=w2017) -> (x = y?=w2039:bool)
                      n1053 = Equal?(x=w2016, y=w2030) -> (x = y?=w2038:bool)
                      n1054 = Equal?(x=w2015, y=w2014) -> (x = y?=w2037:bool)
                      n1055 = Bundle By Name(cluster=w2064, "电压过高"=w2035, "电压过低"=w2027, "温度过高"=w2033, "温度过低"=w2032, "电压不均衡(V)"=w2031, "温度不均衡"=w2030, "SOC过低"=w2029) -> (w2062:T10)
                      n1056 = Compound Arithmetic op=AND(w2043, w2042, w2041, w2040, w2039, w2038, w2037) -> (w2036:bool)
                      n1057 = global write "EV05全局变量1.vi" "写入超时"(TRUE ("写入超时")) -> ()
                      n1058 = property class="Clust (严格)"(reference=w2063, "Value"=w2062) -> ()  [unwired: 1 in, 2 out]
                      n1059 = global write "读配置文件全局2.vi" "二级故障判定"(w2036) -> ()
                    }
                    frame 3 {
                      n1060 = Unbundle By Name(w2127) -> ("三级故障(从板)"=w2126:refnum<vi>)
                      n1061 = Index Array(array=w2147, index #1=0 ("长度")) -> (element #1=w2144:u8, element #2=w2145:u8, element #3=w2143:u8, element #4=w2142:u8, element #5=w2141:u8, element #6=w2140:u8, element #7=w2136:u8, element #8=w2135:u8, element #9=w2096:u8, element #10=w2121:u8, element #11=w2120:u8)  [unwired: 10 in]
                      n1062 = global read "读配置文件全局2.vi" "三级故障阀值"() -> (w2117:dbl[])
                      n1063 = Join Numbers(hi=w2144, lo=w2145) -> ((hi.lo)=w2139:u16)
                      n1064 = Join Numbers(hi=w2143, lo=w2142) -> ((hi.lo)=w2138:u16)
                      n1065 = Join Numbers(hi=w2141, lo=w2140) -> ((hi.lo)=w2132:u16)
                      n1066 = Join Numbers(hi=w2121, lo=w2120) -> ((hi.lo)=w2119:u16)
                      n1067 = call "输出分辨率计算.vi"("分辨率"=0.1, "数值 2"=w2119) -> ("输出2"=w2095:dbl)  [unwired: 4 in, 5 out]
                      n1068 = Index Array(array=w2117) -> (element #1=w2116:dbl, element #2=w2115:dbl, element #3=w2114:dbl, element #4=w2113:dbl, element #5=w2112:dbl, element #6=w2111:dbl, element #7=w2110:dbl)  [unwired: 7 in]
                      n1069 = call "输出分辨率计算.vi"("分辨率"=0.001, "数值 4"=w2132, "数值 3"=w2138, "数值 2"=w2139) -> ("输出4"=w2097:dbl, "输出3"=w2100:dbl, "输出2"=w2101:dbl)  [unwired: 2 in, 3 out]
                      n1070 = call "输出分辨率计算.vi"("偏移量"=sgl -40.0, "分辨率"=1.0, "数值 3"=w2135, "数值 2"=w2136) -> ("输出3"=w2098:dbl, "输出2"=w2099:dbl)  [unwired: 2 in, 4 out]
                      n1071 = Build Array("三级故障阀值     读取成功" ("字符串")) -> (w2125:string[])
                      n1072 = To Single Precision Float(number=w2110) -> (single precision float=w2083:sgl)
                      n1073 = To Single Precision Float(number=w2095) -> (single precision float=w2082:sgl)
                      n1074 = To Single Precision Float(number=w2113) -> (single precision float=w2088:sgl)
                      n1075 = To Single Precision Float(number=w2098) -> (single precision float=w2087:sgl)
                      n1076 = To Single Precision Float(number=w2112) -> (single precision float=w2086:sgl)
                      n1077 = To Single Precision Float(number=w2111) -> (single precision float=w2084:sgl)
                      n1078 = To Single Precision Float(number=w2097) -> (single precision float=w2085:sgl)
                      n1079 = To Single Precision Float(number=w2114) -> (single precision float=w2090:sgl)
                      n1080 = To Single Precision Float(number=w2099) -> (single precision float=w2089:sgl)
                      n1081 = To Single Precision Float(number=w2100) -> (single precision float=w2091:sgl)
                      n1082 = To Single Precision Float(number=w2116) -> (single precision float=w2094:sgl)
                      n1083 = To Single Precision Float(number=w2115) -> (single precision float=w2092:sgl)
                      n1084 = To Single Precision Float(number=w2101) -> (single precision float=w2093:sgl)
                      n1085 = call "表格编辑.vi"("新元素/子数组"=w2125, "活动单元格:单元格背景色"=u32 6618880, "MCListbox引用句柄"=w2122) -> ()  [unwired: 9 out]
                      n1086 = property class="Clust (严格)"(reference=w2126) -> (reference out=w2129:refnum<vi>, "Value"=w2130:T10)  [unwired: 1 in, 1 out]
                      n1087 = Equal?(x=w2094, y=w2093) -> (x = y?=w2109:bool)
                      n1088 = Equal?(x=w2092, y=w2091) -> (x = y?=w2108:bool)
                      n1089 = Equal?(x=w2090, y=w2089) -> (x = y?=w2107:bool)
                      n1090 = Equal?(x=w2088, y=w2087) -> (x = y?=w2106:bool)
                      n1091 = Equal?(x=w2086, y=w2085) -> (x = y?=w2105:bool)
                      n1092 = Equal?(x=w2084, y=w2096) -> (x = y?=w2104:bool)
                      n1093 = Equal?(x=w2083, y=w2082) -> (x = y?=w2103:bool)
                      n1094 = Bundle By Name(cluster=w2130, "电压过高"=w2101, "电压过低"=w2100, "温度过高"=w2099, "温度过低"=w2098, "电压不均衡(V)"=w2097, "温度不均衡"=w2096, "SOC过低"=w2095) -> (w2128:T10)
                      n1095 = global write "EV05全局变量1.vi" "写入超时"(TRUE ("写入超时")) -> ()
                      n1096 = Compound Arithmetic op=AND(w2109, w2108, w2107, w2106, w2105, w2104, w2103) -> (w2102:bool)
                      n1097 = property class="Clust (严格)"(reference=w2129, "Value"=w2128) -> ()  [unwired: 1 in, 2 out]
                      n1098 = global write "读配置文件全局2.vi" "三级故障判定"(w2102) -> ()
                    }
                  }
                }
                frame 3 {
                  n1099 = case shown="1" w2154 {
                    tunnel: w2153 -> [_ w2157 w2228 w2247 w2283 w2298 w2309 w2350]
                    tunnel: w2152 -> [_ w2158 w2231 w2245 w2280 w2294 w2306 w2336]
                    tunnel: [_ "电池组信息1     读取成功" ("字符串") "电池包组号     读取成功" ("字符串") "充放电安时     读取成功" ("字符串") "充电次数时间     读取成功" ("字符串") "SOC     读取成功" ("字符串") "车牌号     读取成功" ("字符串") "充电参数     读取成功" ("字符串")] -> w2148
                    frame 0, Default {
                    }
                    frame 1 {
                      w2199 = ":" ("字符串")
                      w2210 = "-" ("字符串")
                      n1100 = Unbundle By Name(w2158) -> ("电池组信息(从板)"=w2219:refnum<vi>)
                      n1101 = Reshape Array(w2157, 30 ("维数大小")) -> (w2220:u8[])
                      n1102 = Index Array(array=w2220) -> (element #1=w2217:u8, element #2=w2218:u8, element #3=w2167:u8, element #4=w2156:u8, element #5=w2155:u8, element #6=w2194:u8, element #7=w2193:u8, element #8=w2192:u8, element #9=w2191:u8, element #10=w2190:u8, element #11=w2189:u8, element #12=w2183:u8, element #13=w2182:u8, element #14=w2181:u8, element #15=w2180:u8, element #16=w2177:u8, element #17=w2176:u8, element #21=w2174:u8, element #22=w2173:u8, element #23=w2172:u8, element #24=w2171:u8, element #25=w2170:u8, element #26=w2169:u8)  [unwired: 26 in, 3 out]
                      n1103 = Join Numbers(hi=w2190, lo=w2189) -> ((hi.lo)=w2188:u16)
                      n1104 = Join Numbers(hi=w2217, lo=w2218) -> ((hi.lo)=w2168:u16)
                      n1105 = Join Numbers(hi=w2181, lo=w2180) -> ((hi.lo)=w2184:u16)
                      n1106 = Join Numbers(hi=w2177, lo=w2176) -> ((hi.lo)=w2175:u16)
                      n1107 = Join Numbers(hi=w2194, lo=w2193) -> ((hi.lo)=w2164:u16)
                      n1108 = Join Numbers(hi=w2192, lo=w2191) -> ((hi.lo)=w2187:u16)
                      n1109 = Join Numbers(hi=w2183, lo=w2182) -> ((hi.lo)=w2179:u16)
                      n1110 = Join Numbers(hi=w2187, lo=w2188) -> ((hi.lo)=w2186:u32)
                      n1111 = Join Numbers(hi=w2179, lo=w2184) -> ((hi.lo)=w2185:u32)
                      n1112 = To Double Precision Float(number=w2186) -> (double precision float=w2163:dbl)
                      n1113 = To Double Precision Float(number=w2185) -> (double precision float=w2162:dbl)
                      n1114 = call "输出分辨率计算.vi"("数值1"=w2164, "分辨率"=0.1, "数值 4"=w2175) -> ("输出4"=w2165:dbl, "输出1"=w2166:dbl)  [unwired: 3 in, 4 out]
                      n1115 = Number To Decimal String(number=w2174, width (-)=i16 2 ("宽度(-)")) -> (decimal integer string=w2212:string)
                      n1116 = Number To Decimal String(number=w2173, width (-)=i16 2 ("宽度(-)")) -> (decimal integer string=w2207:string)
                      n1117 = Number To Decimal String(number=w2171, width (-)=i16 2 ("宽度(-)")) -> (decimal integer string=w2200:string)
                      n1118 = Number To Decimal String(number=w2172, width (-)=i16 2 ("宽度(-)")) -> (decimal integer string=w2206:string)
                      n1119 = Number To Decimal String(number=w2170, width (-)=i16 2 ("宽度(-)")) -> (decimal integer string=w2204:string)
                      n1120 = Number To Decimal String(number=w2169, width (-)=i16 2 ("宽度(-)")) -> (decimal integer string=w2205:string)
                      n1121 = call "输出分辨率计算.vi"("分辨率"=0.001, "数值 3"=w2162, "数值 2"=w2163) -> ("输出3"=w2159:dbl, "输出2"=w2160:dbl)  [unwired: 3 in, 4 out]
                      n1122 = Concatenate Strings("20" ("字符串"), w2212, w2210, w2207, w2210, w2206) -> (w2198:string)
                      n1123 = Concatenate Strings(w2200, w2199, w2204, w2199, w2205) -> (w2197:string)
                      n1124 = call <vilib>:"Space Constant.vi"() -> ("String"=w2196:string)
                      n1125 = Concatenate Strings(w2198, w2196, w2197) -> (w2195:string)
                      n1126 = property class="Clust (严格)"(reference=w2219) -> (reference out=w2215:refnum<vi>, "Value"=w2216:T11)  [unwired: 1 in, 1 out]
                      n1127 = Bundle By Name(cluster=w2216, "串联数"=w2168, "并联数"=w2167, "电池厂家"=w2156, "电池类型"=w2155, "额定能量"=w2166, "额定容量"=w2160, "实际容量"=w2159, "额定总压"=w2165, "生产日期"=w2195) -> (w2214:T11)
                      n1128 = global write "EV05全局变量1.vi" "写入超时"(TRUE ("写入超时")) -> ()
                      n1129 = property class="Clust (严格)"(reference=w2215, "Value"=w2214) -> ()  [unwired: 1 in, 2 out]
                    }
                    frame 2 {
                      n1130 = Unbundle By Name(w2231) -> ("电池组信息(从板)"=w2230:refnum<vi>)
                      n1131 = Index Array(array=w2228, index #1=0 ("索引"), index #2=1 ("索引")) -> (element #1=w2236:u8, element #2=w2235:u8)  [unwired: 1 in, 1 out]
                      n1132 = Join Numbers(hi=w2236, lo=w2235) -> ((hi.lo)=w2229:u16)
                      n1133 = property class="Clust (严格)"(reference=w2230) -> (reference out=w2233:refnum<vi>, "Value"=w2234:T11)  [unwired: 1 in, 1 out]
                      n1134 = Bundle By Name(cluster=w2234, "电池包组号"=w2229) -> (w2232:T11)
                      n1135 = global write "EV05全局变量1.vi" "写入超时"(TRUE ("写入超时")) -> ()
                      n1136 = property class="Clust (严格)"(reference=w2233, "Value"=w2232) -> ()  [unwired: 1 in, 2 out]
                    }
                    frame 3 {
                      n1137 = Unbundle By Name(w2245) -> ("电池组信息(从板)"=w2244:refnum<vi>)
                      n1138 = Reshape Array(w2247, 8 ("维数大小")) -> (w2246:u8[])
                      n1139 = for {
                        N: 2 -> [_]
                        tunnel: w2246 -> [w2266]
                        tunnel: [w2251] -> w2248 mode=indexing
                        i -> [w2263]
                        n1140 = Multiply(x=w2263, y=4) -> (x*y=w2264:i32)
                        n1141 = Increment(x=w2264) -> (x+1=w2260:i32)
                        n1142 = Increment(x=w2260) -> (x+1=w2259:i32)
                        n1143 = Increment(x=w2259) -> (x+1=w2258:i32)
                        n1144 = Index Array(array=w2266, index #1=w2264, index #2=w2260, index #3=w2259, index #4=w2258) -> (element #1=w2262:u8, element #2=w2261:u8, element #3=w2257:u8, element #4=w2256:u8)
                        n1145 = Join Numbers(hi=w2262, lo=w2261) -> ((hi.lo)=w2254:u16)
                        n1146 = Join Numbers(hi=w2257, lo=w2256) -> ((hi.lo)=w2255:u16)
                        n1147 = Join Numbers(hi=w2254, lo=w2255) -> ((hi.lo)=w2252:u32)
                        n1148 = call "输出分辨率计算.vi"("分辨率"=0.001, "数值 2"=w2252) -> ("输出2"=w2251:dbl)  [unwired: 4 in, 5 out]
                      }
                      n1149 = Index Array(array=w2248) -> (element #1=w2242:dbl, element #2=w2241:dbl)  [unwired: 2 in]
                      n1150 = global write "EV05全局变量1.vi" "写入超时"(TRUE ("写入超时")) -> ()
                      n1151 = property class="Clust (严格)"(reference=w2244) -> (reference out=w2239:refnum<vi>, "Value"=w2243:T11)  [unwired: 1 in, 1 out]
                      n1152 = Bundle By Name(cluster=w2243, "充电总安时"=w2242, "放电总这时"=w2241) -> (w2240:T11)
                      n1153 = property class="Clust (严格)"(reference=w2239, "Value"=w2240) -> ()  [unwired: 1 in, 2 out]
                    }
                    frame 4 {
                      n1154 = Unbundle By Name(w2280) -> ("电池组信息(从板)"=w2276:refnum<vi>)
                      n1155 = Index Array(array=w2283) -> (element #1=w2281:u8, element #2=w2282:u8, element #3=w2274:u8, element #4=w2273:u8, element #5=w2272:u8, element #6=w2271:u8)  [unwired: 6 in]
                      n1156 = Join Numbers(hi=w2274, lo=w2273) -> ((hi.lo)=w2270:u16)
                      n1157 = Join Numbers(hi=w2272, lo=w2271) -> ((hi.lo)=w2269:u16)
                      n1158 = Join Numbers(hi=w2281, lo=w2282) -> ((hi.lo)=w2275:u16)
                      n1159 = property class="Clust (严格)"(reference=w2276) -> (reference out=w2278:refnum<vi>, "Value"=w2279:T11)  [unwired: 1 in, 1 out]
                      n1160 = Bundle By Name(cluster=w2279, "放空次数"=w2275, "充满次数"=w2270, "充电次数"=w2269) -> (w2277:T11)
                      n1161 = global write "EV05全局变量1.vi" "写入超时"(TRUE ("写入超时")) -> ()
                      n1162 = property class="Clust (严格)"(reference=w2278, "Value"=w2277) -> ()  [unwired: 1 in, 2 out]
                    }
                    frame 5 {
                      n1163 = Unbundle By Name(w2294) -> ("电池组信息(从板)"=w2290:refnum<vi>)
                      n1164 = Index Array(array=w2298, index #1=0 ("长度"), index #2=1 ("长度")) -> (element #1=w2285:u8, element #2=w2286:u8)
                      n1165 = Join Numbers(hi=w2285, lo=w2286) -> ((hi.lo)=w2284:u16)
                      n1166 = call "输出分辨率计算.vi"("分辨率"=0.1, "数值 2"=w2284) -> ("输出2"=w2289:dbl)  [unwired: 4 in, 5 out]
                      n1167 = global write "EV05全局变量1.vi" "写入超时"(TRUE ("写入超时")) -> ()
                      n1168 = property class="Clust (严格)"(reference=w2290) -> (reference out=w2292:refnum<vi>, "Value"=w2293:T11)  [unwired: 1 in, 1 out]
                      n1169 = Bundle By Name(cluster=w2293, "SOC"=w2289) -> (w2291:T11)
                      n1170 = property class="Clust (严格)"(reference=w2292, "Value"=w2291) -> ()  [unwired: 1 in, 2 out]
                    }
                    frame 6 {
                      n1171 = Unbundle By Name(w2306) -> ("电池组信息(从板)"=w2302:refnum<vi>)
                      n1172 = Array Subset(array=w2309, length=7 ("长度")) -> (w2307:u8[])  [unwired: 1 in]
                      n1173 = Byte Array To String(unsigned byte array=w2307) -> (string=w2301:string)
                      n1174 = property class="Clust (严格)"(reference=w2302) -> (reference out=w2304:refnum<vi>, "Value"=w2305:T11)  [unwired: 1 in, 1 out]
                      n1175 = Bundle By Name(cluster=w2305, "车牌号"=w2301) -> (w2303:T11)
                      n1176 = global write "EV05全局变量1.vi" "写入超时"(TRUE ("写入超时")) -> ()
                      n1177 = property class="Clust (严格)"(reference=w2304, "Value"=w2303) -> ()  [unwired: 1 in, 2 out]
                    }
                    frame 7 {
                      n1178 = Unbundle By Name(w2336) -> ("电池组信息(从板)"=w2335:refnum<vi>)
                      n1179 = Index Array(array=w2350) -> (element #1=w2348:u8, element #2=w2349:u8, element #3=w2346:u8, element #4=w2347:u8, element #5=w2328:u8, element #6=w2327:u8, element #7=w2345:u8, element #8=w2344:u8, element #9=w2320:u8, element #10=w2321:u8, element #11=w2318:u8, element #12=w2319:u8, element #13=w2317:u8, element #14=w2316:u8)  [unwired: 14 in]
                      n1180 = Join Numbers(hi=w2317, lo=w2316) -> ((hi.lo)=w2315:u16)
                      n1181 = Join Numbers(hi=w2320, lo=w2321) -> ((hi.lo)=w2312:u16)
                      n1182 = Join Numbers(hi=w2318, lo=w2319) -> ((hi.lo)=w2313:u16)
                      n1183 = Join Numbers(hi=w2348, lo=w2349) -> ((hi.lo)=w2343:u16)
                      n1184 = Join Numbers(hi=w2346, lo=w2347) -> ((hi.lo)=w2342:u16)
                      n1185 = Join Numbers(hi=w2345, lo=w2344) -> ((hi.lo)=w2339:u16)
                      n1186 = call "输出分辨率计算.vi"("分辨率"=0.001, "数值 3"=w2315, "数值 2"=w2343) -> ("输出3"=w2314:dbl, "输出2"=w2332:dbl)  [unwired: 3 in, 4 out]
                      n1187 = call "输出分辨率计算.vi"("分辨率"=0.1, "数值 2"=w2342) -> ("输出2"=w2331:dbl)  [unwired: 4 in, 5 out]
                      n1188 = call "输出分辨率计算.vi"("偏移量"=sgl 0.0, "分辨率"=0.1, "数值 3"=w2312, "数值 2"=w2339) -> ("输出3"=w2311:dbl, "输出2"=w2323:dbl)  [unwired: 2 in, 4 out]
                      n1189 = call "输出分辨率计算.vi"("偏移量"=sgl -40.0, "分辨率"=1.0, "数值 3"=w2327, "数值 2"=w2328) -> ("输出3"=w2325:dbl, "输出2"=w2326:dbl)  [unwired: 2 in, 4 out]
                      n1190 = global write "EV05全局变量1.vi" "写入超时"(TRUE ("写入超时")) -> ()
                      n1191 = property class="Clust (严格)"(reference=w2335) -> (reference out=w2324:refnum<vi>, "Value"=w2334:T11)  [unwired: 1 in, 1 out]
                      n1192 = Bundle By Name(cluster=w2334, "最大允许单体电压"=w2332, "最大允许总电压"=w2331, "最大允许温度"=w2326, "最小允许温度"=w2325, "最大允许充电电流"=w2323, "最小允许充电电流"=w2311, "电流步长"=w2313, "最小允许单体电压"=w2314) -> (w2333:T11)
                      n1193 = property class="Clust (严格)"(reference=w2324, "Value"=w2333) -> ()  [unwired: 1 in, 2 out]
                    }
                  }
                  n1194 = Build Array(w2148) -> (w2151:string[])
                  n1195 = call "表格编辑.vi"("新元素/子数组"=w2151, "活动单元格:单元格背景色"=u32 6618880, "MCListbox引用句柄"=w2149) -> ()  [unwired: 9 out]
                }
                frame 10 {
                  n1196 = Array Subset(array=w2352, length=30 ("长度")) -> (w2361:u8[])  [unwired: 1 in]
                  n1197 = Byte Array To String(unsigned byte array=w2361) -> (string=w2356:string)
                  n1198 = Concatenate Strings("BNET" ("字符串"), w2356) -> (w2355:string)
                  n1199 = property class="Str"(reference="从板二维码信息", "Text.Text"=w2355) -> ()  [unwired: 1 in, 2 out]
                  n1200 = global write "EV05全局变量1.vi" "写入超时"(TRUE ("写入超时")) -> ()
                  n1201 = Build Array("二维码     读取成功" ("字符串")) -> (w2359:string[])
                  n1202 = call "表格编辑.vi"("新元素/子数组"=w2359, "活动单元格:单元格背景色"=u32 6618880, "MCListbox引用句柄"=w2351) -> ()  [unwired: 9 out]
                }
                frame 6 {
                  n1203 = case shown="2" w2369 {
                    tunnel: w2368 -> [_ w2397 w2452]
                    tunnel: w2367 -> [_ w2398 w2453]
                    tunnel: [_ "均衡阀值     读取成功" ("字符串") "充电结束电压     读取成功" ("字符串")] -> w2363
                    frame 0, Default {
                    }
                    frame 1 {
                      w2380 = 0.001 ("分辨率")
                      n1204 = Reshape Array(w2397, 24 ("维数大小")) -> (w2405:u8[])
                      n1205 = Unbundle By Name(w2398) -> ("均衡参数"=w2404:refnum<vi>)
                      n1206 = Index Array(array=w2405) -> (element #1=w2402:u8, element #2=w2403:u8, element #3=w2396:u8, element #4=w2395:u8, element #5=w2394:u8, element #6=w2393:u8, element #7=w2392:u8, element #8=w2391:u8, element #9=w2390:u8, element #10=w2389:u8, element #11=w2388:u8, element #12=w2387:u8, element #13=w2386:u8, element #14=w2385:u8)  [unwired: 14 in]
                      n1207 = Join Numbers(hi=w2402, lo=w2403) -> ((hi.lo)=w2384:u16)
                      n1208 = Join Numbers(hi=w2396, lo=w2395) -> ((hi.lo)=w2383:u16)
                      n1209 = Join Numbers(hi=w2394, lo=w2393) -> ((hi.lo)=w2382:u16)
                      n1210 = Join Numbers(hi=w2392, lo=w2391) -> ((hi.lo)=w2381:u16)
                      n1211 = Join Numbers(hi=w2390, lo=w2389) -> ((hi.lo)=w2379:u16)
                      n1212 = Join Numbers(hi=w2388, lo=w2387) -> ((hi.lo)=w2378:u16)
                      n1213 = Join Numbers(hi=w2386, lo=w2385) -> ((hi.lo)=w2377:u16)
                      n1214 = call "输出分辨率计算.vi"("分辨率"=w2380, "数值 4"=w2377, "数值 3"=w2378, "数值 2"=w2379) -> ("输出4"=w2370:dbl, "输出3"=w2371:dbl, "输出2"=w2372:dbl)  [unwired: 2 in, 3 out]
                      n1215 = call "输出分辨率计算.vi"("数值1"=w2384, "分辨率"=w2380, "数值 4"=w2381, "数值 3"=w2382, "数值 2"=w2383) -> ("输出4"=w2373:dbl, "输出3"=w2374:dbl, "输出2"=w2375:dbl, "输出1"=w2376:dbl)  [unwired: 1 in, 2 out]
                      n1216 = property class="Clust (严格)"(reference=w2404) -> (reference out=w2400:refnum<vi>, "Value"=w2401:T12)  [unwired: 1 in, 1 out]
                      n1217 = Bundle By Name(cluster=w2401, "均衡计算-电压高阀值2级"=w2376, "均衡计算-电压高阀值1级"=w2375, "均衡计算-电压低阀值1级"=w2374, "均衡计算-电压低阀值2级"=w2373, "均衡计算-最低电压阀值"=w2372, "均衡停止-最低电压阀值"=w2371, "均衡计算-电压极差阀值"=w2370) -> (w2399:T12)
                      n1218 = global write "EV05全局变量1.vi" "写入超时"(TRUE ("写入超时")) -> ()
                      n1219 = property class="Clust (严格)"(reference=w2400, "Value"=w2399) -> ()  [unwired: 1 in, 2 out]
                    }
                    frame 2 {
                      w2417 = 0.001 ("分辨率")
                      n1220 = Reshape Array(w2452, 22 ("维数大小")) -> (w2460:u8[])
                      n1221 = Unbundle By Name(w2453) -> ("均衡参数"=w2459:refnum<vi>)
                      n1222 = Index Array(array=w2460) -> (element #1=w2457:u8, element #2=w2458:u8, element #3=w2451:u8, element #4=w2450:u8, element #5=w2449:u8, element #6=w2448:u8, element #7=w2447:u8, element #8=w2446:u8, element #9=w2445:u8, element #10=w2444:u8, element #11=w2443:u8, element #12=w2442:u8, element #13=w2441:u8, element #14=w2440:u8, element #15=w2425:u8, element #16=w2424:u8, element #17=w2423:u8, element #18=w2422:u8, element #19=w2421:u8, element #20=w2420:u8, element #21=w2419:u8, element #22=w2418:u8)  [unwired: 22 in]
                      n1223 = Join Numbers(hi=w2457, lo=w2458) -> ((hi.lo)=w2439:u16)
                      n1224 = Join Numbers(hi=w2451, lo=w2450) -> ((hi.lo)=w2438:u16)
                      n1225 = Join Numbers(hi=w2449, lo=w2448) -> ((hi.lo)=w2437:u16)
                      n1226 = Join Numbers(hi=w2447, lo=w2446) -> ((hi.lo)=w2436:u16)
                      n1227 = Join Numbers(hi=w2445, lo=w2444) -> ((hi.lo)=w2435:u16)
                      n1228 = Join Numbers(hi=w2443, lo=w2442) -> ((hi.lo)=w2434:u16)
                      n1229 = Join Numbers(hi=w2441, lo=w2440) -> ((hi.lo)=w2433:u16)
                      n1230 = Join Numbers(hi=w2425, lo=w2424) -> ((hi.lo)=w2416:u16)
                      n1231 = Join Numbers(hi=w2423, lo=w2422) -> ((hi.lo)=w2415:u16)
                      n1232 = Join Numbers(hi=w2421, lo=w2420) -> ((hi.lo)=w2414:u16)
                      n1233 = Join Numbers(hi=w2419, lo=w2418) -> ((hi.lo)=w2413:u16)
                      n1234 = call "输出分辨率计算.vi"("数值1"=w2416, "分辨率"=w2417, "数值 4"=w2413, "数值 3"=w2414, "数值 2"=w2415) -> ("输出4"=w2409:dbl, "输出3"=w2410:dbl, "输出2"=w2411:dbl, "输出1"=w2412:dbl)  [unwired: 1 in, 2 out]
                      n1235 = call "输出分辨率计算.vi"("分辨率"=w2417, "数值 4"=w2433, "数值 3"=w2434, "数值 2"=w2435) -> ("输出4"=w2426:dbl, "输出3"=w2427:dbl, "输出2"=w2428:dbl)  [unwired: 2 in, 3 out]
                      n1236 = call "输出分辨率计算.vi"("数值1"=w2439, "分辨率"=w2417, "数值 4"=w2436, "数值 3"=w2437, "数值 2"=w2438) -> ("输出4"=w2429:dbl, "输出3"=w2430:dbl, "输出2"=w2431:dbl, "输出1"=w2432:dbl)  [unwired: 1 in, 2 out]
                      n1237 = property class="Clust (严格)"(reference=w2459) -> (reference out=w2455:refnum<vi>, "Value"=w2456:T12)  [unwired: 1 in, 1 out]
                      n1238 = Bundle By Name(cluster=w2456, "充电结束电压(90%)"=w2432, "充电结束电压(91%)"=w2431, "充电结束电压(92%)"=w2430, "充电结束电压(93%)"=w2429, "充电结束电压(94%)"=w2428, "充电结束电压(95%)"=w2427, "充电结束电压(96%)"=w2426, "充电结束电压(97%)"=w2412, "充电结束电压(98%)"=w2411, "充电结束电压(99%)"=w2410, "充电结束电压(100%)"=w2409) -> (w2454:T12)
                      n1239 = global write "EV05全局变量1.vi" "写入超时"(TRUE ("写入超时")) -> ()
                      n1240 = property class="Clust (严格)"(reference=w2455, "Value"=w2454) -> ()  [unwired: 1 in, 2 out]
                    }
                  }
                  n1241 = Build Array(w2363) -> (w2366:string[])
                  n1242 = call "表格编辑.vi"("新元素/子数组"=w2366, "活动单元格:单元格背景色"=u32 6618880, "MCListbox引用句柄"=w2364) -> ()  [unwired: 9 out]
                }
              }
            }
            frame True {
            }
          }
        }
      }
    }
  }
  n1243 = disable-structure shown="禁用" {
    frame Disabled {
      n1244 = global read "读配置文件全局2.vi" "表格"() -> (w2470:string[])
      n1245 = Array Subset(array=w2470, index=0 ("索引"), length=2 ("长度")) -> (w2467:string[])
      n1246 = for {
        tunnel: w2467 -> [w2472] mode=indexing
        tunnel: [w2471] -> w2466 mode=indexing
        n1247 = Fract/Exp String To Number(string=w2472) -> (number=w2471:dbl)  [unwired: 4 out]
      }
      n1248 = Equal?(y=w2466) -> (x = y?=w2465:bool[])  [unwired: 1 in]
      n1249 = And Array Elements(Boolean array=w2465) -> (logical AND=w2464:bool)
      n1250 = global write "读配置文件全局2.vi" "电压起始值判定"(w2464) -> ()
    }
    frame Enabled {
    }
  }
